vi "CPT32 Pulse Gen 3 (FPGA).vi"() -> ()   [LabVIEW 2021]
uses:
  <vilib>/rvi/Emulation/niFpgaGetClockAttributes.vi
  <vilib>/rvi/Emulation/niFpgaSctlEmulationGetInTimedLoop.vi
  <vilib>/rvi/Emulation/niFpgaEmulationReportErrorSimple.vi
  <vilib>/rvi/Emulation/niFpgaProcessEmulError.vi
  <vilib>/rvi/eio/common/nirviEmuTemplateMethod_errors.vi
  <vilib>/rvi/Emulation/niFpgaCriticalErrorInLSC.vi
  <vilib>/eio/EIOMethodNode/EIOMethodNode.xnode
  <vilib>/eio/EIONode/EIONode.xnode
panel:
  out "Array 7":fxp<+/-,37,27>[](array[numeric])
  out "Array 6":fxp<+/-,37,27>[](array[numeric])
  out "Array 5":fxp<+/-,37,27>[](array[numeric])
  out "Array 4":fxp<+/-,37,27>[](array[numeric])=[20.0, -50.0, 10.0, 20.0, 0.0, 0.0, 0.0, 0.0, 0.0, 0.0, 0.0, 0.0, 0.0, 0.0, 0.0, 0.0, 0.0, 0.0, 0.0, 0.0, 0.0, 0.0, 0.0, 0.0, 0.0, 0.0, 0.0, 0.0, 0.0, 0.0, 0.0, 0.0]
  out "Array 2":fxp<+/-,37,27>[](array[numeric])
  out "Array 1":fxp<+/-,37,27>[](array[numeric])
  out "Array 0":fxp<+/-,37,27>[](array[numeric])
  out "Array 3":fxp<+/-,37,27>[](array[numeric])=[20.0, -10.0, 50.0, -10.0, 0.0, 0.0, 0.0, 0.0, 0.0, 0.0, 0.0, 0.0, 0.0, 0.0, 0.0, 0.0]
  in  "Period (ms)":fxp<+,21,11>=160.0
  in  "DO 4":fxp<+/-,21,11>[](array[numeric])=[10.0, -10.0, 10.0, -10.0, 10.0, -10.0, 10.0, -10.0, 10.0, -10.0, 10.0, -10.0, 10.0, -10.0, 10.0, -10.0, 0.0, 0.0, 0.0, 0.0, 0.0, 0.0, 0.0, 0.0, 0.0, 0.0, 0.0, 0.0, 0.0, 0.0, 0.0, 0.0] format="%#.4g"
  in  "DO 2":fxp<+/-,21,11>[](array[numeric])=[10.0, -10.0, 10.0, -10.0, 10.0, -10.0, 10.0, -10.0, 10.0, -10.0, 10.0, -10.0, 10.0, -10.0, 10.0, -10.0] format="%#.4g"
  in  "DO 1":fxp<+/-,21,11>[](array[numeric])=[10.0, -10.0, 10.0, -10.0, 10.0, -10.0, 10.0, -10.0, 10.0, -10.0, 10.0, -10.0, 10.0, -10.0, 10.0, -10.0, 0.0, 0.0, 0.0, 0.0, 0.0, 0.0, 0.0, 0.0, 0.0, 0.0, 0.0, 0.0, 0.0, 0.0, 0.0, 0.0] format="%#.4g"
  in  "DO 3":fxp<+/-,21,11>[](array[numeric])=[0.0009765625, -10.0, -10.0, -10.0, -10.0, -10.0, -10.0, -10.0, -10.0, -10.0, -10.0, -10.0, -10.0, -10.0, -10.0, -10.0] format="%#.4g"
  in  "DO 5":fxp<+/-,21,11>[](array[numeric])=[10.0, -10.0, 10.0, -10.0, 10.0, -10.0, 10.0, -10.0, 10.0, -10.0, 10.0, -10.0, 10.0, -10.0, 10.0, -10.0, 0.0, 0.0, 0.0, 0.0, 0.0, 0.0, 0.0, 0.0, 0.0, 0.0, 0.0, 0.0, 0.0, 0.0, 0.0, 0.0] format="%#.4g"
  in  "DO 6":fxp<+/-,21,11>[](array[numeric])=[10.0, -10.0, 10.0, -10.0, 10.0, -10.0, 10.0, -10.0, 10.0, -10.0, 10.0, -10.0, 10.0, -10.0, 10.0, -10.0, 0.0, 0.0, 0.0, 0.0, 0.0, 0.0, 0.0, 0.0, 0.0, 0.0, 0.0, 0.0, 0.0, 0.0, 0.0, 0.0] format="%#.4g"
  in  "DO 7":fxp<+/-,21,11>[](array[numeric])=[10.0, -10.0, -10.0, -10.0, -10.0, -10.0, -10.0, -10.0, -10.0, -10.0, -10.0, -10.0, -10.0, -10.0, -10.0, -10.0, 0.0, 0.0, 0.0, 0.0, 0.0, 0.0, 0.0, 0.0, 0.0, 0.0, 0.0, 0.0, 0.0, 0.0, 0.0, 0.0] format="%#.4g"
  in  "DO 0":fxp<+/-,21,11>[](array[numeric])=[0.0, 0.0, 0.0, 0.0, 0.0, 0.0, 0.0, 0.0, 0.0, 0.0, 0.0, 0.0, 0.0, 0.0, 0.0, 0.0] format="%#.4g"
  out "Period (us)":fxp<+/-,37,27>
  in  "Stop":bool
  out "AO 0 t":fxp<+/-,37,27>[](array[numeric])
  in  "Start":bool
  out "AO 1 t":fxp<+/-,37,27>[](array[numeric])
  out "AO 2 t":fxp<+/-,37,27>[](array[numeric])
  out "AO 3 t":fxp<+/-,37,27>[](array[numeric])
  in  "AO 0 time":fxp<+/-,21,11>[](array[numeric])=[0.0, 0.0, 0.0, 0.0, 0.0, 0.0, 0.0, 0.0, 0.0, 0.0, 0.0, 0.0, 0.0, 0.0, 0.0, 0.0] format="%#.4g"
  in  "AO 0 voltage":fxp<+/-,32,6>[](array[numeric])=[0.0, 0.0, 0.0, 0.0, 0.0, 0.0, 0.0, 0.0, 0.0, 0.0, 0.0, 0.0, 0.0, 0.0, 0.0, 0.0]
  in  "AO 1 time":fxp<+/-,21,11>[](array[numeric])=[0.0, 0.0, 0.0, 0.0, 0.0, 0.0, 0.0, 0.0, 0.0, 0.0, 0.0, 0.0, 0.0, 0.0, 0.0, 0.0] format="%#.4g"
  in  "AO 1 voltage":fxp<+/-,32,6>[](array[numeric])=[0.0, 0.0, 0.0, 0.0, 0.0, 0.0, 0.0, 0.0, 0.0, 0.0, 0.0, 0.0, 0.0, 0.0, 0.0, 0.0]
  in  "AO 2 time":fxp<+/-,21,11>[](array[numeric])=[0.0, 0.0, 0.0, 0.0] format="%#.4g"
  in  "AO 2 voltage":fxp<+/-,32,6>[](array[numeric])=[0.0, 0.0, 0.0, 0.0]
  in  "AO 3 time":fxp<+/-,21,11>[](array[numeric])=[0.0, 0.0, 0.0, 0.0] format="%#.4g"
  in  "AO 3 voltage":fxp<+/-,32,6>[](array[numeric])=[0.0, 0.0, 0.0, 0.0]
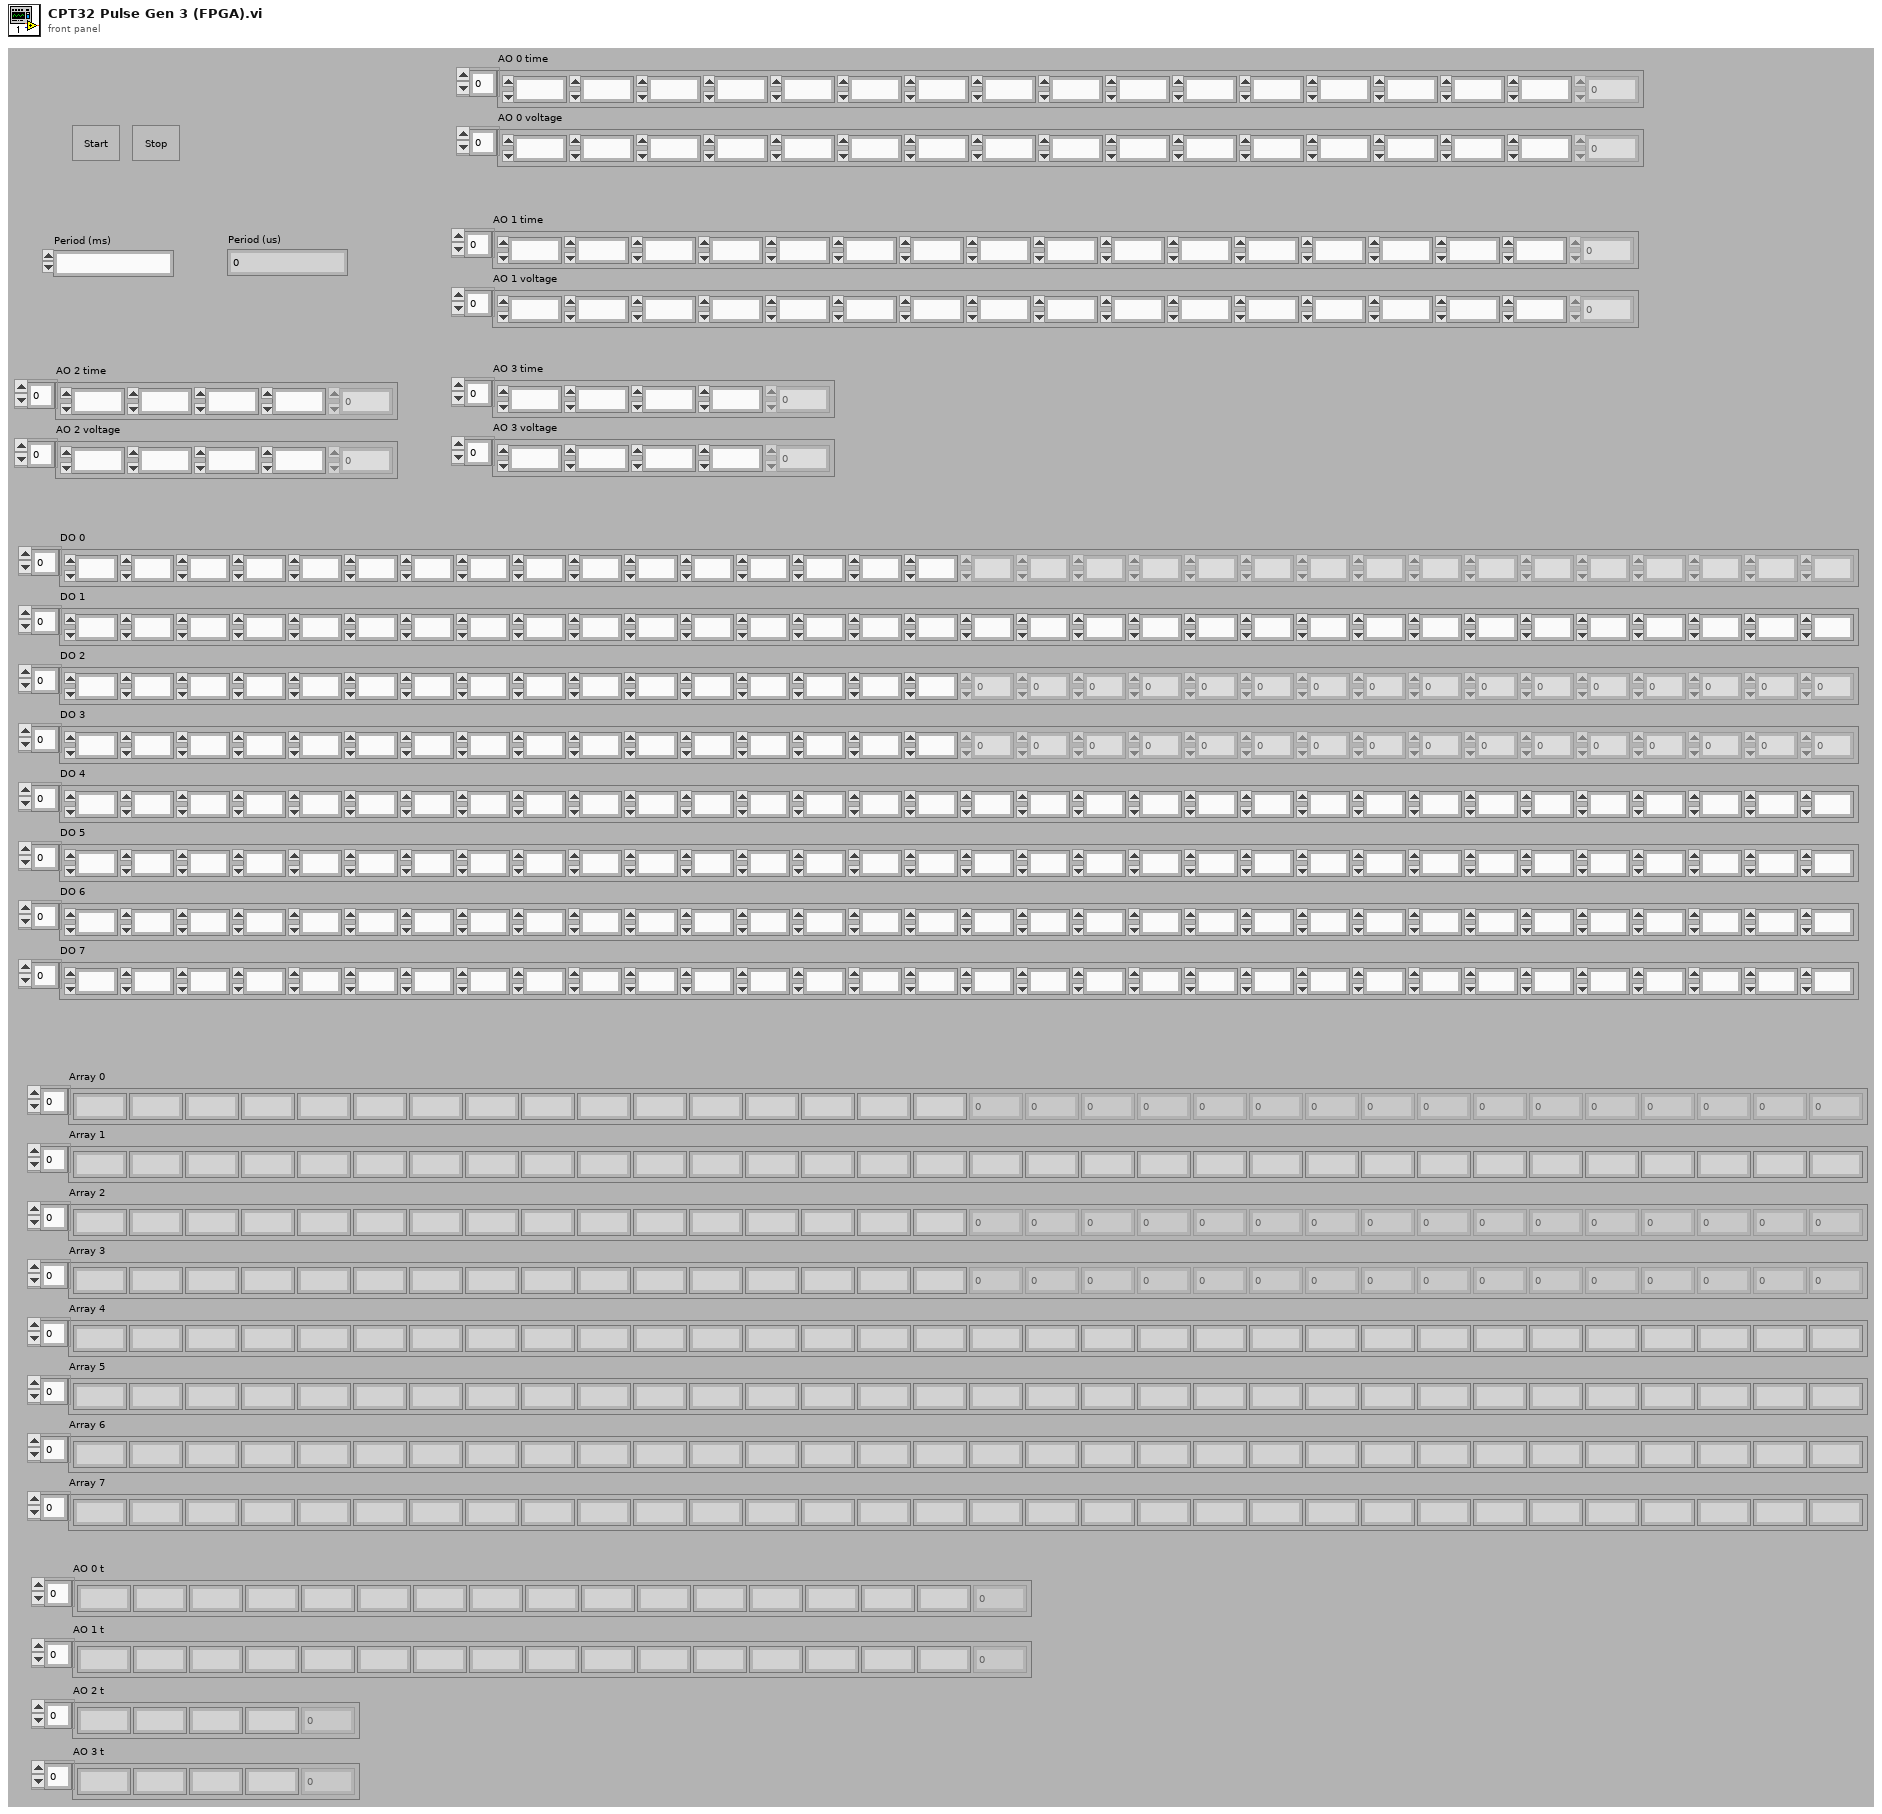
[diagram p1: front panel]
diagram:
  n1 = while {
    stop <- FALSE stop-if-true
    n2 = case shown="True" "Start" {
      frame False {
      }
      frame True {
        w4 = FALSE
        w3 = i16 0
        n3 = xnode "FPGA I/O Node"("Connector0/DIO0"=w4, "Connector0/DIO1"=w4, "Connector0/DIO2"=w4, "Connector0/DIO3"=w4, "Connector0/DIO4"=w4, "Connector0/DIO5"=w4, "Connector0/DIO6"=w4, "Connector0/DIO7"=w4, "Connector0/AO0"=w3, "Connector0/AO1"=w3, "Connector0/AO2"=w3, "Connector0/AO3"=w3) -> ()  [unwired: 12 in, 12 out]
        n4 = while {
          stop <- "Stop" stop-if-true
          n5 = Multiply(x="DO 3", y=i16 1000) -> (x*y=→"Array 3":fxp<+/-,37,27>[])
          n6 = Multiply(x="DO 4", y=i16 1000) -> (x*y=→"Array 4":fxp<+/-,37,27>[])
          n7 = Multiply(x="DO 5", y=i16 1000) -> (x*y=→"Array 5":fxp<+/-,37,27>[])
          n8 = Multiply(x="DO 6", y=i16 1000) -> (x*y=→"Array 6":fxp<+/-,37,27>[])
          n9 = Multiply(x="DO 7", y=i16 1000) -> (x*y=→"Array 7":fxp<+/-,37,27>[])
          n10 = Multiply(x="DO 0", y=i16 1000) -> (x*y=→"Array 0":fxp<+/-,37,27>[])
          n11 = Multiply(x="DO 1", y=i16 1000) -> (x*y=→"Array 1":fxp<+/-,37,27>[])
          n12 = Multiply(x="DO 2", y=i16 1000) -> (x*y=→"Array 2":fxp<+/-,37,27>[])
          n13 = Multiply(x="AO 0 time", y=i16 1000) -> (x*y=→"AO 0 t":fxp<+/-,37,27>[])
          n14 = Multiply(x="AO 3 time", y=i16 1000) -> (x*y=→"AO 3 t":fxp<+/-,37,27>[])
          n15 = Multiply(x="AO 1 time", y=i16 1000) -> (x*y=→"AO 1 t":fxp<+/-,37,27>[])
          n16 = Multiply(x="AO 2 time", y=i16 1000) -> (x*y=→"AO 2 t":fxp<+/-,37,27>[])
          n17 = Multiply(x="Period (ms)", y=i16 1000) -> (x*y=→"Period (us)":fxp<+/-,37,27>)
          n18 = flat-sequence {
            frame #0 {
              n19 = xnode "FPGA I/O Method Node"("Timeout"=-1) -> ()  [unwired: 1 in, 2 out]
            }
            frame #1 {
              n20 = local read "Period (us)"() -> (w126:fxp<+/-,37,27>)
              n21 = flat-sequence "Channel 0" {
                frame #0 {
                  # "第一段电压大小"
                  n22 = local read "AO 2 voltage"() -> (w281:fxp<+/-,32,6>[])
                  n23 = Index Array(array=w281, index=0) -> (element=w279:fxp<+/-,32,6>)
                  n24 = xnode "FPGA I/O Node"("Connector0/AO2"=w279) -> ()  [unwired: 1 in, 1 out]
                }
                frame #1 {
                  # "第一段持续时间"
                  n25 = local read "AO 2 t"() -> (w284:fxp<+/-,37,27>[])
                  n26 = Index Array(array=w284, index=0) -> (element=w282:fxp<+/-,37,27>)
                  n27 = call "Wait9"("Count(uSec)"=w282) -> ()  [unwired: 1 out]
                }
                frame #2 {
                  # "第二段电压大小"
                  n28 = local read "AO 2 voltage"() -> (w286:fxp<+/-,32,6>[])
                  n29 = Index Array(array=w286, index=1) -> (element=w285:fxp<+/-,32,6>)
                  n30 = xnode "FPGA I/O Node"("Connector0/AO2"=w285) -> ()  [unwired: 1 in, 1 out]
                }
                frame #3 {
                  # "第二段持续时间"
                  n31 = local read "AO 2 t"() -> (w289:fxp<+/-,37,27>[])
                  n32 = Index Array(array=w289, index=1) -> (element=w288:fxp<+/-,37,27>)
                  n33 = call "Wait10"("Count(uSec)"=w288) -> ()  [unwired: 1 out]
                }
                frame #4 {
                  # "第三段电压大小"
                  n34 = local read "AO 2 voltage"() -> (w292:fxp<+/-,32,6>[])
                  n35 = Index Array(array=w292, index=2) -> (element=w291:fxp<+/-,32,6>)
                  n36 = xnode "FPGA I/O Node"("Connector0/AO2"=w291) -> ()  [unwired: 1 in, 1 out]
                }
                frame #5 {
                  # "第三段持续时间"
                  n37 = local read "AO 2 t"() -> (w296:fxp<+/-,37,27>[])
                  n38 = Index Array(array=w296, index=2) -> (element=w294:fxp<+/-,37,27>)
                  n39 = call "Wait11"("Count(uSec)"=w294) -> ()  [unwired: 1 out]
                }
                frame #6 {
                  # "第四段电压大小"
                  n40 = local read "AO 2 voltage"() -> (w299:fxp<+/-,32,6>[])
                  n41 = Index Array(array=w299, index=3) -> (element=w297:fxp<+/-,32,6>)
                  n42 = xnode ("FPGA I/O Node")("Connector0/AO2"=w297) -> ()  [unwired: 1 in, 1 out]
                }
                frame #7 {
                  # "第四段持续时间"
                  n43 = local read "AO 2 t"() -> (w301:fxp<+/-,37,27>[])
                  n44 = Index Array(array=w301, index=3) -> (element=w300:fxp<+/-,37,27>)
                  n45 = call "Wait12"("Count(uSec)"=w300) -> ()  [unwired: 1 out]
                }
              }
              n46 = flat-sequence "Channel 0" {
                frame #0 {
                  # "第一段电压大小"
                  n47 = local read "AO 3 voltage"() -> (w257:fxp<+/-,32,6>[])
                  n48 = Index Array(array=w257, index=0) -> (element=w255:fxp<+/-,32,6>)
                  n49 = xnode "FPGA I/O Node"("Connector0/AO3"=w255) -> ()  [unwired: 1 in, 1 out]
                }
                frame #1 {
                  # "第一段持续时间"
                  n50 = local read "AO 3 t"() -> (w260:fxp<+/-,37,27>[])
                  n51 = Index Array(array=w260, index=0) -> (element=w258:fxp<+/-,37,27>)
                  n52 = call "Wait13"("Count(uSec)"=w258) -> ()  [unwired: 1 out]
                }
                frame #2 {
                  # "第二段电压大小"
                  n53 = local read "AO 3 voltage"() -> (w262:fxp<+/-,32,6>[])
                  n54 = Index Array(array=w262, index=1) -> (element=w261:fxp<+/-,32,6>)
                  n55 = xnode "FPGA I/O Node"("Connector0/AO3"=w261) -> ()  [unwired: 1 in, 1 out]
                }
                frame #3 {
                  # "第二段持续时间"
                  n56 = local read "AO 3 t"() -> (w265:fxp<+/-,37,27>[])
                  n57 = Index Array(array=w265, index=1) -> (element=w264:fxp<+/-,37,27>)
                  n58 = call "Wait14"("Count(uSec)"=w264) -> ()  [unwired: 1 out]
                }
                frame #4 {
                  # "第三段电压大小"
                  n59 = local read "AO 3 voltage"() -> (w268:fxp<+/-,32,6>[])
                  n60 = Index Array(array=w268, index=2) -> (element=w267:fxp<+/-,32,6>)
                  n61 = xnode "FPGA I/O Node"("Connector0/AO3"=w267) -> ()  [unwired: 1 in, 1 out]
                }
                frame #5 {
                  # "第三段持续时间"
                  n62 = local read "AO 3 t"() -> (w272:fxp<+/-,37,27>[])
                  n63 = Index Array(array=w272, index=2) -> (element=w270:fxp<+/-,37,27>)
                  n64 = call "Wait15"("Count(uSec)"=w270) -> ()  [unwired: 1 out]
                }
                frame #6 {
                  # "第四段电压大小"
                  n65 = local read "AO 3 voltage"() -> (w275:fxp<+/-,32,6>[])
                  n66 = Index Array(array=w275, index=3) -> (element=w273:fxp<+/-,32,6>)
                  n67 = xnode ("FPGA I/O Node")("Connector0/AO3"=w273) -> ()  [unwired: 1 in, 1 out]
                }
                frame #7 {
                  # "第四段持续时间"
                  n68 = local read "AO 3 t"() -> (w277:fxp<+/-,37,27>[])
                  n69 = Index Array(array=w277, index=3) -> (element=w276:fxp<+/-,37,27>)
                  n70 = call "Wait16"("Count(uSec)"=w276) -> ()  [unwired: 1 out]
                }
              }
              n71 = flat-sequence "Channel 3" {
                tunnel: [w1648] -> w254
                tunnel: w254 -> [w1652]
                tunnel: [w1653] -> w253
                tunnel: w253 -> [w1658]
                tunnel: [w1660] -> w252
                tunnel: w252 -> [w1664]
                tunnel: [w1666] -> w251
                tunnel: w251 -> [w1670]
                tunnel: [w1672] -> w250
                tunnel: w250 -> [w1676]
                tunnel: [w1678] -> w249
                tunnel: w249 -> [w1682]
                tunnel: [w1684] -> w248
                tunnel: w248 -> [w1688]
                tunnel: [w1690] -> w247
                tunnel: w247 -> [w1694]
                tunnel: [w1695] -> w246
                tunnel: w246 -> [w1700]
                tunnel: [w1701] -> w245
                tunnel: w245 -> [w1706]
                tunnel: [w1708] -> w244
                tunnel: w244 -> [w1712]
                tunnel: [w1714] -> w243
                tunnel: w243 -> [w1718]
                tunnel: [w1720] -> w242
                tunnel: w242 -> [w1724]
                tunnel: [w1726] -> w241
                tunnel: w241 -> [w1730]
                tunnel: [w1732] -> w240
                tunnel: w240 -> [w1736]
                tunnel: [w1738] -> w239
                tunnel: w239 -> [w1742]
                frame #0 {
                  # "起始电平"
                  n72 = local read "Array 0"() -> (w1650:fxp<+/-,37,27>[])
                  n73 = Index Array(array=w1650, index=0) -> (element=w1648:fxp<+/-,37,27>)
                  n74 = Greater Than 0?(x=w1648) -> (x > 0?=w1647:bool)
                  n75 = xnode "FPGA I/O Node"("Connector0/DIO0"=w1647) -> ()  [unwired: 1 in, 1 out]
                }
                frame #1 {
                  # "第一段持续时间"
                  n76 = Absolute Value(x=w1652) -> (abs(x)=w1651:fxp<+,36,26>)
                  n77 = call "Wait17"("Count(uSec)"=w1651) -> ()  [unwired: 1 out]
                }
                frame #2 {
                  n78 = local read "Array 0"() -> (w1656:fxp<+/-,37,27>[])
                  n79 = Index Array(array=w1656, index=1) -> (element=w1653:fxp<+/-,37,27>)
                  n80 = Greater Than 0?(x=w1653) -> (x > 0?=w1654:bool)
                  n81 = xnode "FPGA I/O Node"("Connector0/DIO0"=w1654) -> ()  [unwired: 1 in, 1 out]
                }
                frame #3 {
                  n82 = Absolute Value(x=w1658) -> (abs(x)=w1657:fxp<+,36,26>)
                  n83 = call "Wait18"("Count(uSec)"=w1657) -> ()  [unwired: 1 out]
                }
                frame #4 {
                  n84 = local read "Array 0"() -> (w1662:fxp<+/-,37,27>[])
                  n85 = Index Array(array=w1662, index=2) -> (element=w1660:fxp<+/-,37,27>)
                  n86 = Greater Than 0?(x=w1660) -> (x > 0?=w1659:bool)
                  n87 = xnode "FPGA I/O Node"("Connector0/DIO0"=w1659) -> ()  [unwired: 1 in, 1 out]
                }
                frame #5 {
                  n88 = Absolute Value(x=w1664) -> (abs(x)=w1663:fxp<+,36,26>)
                  n89 = call "Wait19"("Count(uSec)"=w1663) -> ()  [unwired: 1 out]
                }
                frame #6 {
                  n90 = local read "Array 0"() -> (w1668:fxp<+/-,37,27>[])
                  n91 = Index Array(array=w1668, index=3) -> (element=w1666:fxp<+/-,37,27>)
                  n92 = Greater Than 0?(x=w1666) -> (x > 0?=w1665:bool)
                  n93 = xnode ("FPGA I/O Node")("Connector0/DIO0"=w1665) -> ()  [unwired: 1 in, 1 out]
                }
                frame #7 {
                  n94 = Absolute Value(x=w1670) -> (abs(x)=w1669:fxp<+,36,26>)
                  n95 = call "Wait20"("Count(uSec)"=w1669) -> ()  [unwired: 1 out]
                }
                frame #8 {
                  # "低"
                  n96 = local read "Array 0"() -> (w1674:fxp<+/-,37,27>[])
                  n97 = Index Array(array=w1674, index=4) -> (element=w1672:fxp<+/-,37,27>)
                  n98 = Greater Than 0?(x=w1672) -> (x > 0?=w1671:bool)
                  n99 = xnode "FPGA I/O Node"("Connector0/DIO0"=w1671) -> ()  [unwired: 1 in, 1 out]
                }
                frame #9 {
                  n100 = Absolute Value(x=w1676) -> (abs(x)=w1675:fxp<+,36,26>)
                  n101 = call "Wait21"("Count(uSec)"=w1675) -> ()  [unwired: 1 out]
                }
                frame #10 {
                  # "高"
                  n102 = local read "Array 0"() -> (w1680:fxp<+/-,37,27>[])
                  n103 = Index Array(array=w1680, index=5) -> (element=w1678:fxp<+/-,37,27>)
                  n104 = Greater Than 0?(x=w1678) -> (x > 0?=w1677:bool)
                  n105 = xnode "FPGA I/O Node"("Connector0/DIO0"=w1677) -> ()  [unwired: 1 in, 1 out]
                }
                frame #11 {
                  n106 = Absolute Value(x=w1682) -> (abs(x)=w1681:fxp<+,36,26>)
                  n107 = call "Wait22"("Count(uSec)"=w1681) -> ()  [unwired: 1 out]
                }
                frame #12 {
                  # "低"
                  n108 = local read "Array 0"() -> (w1686:fxp<+/-,37,27>[])
                  n109 = Index Array(array=w1686, index=6) -> (element=w1684:fxp<+/-,37,27>)
                  n110 = Greater Than 0?(x=w1684) -> (x > 0?=w1683:bool)
                  n111 = xnode "FPGA I/O Node"("Connector0/DIO0"=w1683) -> ()  [unwired: 1 in, 1 out]
                }
                frame #13 {
                  n112 = Absolute Value(x=w1688) -> (abs(x)=w1687:fxp<+,36,26>)
                  n113 = call "Wait23"("Count(uSec)"=w1687) -> ()  [unwired: 1 out]
                }
                frame #14 {
                  n114 = local read "Array 0"() -> (w1692:fxp<+/-,37,27>[])
                  n115 = Index Array(array=w1692, index=7) -> (element=w1690:fxp<+/-,37,27>)
                  n116 = Greater Than 0?(x=w1690) -> (x > 0?=w1689:bool)
                  n117 = xnode "FPGA I/O Node"("Connector0/DIO0"=w1689) -> ()  [unwired: 1 in, 1 out]
                }
                frame #15 {
                  n118 = Absolute Value(x=w1694) -> (abs(x)=w1693:fxp<+,36,26>)
                  n119 = call "Wait24"("Count(uSec)"=w1693) -> ()  [unwired: 1 out]
                }
                frame #16 {
                  n120 = local read "Array 0"() -> (w1698:fxp<+/-,37,27>[])
                  n121 = Index Array(array=w1698, index=8) -> (element=w1695:fxp<+/-,37,27>)
                  n122 = Greater Than 0?(x=w1695) -> (x > 0?=w1696:bool)
                  n123 = xnode "FPGA I/O Node"("Connector0/DIO0"=w1696) -> ()  [unwired: 1 in, 1 out]
                }
                frame #17 {
                  n124 = Absolute Value(x=w1700) -> (abs(x)=w1699:fxp<+,36,26>)
                  n125 = call "Wait25"("Count(uSec)"=w1699) -> ()  [unwired: 1 out]
                }
                frame #18 {
                  n126 = local read "Array 0"() -> (w1704:fxp<+/-,37,27>[])
                  n127 = Index Array(array=w1704, index=9) -> (element=w1701:fxp<+/-,37,27>)
                  n128 = Greater Than 0?(x=w1701) -> (x > 0?=w1702:bool)
                  n129 = xnode "FPGA I/O Node"("Connector0/DIO0"=w1702) -> ()  [unwired: 1 in, 1 out]
                }
                frame #19 {
                  n130 = Absolute Value(x=w1706) -> (abs(x)=w1705:fxp<+,36,26>)
                  n131 = call "Wait26"("Count(uSec)"=w1705) -> ()  [unwired: 1 out]
                }
                frame #20 {
                  # "低"
                  n132 = local read "Array 0"() -> (w1710:fxp<+/-,37,27>[])
                  n133 = Index Array(array=w1710, index=10) -> (element=w1708:fxp<+/-,37,27>)
                  n134 = Greater Than 0?(x=w1708) -> (x > 0?=w1707:bool)
                  n135 = xnode "FPGA I/O Node"("Connector0/DIO0"=w1707) -> ()  [unwired: 1 in, 1 out]
                }
                frame #21 {
                  n136 = Absolute Value(x=w1712) -> (abs(x)=w1711:fxp<+,36,26>)
                  n137 = call "Wait27"("Count(uSec)"=w1711) -> ()  [unwired: 1 out]
                }
                frame #22 {
                  # "高"
                  n138 = local read "Array 0"() -> (w1716:fxp<+/-,37,27>[])
                  n139 = Index Array(array=w1716, index=11) -> (element=w1714:fxp<+/-,37,27>)
                  n140 = Greater Than 0?(x=w1714) -> (x > 0?=w1713:bool)
                  n141 = xnode "FPGA I/O Node"("Connector0/DIO0"=w1713) -> ()  [unwired: 1 in, 1 out]
                }
                frame #23 {
                  n142 = Absolute Value(x=w1718) -> (abs(x)=w1717:fxp<+,36,26>)
                  n143 = call "Wait28"("Count(uSec)"=w1717) -> ()  [unwired: 1 out]
                }
                frame #24 {
                  # "低"
                  n144 = local read "Array 0"() -> (w1722:fxp<+/-,37,27>[])
                  n145 = Index Array(array=w1722, index=12) -> (element=w1720:fxp<+/-,37,27>)
                  n146 = Greater Than 0?(x=w1720) -> (x > 0?=w1719:bool)
                  n147 = xnode "FPGA I/O Node"("Connector0/DIO0"=w1719) -> ()  [unwired: 1 in, 1 out]
                }
                frame #25 {
                  n148 = Absolute Value(x=w1724) -> (abs(x)=w1723:fxp<+,36,26>)
                  n149 = call "Wait29"("Count(uSec)"=w1723) -> ()  [unwired: 1 out]
                }
                frame #26 {
                  # "高"
                  n150 = local read "Array 0"() -> (w1728:fxp<+/-,37,27>[])
                  n151 = Index Array(array=w1728, index=13) -> (element=w1726:fxp<+/-,37,27>)
                  n152 = Greater Than 0?(x=w1726) -> (x > 0?=w1725:bool)
                  n153 = xnode "FPGA I/O Node"("Connector0/DIO0"=w1725) -> ()  [unwired: 1 in, 1 out]
                }
                frame #27 {
                  n154 = Absolute Value(x=w1730) -> (abs(x)=w1729:fxp<+,36,26>)
                  n155 = call "Wait30"("Count(uSec)"=w1729) -> ()  [unwired: 1 out]
                }
                frame #28 {
                  # "低"
                  n156 = local read "Array 0"() -> (w1734:fxp<+/-,37,27>[])
                  n157 = Index Array(array=w1734, index=14) -> (element=w1732:fxp<+/-,37,27>)
                  n158 = Greater Than 0?(x=w1732) -> (x > 0?=w1731:bool)
                  n159 = xnode "FPGA I/O Node"("Connector0/DIO0"=w1731) -> ()  [unwired: 1 in, 1 out]
                }
                frame #29 {
                  n160 = Absolute Value(x=w1736) -> (abs(x)=w1735:fxp<+,36,26>)
                  n161 = call "Wait31"("Count(uSec)"=w1735) -> ()  [unwired: 1 out]
                }
                frame #30 {
                  n162 = local read "Array 0"() -> (w1740:fxp<+/-,37,27>[])
                  n163 = Index Array(array=w1740, index=15) -> (element=w1738:fxp<+/-,37,27>)
                  n164 = Greater Than 0?(x=w1738) -> (x > 0?=w1737:bool)
                  n165 = xnode "FPGA I/O Node"("Connector0/DIO0"=w1737) -> ()  [unwired: 1 in, 1 out]
                }
                frame #31 {
                  n166 = Absolute Value(x=w1742) -> (abs(x)=w1741:fxp<+,36,26>)
                  n167 = call "Wait32"("Count(uSec)"=w1741) -> ()  [unwired: 1 out]
                }
              }
              n168 = flat-sequence "Channel 3" {
                tunnel: [w1360] -> w222
                tunnel: w222 -> [w1364]
                tunnel: [w1365] -> w221
                tunnel: w221 -> [w1370]
                tunnel: [w1372] -> w220
                tunnel: w220 -> [w1376]
                tunnel: [w1378] -> w219
                tunnel: w219 -> [w1382]
                tunnel: [w1384] -> w218
                tunnel: w218 -> [w1388]
                tunnel: [w1390] -> w217
                tunnel: w217 -> [w1394]
                tunnel: [w1396] -> w216
                tunnel: w216 -> [w1400]
                tunnel: [w1402] -> w215
                tunnel: w215 -> [w1406]
                tunnel: [w1407] -> w214
                tunnel: w214 -> [w1412]
                tunnel: [w1413] -> w213
                tunnel: w213 -> [w1418]
                tunnel: [w1420] -> w212
                tunnel: w212 -> [w1424]
                tunnel: [w1426] -> w211
                tunnel: w211 -> [w1430]
                tunnel: [w1432] -> w210
                tunnel: w210 -> [w1436]
                tunnel: [w1438] -> w209
                tunnel: w209 -> [w1442]
                tunnel: [w1444] -> w208
                tunnel: w208 -> [w1448]
                tunnel: [w1450] -> w207
                tunnel: w207 -> [w1454]
                frame #0 {
                  # "起始电平"
                  n169 = local read "Array 2"() -> (w1362:fxp<+/-,37,27>[])
                  n170 = Index Array(array=w1362, index=0) -> (element=w1360:fxp<+/-,37,27>)
                  n171 = Greater Than 0?(x=w1360) -> (x > 0?=w1359:bool)
                  n172 = xnode "FPGA I/O Node"("Connector0/DIO2"=w1359) -> ()  [unwired: 1 in, 1 out]
                }
                frame #1 {
                  # "第一段持续时间"
                  n173 = Absolute Value(x=w1364) -> (abs(x)=w1363:fxp<+,36,26>)
                  n174 = call "Wait49"("Count(uSec)"=w1363) -> ()  [unwired: 1 out]
                }
                frame #2 {
                  n175 = local read "Array 2"() -> (w1368:fxp<+/-,37,27>[])
                  n176 = Index Array(array=w1368, index=1) -> (element=w1365:fxp<+/-,37,27>)
                  n177 = Greater Than 0?(x=w1365) -> (x > 0?=w1366:bool)
                  n178 = xnode "FPGA I/O Node"("Connector0/DIO2"=w1366) -> ()  [unwired: 1 in, 1 out]
                }
                frame #3 {
                  n179 = Absolute Value(x=w1370) -> (abs(x)=w1369:fxp<+,36,26>)
                  n180 = call "Wait50"("Count(uSec)"=w1369) -> ()  [unwired: 1 out]
                }
                frame #4 {
                  n181 = local read "Array 2"() -> (w1374:fxp<+/-,37,27>[])
                  n182 = Index Array(array=w1374, index=2) -> (element=w1372:fxp<+/-,37,27>)
                  n183 = Greater Than 0?(x=w1372) -> (x > 0?=w1371:bool)
                  n184 = xnode "FPGA I/O Node"("Connector0/DIO2"=w1371) -> ()  [unwired: 1 in, 1 out]
                }
                frame #5 {
                  n185 = Absolute Value(x=w1376) -> (abs(x)=w1375:fxp<+,36,26>)
                  n186 = call "Wait51"("Count(uSec)"=w1375) -> ()  [unwired: 1 out]
                }
                frame #6 {
                  n187 = local read "Array 2"() -> (w1380:fxp<+/-,37,27>[])
                  n188 = Index Array(array=w1380, index=3) -> (element=w1378:fxp<+/-,37,27>)
                  n189 = Greater Than 0?(x=w1378) -> (x > 0?=w1377:bool)
                  n190 = xnode ("FPGA I/O Node")("Connector0/DIO2"=w1377) -> ()  [unwired: 1 in, 1 out]
                }
                frame #7 {
                  n191 = Absolute Value(x=w1382) -> (abs(x)=w1381:fxp<+,36,26>)
                  n192 = call "Wait52"("Count(uSec)"=w1381) -> ()  [unwired: 1 out]
                }
                frame #8 {
                  # "低"
                  n193 = local read "Array 2"() -> (w1386:fxp<+/-,37,27>[])
                  n194 = Index Array(array=w1386, index=4) -> (element=w1384:fxp<+/-,37,27>)
                  n195 = Greater Than 0?(x=w1384) -> (x > 0?=w1383:bool)
                  n196 = xnode "FPGA I/O Node"("Connector0/DIO2"=w1383) -> ()  [unwired: 1 in, 1 out]
                }
                frame #9 {
                  n197 = Absolute Value(x=w1388) -> (abs(x)=w1387:fxp<+,36,26>)
                  n198 = call "Wait53"("Count(uSec)"=w1387) -> ()  [unwired: 1 out]
                }
                frame #10 {
                  # "高"
                  n199 = local read "Array 2"() -> (w1392:fxp<+/-,37,27>[])
                  n200 = Index Array(array=w1392, index=5) -> (element=w1390:fxp<+/-,37,27>)
                  n201 = Greater Than 0?(x=w1390) -> (x > 0?=w1389:bool)
                  n202 = xnode "FPGA I/O Node"("Connector0/DIO2"=w1389) -> ()  [unwired: 1 in, 1 out]
                }
                frame #11 {
                  n203 = Absolute Value(x=w1394) -> (abs(x)=w1393:fxp<+,36,26>)
                  n204 = call "Wait54"("Count(uSec)"=w1393) -> ()  [unwired: 1 out]
                }
                frame #12 {
                  # "低"
                  n205 = local read "Array 2"() -> (w1398:fxp<+/-,37,27>[])
                  n206 = Index Array(array=w1398, index=6) -> (element=w1396:fxp<+/-,37,27>)
                  n207 = Greater Than 0?(x=w1396) -> (x > 0?=w1395:bool)
                  n208 = xnode "FPGA I/O Node"("Connector0/DIO2"=w1395) -> ()  [unwired: 1 in, 1 out]
                }
                frame #13 {
                  n209 = Absolute Value(x=w1400) -> (abs(x)=w1399:fxp<+,36,26>)
                  n210 = call "Wait55"("Count(uSec)"=w1399) -> ()  [unwired: 1 out]
                }
                frame #14 {
                  n211 = local read "Array 2"() -> (w1404:fxp<+/-,37,27>[])
                  n212 = Index Array(array=w1404, index=7) -> (element=w1402:fxp<+/-,37,27>)
                  n213 = Greater Than 0?(x=w1402) -> (x > 0?=w1401:bool)
                  n214 = xnode "FPGA I/O Node"("Connector0/DIO2"=w1401) -> ()  [unwired: 1 in, 1 out]
                }
                frame #15 {
                  n215 = Absolute Value(x=w1406) -> (abs(x)=w1405:fxp<+,36,26>)
                  n216 = call "Wait56"("Count(uSec)"=w1405) -> ()  [unwired: 1 out]
                }
                frame #16 {
                  n217 = local read "Array 2"() -> (w1410:fxp<+/-,37,27>[])
                  n218 = Index Array(array=w1410, index=8) -> (element=w1407:fxp<+/-,37,27>)
                  n219 = Greater Than 0?(x=w1407) -> (x > 0?=w1408:bool)
                  n220 = xnode "FPGA I/O Node"("Connector0/DIO2"=w1408) -> ()  [unwired: 1 in, 1 out]
                }
                frame #17 {
                  n221 = Absolute Value(x=w1412) -> (abs(x)=w1411:fxp<+,36,26>)
                  n222 = call "Wait57"("Count(uSec)"=w1411) -> ()  [unwired: 1 out]
                }
                frame #18 {
                  n223 = local read "Array 2"() -> (w1416:fxp<+/-,37,27>[])
                  n224 = Index Array(array=w1416, index=9) -> (element=w1413:fxp<+/-,37,27>)
                  n225 = Greater Than 0?(x=w1413) -> (x > 0?=w1414:bool)
                  n226 = xnode "FPGA I/O Node"("Connector0/DIO2"=w1414) -> ()  [unwired: 1 in, 1 out]
                }
                frame #19 {
                  n227 = Absolute Value(x=w1418) -> (abs(x)=w1417:fxp<+,36,26>)
                  n228 = call "Wait58"("Count(uSec)"=w1417) -> ()  [unwired: 1 out]
                }
                frame #20 {
                  # "低"
                  n229 = local read "Array 2"() -> (w1422:fxp<+/-,37,27>[])
                  n230 = Index Array(array=w1422, index=10) -> (element=w1420:fxp<+/-,37,27>)
                  n231 = Greater Than 0?(x=w1420) -> (x > 0?=w1419:bool)
                  n232 = xnode "FPGA I/O Node"("Connector0/DIO2"=w1419) -> ()  [unwired: 1 in, 1 out]
                }
                frame #21 {
                  n233 = Absolute Value(x=w1424) -> (abs(x)=w1423:fxp<+,36,26>)
                  n234 = call "Wait59"("Count(uSec)"=w1423) -> ()  [unwired: 1 out]
                }
                frame #22 {
                  # "高"
                  n235 = local read "Array 2"() -> (w1428:fxp<+/-,37,27>[])
                  n236 = Index Array(array=w1428, index=11) -> (element=w1426:fxp<+/-,37,27>)
                  n237 = Greater Than 0?(x=w1426) -> (x > 0?=w1425:bool)
                  n238 = xnode "FPGA I/O Node"("Connector0/DIO2"=w1425) -> ()  [unwired: 1 in, 1 out]
                }
                frame #23 {
                  n239 = Absolute Value(x=w1430) -> (abs(x)=w1429:fxp<+,36,26>)
                  n240 = call "Wait60"("Count(uSec)"=w1429) -> ()  [unwired: 1 out]
                }
                frame #24 {
                  # "低"
                  n241 = local read "Array 2"() -> (w1434:fxp<+/-,37,27>[])
                  n242 = Index Array(array=w1434, index=12) -> (element=w1432:fxp<+/-,37,27>)
                  n243 = Greater Than 0?(x=w1432) -> (x > 0?=w1431:bool)
                  n244 = xnode "FPGA I/O Node"("Connector0/DIO2"=w1431) -> ()  [unwired: 1 in, 1 out]
                }
                frame #25 {
                  n245 = Absolute Value(x=w1436) -> (abs(x)=w1435:fxp<+,36,26>)
                  n246 = call "Wait61"("Count(uSec)"=w1435) -> ()  [unwired: 1 out]
                }
                frame #26 {
                  # "高"
                  n247 = local read "Array 2"() -> (w1440:fxp<+/-,37,27>[])
                  n248 = Index Array(array=w1440, index=13) -> (element=w1438:fxp<+/-,37,27>)
                  n249 = Greater Than 0?(x=w1438) -> (x > 0?=w1437:bool)
                  n250 = xnode "FPGA I/O Node"("Connector0/DIO2"=w1437) -> ()  [unwired: 1 in, 1 out]
                }
                frame #27 {
                  n251 = Absolute Value(x=w1442) -> (abs(x)=w1441:fxp<+,36,26>)
                  n252 = call "Wait62"("Count(uSec)"=w1441) -> ()  [unwired: 1 out]
                }
                frame #28 {
                  # "低"
                  n253 = local read "Array 2"() -> (w1446:fxp<+/-,37,27>[])
                  n254 = Index Array(array=w1446, index=14) -> (element=w1444:fxp<+/-,37,27>)
                  n255 = Greater Than 0?(x=w1444) -> (x > 0?=w1443:bool)
                  n256 = xnode "FPGA I/O Node"("Connector0/DIO2"=w1443) -> ()  [unwired: 1 in, 1 out]
                }
                frame #29 {
                  n257 = Absolute Value(x=w1448) -> (abs(x)=w1447:fxp<+,36,26>)
                  n258 = call "Wait63"("Count(uSec)"=w1447) -> ()  [unwired: 1 out]
                }
                frame #30 {
                  n259 = local read "Array 2"() -> (w1452:fxp<+/-,37,27>[])
                  n260 = Index Array(array=w1452, index=15) -> (element=w1450:fxp<+/-,37,27>)
                  n261 = Greater Than 0?(x=w1450) -> (x > 0?=w1449:bool)
                  n262 = xnode "FPGA I/O Node"("Connector0/DIO2"=w1449) -> ()  [unwired: 1 in, 1 out]
                }
                frame #31 {
                  n263 = Absolute Value(x=w1454) -> (abs(x)=w1453:fxp<+,36,26>)
                  n264 = call "Wait64"("Count(uSec)"=w1453) -> ()  [unwired: 1 out]
                }
              }
              n265 = flat-sequence "Channel 3" {
                tunnel: [w1264] -> w206
                tunnel: w206 -> [w1268]
                tunnel: [w1269] -> w205
                tunnel: w205 -> [w1274]
                tunnel: [w1276] -> w204
                tunnel: w204 -> [w1280]
                tunnel: [w1282] -> w203
                tunnel: w203 -> [w1286]
                tunnel: [w1288] -> w202
                tunnel: w202 -> [w1292]
                tunnel: [w1294] -> w201
                tunnel: w201 -> [w1298]
                tunnel: [w1300] -> w200
                tunnel: w200 -> [w1304]
                tunnel: [w1306] -> w199
                tunnel: w199 -> [w1310]
                tunnel: [w1311] -> w198
                tunnel: w198 -> [w1316]
                tunnel: [w1317] -> w197
                tunnel: w197 -> [w1322]
                tunnel: [w1324] -> w196
                tunnel: w196 -> [w1328]
                tunnel: [w1330] -> w195
                tunnel: w195 -> [w1334]
                tunnel: [w1336] -> w194
                tunnel: w194 -> [w1340]
                tunnel: [w1342] -> w193
                tunnel: w193 -> [w1346]
                tunnel: [w1348] -> w192
                tunnel: w192 -> [w1352]
                tunnel: [w1354] -> w191
                tunnel: w191 -> [w1358]
                frame #0 {
                  # "起始电平"
                  n266 = local read "Array 3"() -> (w1266:fxp<+/-,37,27>[])
                  n267 = Index Array(array=w1266, index=0) -> (element=w1264:fxp<+/-,37,27>)
                  n268 = Greater Than 0?(x=w1264) -> (x > 0?=w1263:bool)
                  n269 = xnode "FPGA I/O Node"("Connector0/DIO3"=w1263) -> ()  [unwired: 1 in, 1 out]
                }
                frame #1 {
                  # "第一段持续时间"
                  n270 = Absolute Value(x=w1268) -> (abs(x)=w1267:fxp<+,36,26>)
                  n271 = call "Wait65"("Count(uSec)"=w1267) -> ()  [unwired: 1 out]
                }
                frame #2 {
                  n272 = local read "Array 3"() -> (w1272:fxp<+/-,37,27>[])
                  n273 = Index Array(array=w1272, index=1) -> (element=w1269:fxp<+/-,37,27>)
                  n274 = Greater Than 0?(x=w1269) -> (x > 0?=w1270:bool)
                  n275 = xnode "FPGA I/O Node"("Connector0/DIO3"=w1270) -> ()  [unwired: 1 in, 1 out]
                }
                frame #3 {
                  n276 = Absolute Value(x=w1274) -> (abs(x)=w1273:fxp<+,36,26>)
                  n277 = call "Wait66"("Count(uSec)"=w1273) -> ()  [unwired: 1 out]
                }
                frame #4 {
                  n278 = local read "Array 3"() -> (w1278:fxp<+/-,37,27>[])
                  n279 = Index Array(array=w1278, index=2) -> (element=w1276:fxp<+/-,37,27>)
                  n280 = Greater Than 0?(x=w1276) -> (x > 0?=w1275:bool)
                  n281 = xnode "FPGA I/O Node"("Connector0/DIO3"=w1275) -> ()  [unwired: 1 in, 1 out]
                }
                frame #5 {
                  n282 = Absolute Value(x=w1280) -> (abs(x)=w1279:fxp<+,36,26>)
                  n283 = call "Wait67"("Count(uSec)"=w1279) -> ()  [unwired: 1 out]
                }
                frame #6 {
                  n284 = local read "Array 3"() -> (w1284:fxp<+/-,37,27>[])
                  n285 = Index Array(array=w1284, index=3) -> (element=w1282:fxp<+/-,37,27>)
                  n286 = Greater Than 0?(x=w1282) -> (x > 0?=w1281:bool)
                  n287 = xnode ("FPGA I/O Node")("Connector0/DIO3"=w1281) -> ()  [unwired: 1 in, 1 out]
                }
                frame #7 {
                  n288 = Absolute Value(x=w1286) -> (abs(x)=w1285:fxp<+,36,26>)
                  n289 = call "Wait68"("Count(uSec)"=w1285) -> ()  [unwired: 1 out]
                }
                frame #8 {
                  # "低"
                  n290 = local read "Array 3"() -> (w1290:fxp<+/-,37,27>[])
                  n291 = Index Array(array=w1290, index=4) -> (element=w1288:fxp<+/-,37,27>)
                  n292 = Greater Than 0?(x=w1288) -> (x > 0?=w1287:bool)
                  n293 = xnode "FPGA I/O Node"("Connector0/DIO3"=w1287) -> ()  [unwired: 1 in, 1 out]
                }
                frame #9 {
                  n294 = Absolute Value(x=w1292) -> (abs(x)=w1291:fxp<+,36,26>)
                  n295 = call "Wait69"("Count(uSec)"=w1291) -> ()  [unwired: 1 out]
                }
                frame #10 {
                  # "高"
                  n296 = local read "Array 3"() -> (w1296:fxp<+/-,37,27>[])
                  n297 = Index Array(array=w1296, index=5) -> (element=w1294:fxp<+/-,37,27>)
                  n298 = Greater Than 0?(x=w1294) -> (x > 0?=w1293:bool)
                  n299 = xnode "FPGA I/O Node"("Connector0/DIO3"=w1293) -> ()  [unwired: 1 in, 1 out]
                }
                frame #11 {
                  n300 = Absolute Value(x=w1298) -> (abs(x)=w1297:fxp<+,36,26>)
                  n301 = call "Wait70"("Count(uSec)"=w1297) -> ()  [unwired: 1 out]
                }
                frame #12 {
                  # "低"
                  n302 = local read "Array 3"() -> (w1302:fxp<+/-,37,27>[])
                  n303 = Index Array(array=w1302, index=6) -> (element=w1300:fxp<+/-,37,27>)
                  n304 = Greater Than 0?(x=w1300) -> (x > 0?=w1299:bool)
                  n305 = xnode "FPGA I/O Node"("Connector0/DIO3"=w1299) -> ()  [unwired: 1 in, 1 out]
                }
                frame #13 {
                  n306 = Absolute Value(x=w1304) -> (abs(x)=w1303:fxp<+,36,26>)
                  n307 = call "Wait71"("Count(uSec)"=w1303) -> ()  [unwired: 1 out]
                }
                frame #14 {
                  n308 = local read "Array 3"() -> (w1308:fxp<+/-,37,27>[])
                  n309 = Index Array(array=w1308, index=7) -> (element=w1306:fxp<+/-,37,27>)
                  n310 = Greater Than 0?(x=w1306) -> (x > 0?=w1305:bool)
                  n311 = xnode "FPGA I/O Node"("Connector0/DIO3"=w1305) -> ()  [unwired: 1 in, 1 out]
                }
                frame #15 {
                  n312 = Absolute Value(x=w1310) -> (abs(x)=w1309:fxp<+,36,26>)
                  n313 = call "Wait72"("Count(uSec)"=w1309) -> ()  [unwired: 1 out]
                }
                frame #16 {
                  n314 = local read "Array 3"() -> (w1314:fxp<+/-,37,27>[])
                  n315 = Index Array(array=w1314, index=8) -> (element=w1311:fxp<+/-,37,27>)
                  n316 = Greater Than 0?(x=w1311) -> (x > 0?=w1312:bool)
                  n317 = xnode "FPGA I/O Node"("Connector0/DIO3"=w1312) -> ()  [unwired: 1 in, 1 out]
                }
                frame #17 {
                  n318 = Absolute Value(x=w1316) -> (abs(x)=w1315:fxp<+,36,26>)
                  n319 = call "Wait73"("Count(uSec)"=w1315) -> ()  [unwired: 1 out]
                }
                frame #18 {
                  n320 = local read "Array 3"() -> (w1320:fxp<+/-,37,27>[])
                  n321 = Index Array(array=w1320, index=9) -> (element=w1317:fxp<+/-,37,27>)
                  n322 = Greater Than 0?(x=w1317) -> (x > 0?=w1318:bool)
                  n323 = xnode "FPGA I/O Node"("Connector0/DIO3"=w1318) -> ()  [unwired: 1 in, 1 out]
                }
                frame #19 {
                  n324 = Absolute Value(x=w1322) -> (abs(x)=w1321:fxp<+,36,26>)
                  n325 = call "Wait74"("Count(uSec)"=w1321) -> ()  [unwired: 1 out]
                }
                frame #20 {
                  # "低"
                  n326 = local read "Array 3"() -> (w1326:fxp<+/-,37,27>[])
                  n327 = Index Array(array=w1326, index=10) -> (element=w1324:fxp<+/-,37,27>)
                  n328 = Greater Than 0?(x=w1324) -> (x > 0?=w1323:bool)
                  n329 = xnode "FPGA I/O Node"("Connector0/DIO3"=w1323) -> ()  [unwired: 1 in, 1 out]
                }
                frame #21 {
                  n330 = Absolute Value(x=w1328) -> (abs(x)=w1327:fxp<+,36,26>)
                  n331 = call "Wait75"("Count(uSec)"=w1327) -> ()  [unwired: 1 out]
                }
                frame #22 {
                  # "高"
                  n332 = local read "Array 3"() -> (w1332:fxp<+/-,37,27>[])
                  n333 = Index Array(array=w1332, index=11) -> (element=w1330:fxp<+/-,37,27>)
                  n334 = Greater Than 0?(x=w1330) -> (x > 0?=w1329:bool)
                  n335 = xnode "FPGA I/O Node"("Connector0/DIO3"=w1329) -> ()  [unwired: 1 in, 1 out]
                }
                frame #23 {
                  n336 = Absolute Value(x=w1334) -> (abs(x)=w1333:fxp<+,36,26>)
                  n337 = call "Wait76"("Count(uSec)"=w1333) -> ()  [unwired: 1 out]
                }
                frame #24 {
                  # "低"
                  n338 = local read "Array 3"() -> (w1338:fxp<+/-,37,27>[])
                  n339 = Index Array(array=w1338, index=12) -> (element=w1336:fxp<+/-,37,27>)
                  n340 = Greater Than 0?(x=w1336) -> (x > 0?=w1335:bool)
                  n341 = xnode "FPGA I/O Node"("Connector0/DIO3"=w1335) -> ()  [unwired: 1 in, 1 out]
                }
                frame #25 {
                  n342 = Absolute Value(x=w1340) -> (abs(x)=w1339:fxp<+,36,26>)
                  n343 = call "Wait77"("Count(uSec)"=w1339) -> ()  [unwired: 1 out]
                }
                frame #26 {
                  # "高"
                  n344 = local read "Array 3"() -> (w1344:fxp<+/-,37,27>[])
                  n345 = Index Array(array=w1344, index=13) -> (element=w1342:fxp<+/-,37,27>)
                  n346 = Greater Than 0?(x=w1342) -> (x > 0?=w1341:bool)
                  n347 = xnode "FPGA I/O Node"("Connector0/DIO3"=w1341) -> ()  [unwired: 1 in, 1 out]
                }
                frame #27 {
                  n348 = Absolute Value(x=w1346) -> (abs(x)=w1345:fxp<+,36,26>)
                  n349 = call "Wait78"("Count(uSec)"=w1345) -> ()  [unwired: 1 out]
                }
                frame #28 {
                  # "低"
                  n350 = local read "Array 3"() -> (w1350:fxp<+/-,37,27>[])
                  n351 = Index Array(array=w1350, index=14) -> (element=w1348:fxp<+/-,37,27>)
                  n352 = Greater Than 0?(x=w1348) -> (x > 0?=w1347:bool)
                  n353 = xnode "FPGA I/O Node"("Connector0/DIO3"=w1347) -> ()  [unwired: 1 in, 1 out]
                }
                frame #29 {
                  n354 = Absolute Value(x=w1352) -> (abs(x)=w1351:fxp<+,36,26>)
                  n355 = call "Wait79"("Count(uSec)"=w1351) -> ()  [unwired: 1 out]
                }
                frame #30 {
                  n356 = local read "Array 3"() -> (w1356:fxp<+/-,37,27>[])
                  n357 = Index Array(array=w1356, index=15) -> (element=w1354:fxp<+/-,37,27>)
                  n358 = Greater Than 0?(x=w1354) -> (x > 0?=w1353:bool)
                  n359 = xnode "FPGA I/O Node"("Connector0/DIO3"=w1353) -> ()  [unwired: 1 in, 1 out]
                }
                frame #31 {
                  n360 = Absolute Value(x=w1358) -> (abs(x)=w1357:fxp<+,36,26>)
                  n361 = call "Wait80"("Count(uSec)"=w1357) -> ()  [unwired: 1 out]
                }
              }
              n362 = flat-sequence "Channel 0" {
                frame #0 {
                  # "第一段电压大小"
                  n363 = local read "AO 0 voltage"() -> (w401:fxp<+/-,32,6>[])
                  n364 = Index Array(array=w401, index=0) -> (element=w399:fxp<+/-,32,6>)
                  n365 = xnode "FPGA I/O Node"("Connector0/AO0"=w399) -> ()  [unwired: 1 in, 1 out]
                }
                frame #1 {
                  # "第一段持续时间"
                  n366 = local read "AO 0 t"() -> (w404:fxp<+/-,37,27>[])
                  n367 = Index Array(array=w404, index=0) -> (element=w402:fxp<+/-,37,27>)
                  n368 = call "Wait2"("Count(uSec)"=w402) -> ()  [unwired: 1 out]
                }
                frame #2 {
                  # "第二段电压大小"
                  n369 = local read "AO 0 voltage"() -> (w406:fxp<+/-,32,6>[])
                  n370 = Index Array(array=w406, index=1) -> (element=w405:fxp<+/-,32,6>)
                  n371 = xnode "FPGA I/O Node"("Connector0/AO0"=w405) -> ()  [unwired: 1 in, 1 out]
                }
                frame #3 {
                  # "第二段持续时间"
                  n372 = local read "AO 0 t"() -> (w409:fxp<+/-,37,27>[])
                  n373 = Index Array(array=w409, index=1) -> (element=w408:fxp<+/-,37,27>)
                  n374 = call "Wait3"("Count(uSec)"=w408) -> ()  [unwired: 1 out]
                }
                frame #4 {
                  # "第三段电压大小"
                  n375 = local read "AO 0 voltage"() -> (w412:fxp<+/-,32,6>[])
                  n376 = Index Array(array=w412, index=2) -> (element=w411:fxp<+/-,32,6>)
                  n377 = xnode "FPGA I/O Node"("Connector0/AO0"=w411) -> ()  [unwired: 1 in, 1 out]
                }
                frame #5 {
                  # "第三段持续时间"
                  n378 = local read "AO 0 t"() -> (w416:fxp<+/-,37,27>[])
                  n379 = Index Array(array=w416, index=2) -> (element=w414:fxp<+/-,37,27>)
                  n380 = call "Wait"("Count(uSec)"=w414) -> ()  [unwired: 1 out]
                }
                frame #6 {
                  # "第四段电压大小"
                  n381 = local read "AO 0 voltage"() -> (w419:fxp<+/-,32,6>[])
                  n382 = Index Array(array=w419, index=3) -> (element=w417:fxp<+/-,32,6>)
                  n383 = xnode ("FPGA I/O Node")("Connector0/AO0"=w417) -> ()  [unwired: 1 in, 1 out]
                }
                frame #7 {
                  # "第四段持续时间"
                  n384 = local read "AO 0 t"() -> (w421:fxp<+/-,37,27>[])
                  n385 = Index Array(array=w421, index=3) -> (element=w420:fxp<+/-,37,27>)
                  n386 = call "Wait4"("Count(uSec)"=w420) -> ()  [unwired: 1 out]
                }
                frame #8 {
                  n387 = local read "AO 0 voltage"() -> (w423:fxp<+/-,32,6>[])
                  n388 = Index Array(array=w423, index=4) -> (element=w424:fxp<+/-,32,6>)
                  n389 = xnode ("FPGA I/O Node")("Connector0/AO0"=w424) -> ()  [unwired: 1 in, 1 out]
                }
                frame #9 {
                  # "5"
                  n390 = local read "AO 0 t"() -> (w426:fxp<+/-,37,27>[])
                  n391 = Index Array(array=w426, index=4) -> (element=w427:fxp<+/-,37,27>)
                  n392 = call "Wait226"("Count(uSec)"=w427) -> ()  [unwired: 1 out]
                }
                frame #10 {
                  n393 = local read "AO 0 voltage"() -> (w429:fxp<+/-,32,6>[])
                  n394 = Index Array(array=w429, index=5) -> (element=w430:fxp<+/-,32,6>)
                  n395 = xnode ("FPGA I/O Node")("Connector0/AO0"=w430) -> ()  [unwired: 1 in, 1 out]
                }
                frame #11 {
                  # "6"
                  n396 = local read "AO 0 t"() -> (w432:fxp<+/-,37,27>[])
                  n397 = Index Array(array=w432, index=5) -> (element=w433:fxp<+/-,37,27>)
                  n398 = call "Wait227"("Count(uSec)"=w433) -> ()  [unwired: 1 out]
                }
                frame #12 {
                  n399 = local read "AO 0 voltage"() -> (w435:fxp<+/-,32,6>[])
                  n400 = Index Array(array=w435, index=6) -> (element=w436:fxp<+/-,32,6>)
                  n401 = xnode ("FPGA I/O Node")("Connector0/AO0"=w436) -> ()  [unwired: 1 in, 1 out]
                }
                frame #13 {
                  # "7"
                  n402 = local read "AO 0 t"() -> (w438:fxp<+/-,37,27>[])
                  n403 = Index Array(array=w438, index=6) -> (element=w439:fxp<+/-,37,27>)
                  n404 = call "Wait228"("Count(uSec)"=w439) -> ()  [unwired: 1 out]
                }
                frame #14 {
                  n405 = local read "AO 0 voltage"() -> (w441:fxp<+/-,32,6>[])
                  n406 = Index Array(array=w441, index=7) -> (element=w442:fxp<+/-,32,6>)
                  n407 = xnode ("FPGA I/O Node")("Connector0/AO0"=w442) -> ()  [unwired: 1 in, 1 out]
                }
                frame #15 {
                  # "8"
                  n408 = local read "AO 0 t"() -> (w444:fxp<+/-,37,27>[])
                  n409 = Index Array(array=w444, index=7) -> (element=w445:fxp<+/-,37,27>)
                  n410 = call "Wait229"("Count(uSec)"=w445) -> ()  [unwired: 1 out]
                }
                frame #16 {
                  n411 = local read "AO 0 voltage"() -> (w447:fxp<+/-,32,6>[])
                  n412 = Index Array(array=w447, index=8) -> (element=w448:fxp<+/-,32,6>)
                  n413 = xnode ("FPGA I/O Node")("Connector0/AO0"=w448) -> ()  [unwired: 1 in, 1 out]
                }
                frame #17 {
                  # "9"
                  n414 = local read "AO 0 t"() -> (w450:fxp<+/-,37,27>[])
                  n415 = Index Array(array=w450, index=8) -> (element=w451:fxp<+/-,37,27>)
                  n416 = call "Wait230"("Count(uSec)"=w451) -> ()  [unwired: 1 out]
                }
                frame #18 {
                  n417 = local read "AO 0 voltage"() -> (w453:fxp<+/-,32,6>[])
                  n418 = Index Array(array=w453, index=9) -> (element=w454:fxp<+/-,32,6>)
                  n419 = xnode ("FPGA I/O Node")("Connector0/AO0"=w454) -> ()  [unwired: 1 in, 1 out]
                }
                frame #19 {
                  # "10"
                  n420 = local read "AO 0 t"() -> (w456:fxp<+/-,37,27>[])
                  n421 = Index Array(array=w456, index=9) -> (element=w457:fxp<+/-,37,27>)
                  n422 = call "Wait231"("Count(uSec)"=w457) -> ()  [unwired: 1 out]
                }
                frame #20 {
                  n423 = local read "AO 0 voltage"() -> (w459:fxp<+/-,32,6>[])
                  n424 = Index Array(array=w459, index=10) -> (element=w460:fxp<+/-,32,6>)
                  n425 = xnode ("FPGA I/O Node")("Connector0/AO0"=w460) -> ()  [unwired: 1 in, 1 out]
                }
                frame #21 {
                  # "11"
                  n426 = local read "AO 0 t"() -> (w462:fxp<+/-,37,27>[])
                  n427 = Index Array(array=w462, index=10) -> (element=w463:fxp<+/-,37,27>)
                  n428 = call "Wait238"("Count(uSec)"=w463) -> ()  [unwired: 1 out]
                }
                frame #22 {
                  n429 = local read "AO 0 voltage"() -> (w465:fxp<+/-,32,6>[])
                  n430 = Index Array(array=w465, index=11) -> (element=w466:fxp<+/-,32,6>)
                  n431 = xnode ("FPGA I/O Node")("Connector0/AO0"=w466) -> ()  [unwired: 1 in, 1 out]
                }
                frame #23 {
                  # "12"
                  n432 = local read "AO 0 t"() -> (w468:fxp<+/-,37,27>[])
                  n433 = Index Array(array=w468, index=11) -> (element=w469:fxp<+/-,37,27>)
                  n434 = call "Wait239"("Count(uSec)"=w469) -> ()  [unwired: 1 out]
                }
                frame #24 {
                  n435 = local read "AO 0 voltage"() -> (w471:fxp<+/-,32,6>[])
                  n436 = Index Array(array=w471, index=12) -> (element=w472:fxp<+/-,32,6>)
                  n437 = xnode ("FPGA I/O Node")("Connector0/AO0"=w472) -> ()  [unwired: 1 in, 1 out]
                }
                frame #25 {
                  # "13"
                  n438 = local read "AO 0 t"() -> (w474:fxp<+/-,37,27>[])
                  n439 = Index Array(array=w474, index=12) -> (element=w475:fxp<+/-,37,27>)
                  n440 = call "Wait240"("Count(uSec)"=w475) -> ()  [unwired: 1 out]
                }
                frame #26 {
                  n441 = local read "AO 0 voltage"() -> (w477:fxp<+/-,32,6>[])
                  n442 = Index Array(array=w477, index=13) -> (element=w478:fxp<+/-,32,6>)
                  n443 = xnode ("FPGA I/O Node")("Connector0/AO0"=w478) -> ()  [unwired: 1 in, 1 out]
                }
                frame #27 {
                  # "14"
                  n444 = local read "AO 0 t"() -> (w480:fxp<+/-,37,27>[])
                  n445 = Index Array(array=w480, index=13) -> (element=w481:fxp<+/-,37,27>)
                  n446 = call "Wait241"("Count(uSec)"=w481) -> ()  [unwired: 1 out]
                }
                frame #28 {
                  n447 = local read "AO 0 voltage"() -> (w483:fxp<+/-,32,6>[])
                  n448 = Index Array(array=w483, index=14) -> (element=w484:fxp<+/-,32,6>)
                  n449 = xnode ("FPGA I/O Node")("Connector0/AO0"=w484) -> ()  [unwired: 1 in, 1 out]
                }
                frame #29 {
                  # "15"
                  n450 = local read "AO 0 t"() -> (w486:fxp<+/-,37,27>[])
                  n451 = Index Array(array=w486, index=14) -> (element=w487:fxp<+/-,37,27>)
                  n452 = call "Wait242"("Count(uSec)"=w487) -> ()  [unwired: 1 out]
                }
                frame #30 {
                  n453 = local read "AO 0 voltage"() -> (w489:fxp<+/-,32,6>[])
                  n454 = Index Array(array=w489, index=15) -> (element=w490:fxp<+/-,32,6>)
                  n455 = xnode ("FPGA I/O Node")("Connector0/AO0"=w490) -> ()  [unwired: 1 in, 1 out]
                }
                frame #31 {
                  # "16"
                  n456 = local read "AO 0 t"() -> (w492:fxp<+/-,37,27>[])
                  n457 = Index Array(array=w492, index=15) -> (element=w493:fxp<+/-,37,27>)
                  n458 = call "Wait243"("Count(uSec)"=w493) -> ()  [unwired: 1 out]
                }
              }
              n459 = flat-sequence "Channel 0" {
                frame #0 {
                  # "第一段电压大小"
                  n460 = local read "AO 1 voltage"() -> (w305:fxp<+/-,32,6>[])
                  n461 = Index Array(array=w305, index=0) -> (element=w303:fxp<+/-,32,6>)
                  n462 = xnode "FPGA I/O Node"("Connector0/AO1"=w303) -> ()  [unwired: 1 in, 1 out]
                }
                frame #1 {
                  # "第一段持续时间"
                  n463 = local read "AO 1 t"() -> (w308:fxp<+/-,37,27>[])
                  n464 = Index Array(array=w308, index=0) -> (element=w306:fxp<+/-,37,27>)
                  n465 = call "Wait5"("Count(uSec)"=w306) -> ()  [unwired: 1 out]
                }
                frame #2 {
                  # "第二段电压大小"
                  n466 = local read "AO 1 voltage"() -> (w310:fxp<+/-,32,6>[])
                  n467 = Index Array(array=w310, index=1) -> (element=w309:fxp<+/-,32,6>)
                  n468 = xnode "FPGA I/O Node"("Connector0/AO1"=w309) -> ()  [unwired: 1 in, 1 out]
                }
                frame #3 {
                  # "第二段持续时间"
                  n469 = local read "AO 1 t"() -> (w313:fxp<+/-,37,27>[])
                  n470 = Index Array(array=w313, index=1) -> (element=w312:fxp<+/-,37,27>)
                  n471 = call "Wait6"("Count(uSec)"=w312) -> ()  [unwired: 1 out]
                }
                frame #4 {
                  # "第三段电压大小"
                  n472 = local read "AO 1 voltage"() -> (w316:fxp<+/-,32,6>[])
                  n473 = Index Array(array=w316, index=2) -> (element=w315:fxp<+/-,32,6>)
                  n474 = xnode "FPGA I/O Node"("Connector0/AO1"=w315) -> ()  [unwired: 1 in, 1 out]
                }
                frame #5 {
                  # "第三段持续时间"
                  n475 = local read "AO 1 t"() -> (w320:fxp<+/-,37,27>[])
                  n476 = Index Array(array=w320, index=2) -> (element=w318:fxp<+/-,37,27>)
                  n477 = call "Wait7"("Count(uSec)"=w318) -> ()  [unwired: 1 out]
                }
                frame #6 {
                  # "第四段电压大小"
                  n478 = local read "AO 1 voltage"() -> (w323:fxp<+/-,32,6>[])
                  n479 = Index Array(array=w323, index=3) -> (element=w321:fxp<+/-,32,6>)
                  n480 = xnode ("FPGA I/O Node")("Connector0/AO1"=w321) -> ()  [unwired: 1 in, 1 out]
                }
                frame #7 {
                  # "第四段持续时间"
                  n481 = local read "AO 1 t"() -> (w325:fxp<+/-,37,27>[])
                  n482 = Index Array(array=w325, index=3) -> (element=w324:fxp<+/-,37,27>)
                  n483 = call "Wait8"("Count(uSec)"=w324) -> ()  [unwired: 1 out]
                }
                frame #8 {
                  n484 = local read "AO 1 voltage"() -> (w327:fxp<+/-,32,6>[])
                  n485 = Index Array(array=w327, index=4) -> (element=w328:fxp<+/-,32,6>)
                  n486 = xnode ("FPGA I/O Node")("Connector0/AO1"=w328) -> ()  [unwired: 1 in, 1 out]
                }
                frame #9 {
                  n487 = local read "AO 1 t"() -> (w330:fxp<+/-,37,27>[])
                  n488 = Index Array(array=w330, index=4) -> (element=w331:fxp<+/-,37,27>)
                  n489 = call "Wait237"("Count(uSec)"=w331) -> ()  [unwired: 1 out]
                }
                frame #10 {
                  n490 = local read "AO 1 voltage"() -> (w333:fxp<+/-,32,6>[])
                  n491 = Index Array(array=w333, index=5) -> (element=w334:fxp<+/-,32,6>)
                  n492 = xnode ("FPGA I/O Node")("Connector0/AO1"=w334) -> ()  [unwired: 1 in, 1 out]
                }
                frame #11 {
                  n493 = local read "AO 1 t"() -> (w336:fxp<+/-,37,27>[])
                  n494 = Index Array(array=w336, index=5) -> (element=w337:fxp<+/-,37,27>)
                  n495 = call "Wait236"("Count(uSec)"=w337) -> ()  [unwired: 1 out]
                }
                frame #12 {
                  n496 = local read "AO 1 voltage"() -> (w339:fxp<+/-,32,6>[])
                  n497 = Index Array(array=w339, index=6) -> (element=w340:fxp<+/-,32,6>)
                  n498 = xnode ("FPGA I/O Node")("Connector0/AO1"=w340) -> ()  [unwired: 1 in, 1 out]
                }
                frame #13 {
                  n499 = local read "AO 1 t"() -> (w342:fxp<+/-,37,27>[])
                  n500 = Index Array(array=w342, index=6) -> (element=w343:fxp<+/-,37,27>)
                  n501 = call "Wait235"("Count(uSec)"=w343) -> ()  [unwired: 1 out]
                }
                frame #14 {
                  n502 = local read "AO 1 voltage"() -> (w345:fxp<+/-,32,6>[])
                  n503 = Index Array(array=w345, index=7) -> (element=w346:fxp<+/-,32,6>)
                  n504 = xnode ("FPGA I/O Node")("Connector0/AO1"=w346) -> ()  [unwired: 1 in, 1 out]
                }
                frame #15 {
                  n505 = local read "AO 1 t"() -> (w348:fxp<+/-,37,27>[])
                  n506 = Index Array(array=w348, index=7) -> (element=w349:fxp<+/-,37,27>)
                  n507 = call "Wait234"("Count(uSec)"=w349) -> ()  [unwired: 1 out]
                }
                frame #16 {
                  n508 = local read "AO 1 voltage"() -> (w351:fxp<+/-,32,6>[])
                  n509 = Index Array(array=w351, index=8) -> (element=w352:fxp<+/-,32,6>)
                  n510 = xnode ("FPGA I/O Node")("Connector0/AO1"=w352) -> ()  [unwired: 1 in, 1 out]
                }
                frame #17 {
                  n511 = local read "AO 1 t"() -> (w354:fxp<+/-,37,27>[])
                  n512 = Index Array(array=w354, index=8) -> (element=w355:fxp<+/-,37,27>)
                  n513 = call "Wait233"("Count(uSec)"=w355) -> ()  [unwired: 1 out]
                }
                frame #18 {
                  n514 = local read "AO 1 voltage"() -> (w357:fxp<+/-,32,6>[])
                  n515 = Index Array(array=w357, index=9) -> (element=w358:fxp<+/-,32,6>)
                  n516 = xnode ("FPGA I/O Node")("Connector0/AO1"=w358) -> ()  [unwired: 1 in, 1 out]
                }
                frame #19 {
                  n517 = local read "AO 1 t"() -> (w360:fxp<+/-,37,27>[])
                  n518 = Index Array(array=w360, index=9) -> (element=w361:fxp<+/-,37,27>)
                  n519 = call "Wait232"("Count(uSec)"=w361) -> ()  [unwired: 1 out]
                }
                frame #20 {
                  n520 = local read "AO 1 voltage"() -> (w363:fxp<+/-,32,6>[])
                  n521 = Index Array(array=w363, index=10) -> (element=w364:fxp<+/-,32,6>)
                  n522 = xnode ("FPGA I/O Node")("Connector0/AO1"=w364) -> ()  [unwired: 1 in, 1 out]
                }
                frame #21 {
                  n523 = local read "AO 1 t"() -> (w366:fxp<+/-,37,27>[])
                  n524 = Index Array(array=w366, index=10) -> (element=w367:fxp<+/-,37,27>)
                  n525 = call "Wait244"("Count(uSec)"=w367) -> ()  [unwired: 1 out]
                }
                frame #22 {
                  n526 = local read "AO 1 voltage"() -> (w369:fxp<+/-,32,6>[])
                  n527 = Index Array(array=w369, index=11) -> (element=w370:fxp<+/-,32,6>)
                  n528 = xnode ("FPGA I/O Node")("Connector0/AO1"=w370) -> ()  [unwired: 1 in, 1 out]
                }
                frame #23 {
                  n529 = local read "AO 1 t"() -> (w372:fxp<+/-,37,27>[])
                  n530 = Index Array(array=w372, index=11) -> (element=w373:fxp<+/-,37,27>)
                  n531 = call "Wait245"("Count(uSec)"=w373) -> ()  [unwired: 1 out]
                }
                frame #24 {
                  n532 = local read "AO 1 voltage"() -> (w375:fxp<+/-,32,6>[])
                  n533 = Index Array(array=w375, index=12) -> (element=w376:fxp<+/-,32,6>)
                  n534 = xnode ("FPGA I/O Node")("Connector0/AO1"=w376) -> ()  [unwired: 1 in, 1 out]
                }
                frame #25 {
                  n535 = local read "AO 1 t"() -> (w378:fxp<+/-,37,27>[])
                  n536 = Index Array(array=w378, index=12) -> (element=w379:fxp<+/-,37,27>)
                  n537 = call "Wait246"("Count(uSec)"=w379) -> ()  [unwired: 1 out]
                }
                frame #26 {
                  n538 = local read "AO 1 voltage"() -> (w381:fxp<+/-,32,6>[])
                  n539 = Index Array(array=w381, index=13) -> (element=w382:fxp<+/-,32,6>)
                  n540 = xnode ("FPGA I/O Node")("Connector0/AO1"=w382) -> ()  [unwired: 1 in, 1 out]
                }
                frame #27 {
                  n541 = local read "AO 1 t"() -> (w384:fxp<+/-,37,27>[])
                  n542 = Index Array(array=w384, index=13) -> (element=w385:fxp<+/-,37,27>)
                  n543 = call "Wait247"("Count(uSec)"=w385) -> ()  [unwired: 1 out]
                }
                frame #28 {
                  n544 = local read "AO 1 voltage"() -> (w387:fxp<+/-,32,6>[])
                  n545 = Index Array(array=w387, index=14) -> (element=w388:fxp<+/-,32,6>)
                  n546 = xnode ("FPGA I/O Node")("Connector0/AO1"=w388) -> ()  [unwired: 1 in, 1 out]
                }
                frame #29 {
                  n547 = local read "AO 1 t"() -> (w390:fxp<+/-,37,27>[])
                  n548 = Index Array(array=w390, index=14) -> (element=w391:fxp<+/-,37,27>)
                  n549 = call "Wait248"("Count(uSec)"=w391) -> ()  [unwired: 1 out]
                }
                frame #30 {
                  n550 = local read "AO 1 voltage"() -> (w393:fxp<+/-,32,6>[])
                  n551 = Index Array(array=w393, index=15) -> (element=w394:fxp<+/-,32,6>)
                  n552 = xnode ("FPGA I/O Node")("Connector0/AO1"=w394) -> ()  [unwired: 1 in, 1 out]
                }
                frame #31 {
                  n553 = local read "AO 1 t"() -> (w396:fxp<+/-,37,27>[])
                  n554 = Index Array(array=w396, index=15) -> (element=w397:fxp<+/-,37,27>)
                  n555 = call "Wait249"("Count(uSec)"=w397) -> ()  [unwired: 1 out]
                }
              }
              n556 = flat-sequence "Channel 3" {
                tunnel: [w1072] -> w190
                tunnel: w190 -> [w1076]
                tunnel: [w1077] -> w189
                tunnel: w189 -> [w1082]
                tunnel: [w1084] -> w188
                tunnel: w188 -> [w1088]
                tunnel: [w1090] -> w187
                tunnel: w187 -> [w1094]
                tunnel: [w1096] -> w186
                tunnel: w186 -> [w1100]
                tunnel: [w1102] -> w185
                tunnel: w185 -> [w1106]
                tunnel: [w1108] -> w184
                tunnel: w184 -> [w1112]
                tunnel: [w1114] -> w183
                tunnel: w183 -> [w1118]
                tunnel: [w1119] -> w182
                tunnel: w182 -> [w1124]
                tunnel: [w1125] -> w181
                tunnel: w181 -> [w1130]
                tunnel: [w1132] -> w180
                tunnel: w180 -> [w1136]
                tunnel: [w1138] -> w179
                tunnel: w179 -> [w1142]
                tunnel: [w1144] -> w178
                tunnel: w178 -> [w1148]
                tunnel: [w1150] -> w177
                tunnel: w177 -> [w1154]
                tunnel: [w1156] -> w176
                tunnel: w176 -> [w1160]
                tunnel: [w1162] -> w175
                tunnel: w175 -> [w1166]
                tunnel: [w1167] -> w93
                tunnel: w93 -> [w1171]
                tunnel: [w1173] -> w90
                tunnel: w90 -> [w1177]
                tunnel: [w1179] -> w74
                tunnel: w74 -> [w1183]
                tunnel: [w1185] -> w73
                tunnel: w73 -> [w1189]
                tunnel: [w1191] -> w72
                tunnel: w72 -> [w1195]
                tunnel: [w1197] -> w71
                tunnel: w71 -> [w1201]
                tunnel: [w1203] -> w70
                tunnel: w70 -> [w1207]
                tunnel: [w1209] -> w69
                tunnel: w69 -> [w1213]
                tunnel: [w1215] -> w61
                tunnel: w61 -> [w1219]
                tunnel: [w1221] -> w68
                tunnel: w68 -> [w1225]
                tunnel: [w1227] -> w67
                tunnel: w67 -> [w1231]
                tunnel: [w1233] -> w66
                tunnel: w66 -> [w1237]
                tunnel: [w1239] -> w65
                tunnel: w65 -> [w1243]
                tunnel: [w1245] -> w64
                tunnel: w64 -> [w1249]
                tunnel: [w1251] -> w63
                tunnel: w63 -> [w1255]
                tunnel: [w1257] -> w62
                tunnel: w62 -> [w1261]
                frame #0 {
                  # "起始电平"
                  n557 = local read "Array 4"() -> (w1074:fxp<+/-,37,27>[])
                  n558 = Index Array(array=w1074, index=0) -> (element=w1072:fxp<+/-,37,27>)
                  n559 = Greater Than 0?(x=w1072) -> (x > 0?=w1071:bool)
                  n560 = xnode "FPGA I/O Node"("Connector0/DIO4"=w1071) -> ()  [unwired: 1 in, 1 out]
                }
                frame #1 {
                  # "第一段持续时间"
                  n561 = Absolute Value(x=w1076) -> (abs(x)=w1075:fxp<+,36,26>)
                  n562 = call "Wait81"("Count(uSec)"=w1075) -> ()  [unwired: 1 out]
                }
                frame #2 {
                  n563 = local read "Array 4"() -> (w1080:fxp<+/-,37,27>[])
                  n564 = Index Array(array=w1080, index=1) -> (element=w1077:fxp<+/-,37,27>)
                  n565 = Greater Than 0?(x=w1077) -> (x > 0?=w1078:bool)
                  n566 = xnode "FPGA I/O Node"("Connector0/DIO4"=w1078) -> ()  [unwired: 1 in, 1 out]
                }
                frame #3 {
                  n567 = Absolute Value(x=w1082) -> (abs(x)=w1081:fxp<+,36,26>)
                  n568 = call "Wait82"("Count(uSec)"=w1081) -> ()  [unwired: 1 out]
                }
                frame #4 {
                  n569 = local read "Array 4"() -> (w1086:fxp<+/-,37,27>[])
                  n570 = Index Array(array=w1086, index=2) -> (element=w1084:fxp<+/-,37,27>)
                  n571 = Greater Than 0?(x=w1084) -> (x > 0?=w1083:bool)
                  n572 = xnode "FPGA I/O Node"("Connector0/DIO4"=w1083) -> ()  [unwired: 1 in, 1 out]
                }
                frame #5 {
                  n573 = Absolute Value(x=w1088) -> (abs(x)=w1087:fxp<+,36,26>)
                  n574 = call "Wait83"("Count(uSec)"=w1087) -> ()  [unwired: 1 out]
                }
                frame #6 {
                  n575 = local read "Array 4"() -> (w1092:fxp<+/-,37,27>[])
                  n576 = Index Array(array=w1092, index=3) -> (element=w1090:fxp<+/-,37,27>)
                  n577 = Greater Than 0?(x=w1090) -> (x > 0?=w1089:bool)
                  n578 = xnode ("FPGA I/O Node")("Connector0/DIO4"=w1089) -> ()  [unwired: 1 in, 1 out]
                }
                frame #7 {
                  n579 = Absolute Value(x=w1094) -> (abs(x)=w1093:fxp<+,36,26>)
                  n580 = call "Wait84"("Count(uSec)"=w1093) -> ()  [unwired: 1 out]
                }
                frame #8 {
                  # "低"
                  n581 = local read "Array 4"() -> (w1098:fxp<+/-,37,27>[])
                  n582 = Index Array(array=w1098, index=4) -> (element=w1096:fxp<+/-,37,27>)
                  n583 = Greater Than 0?(x=w1096) -> (x > 0?=w1095:bool)
                  n584 = xnode "FPGA I/O Node"("Connector0/DIO4"=w1095) -> ()  [unwired: 1 in, 1 out]
                }
                frame #9 {
                  n585 = Absolute Value(x=w1100) -> (abs(x)=w1099:fxp<+,36,26>)
                  n586 = call "Wait85"("Count(uSec)"=w1099) -> ()  [unwired: 1 out]
                }
                frame #10 {
                  # "高"
                  n587 = local read "Array 4"() -> (w1104:fxp<+/-,37,27>[])
                  n588 = Index Array(array=w1104, index=5) -> (element=w1102:fxp<+/-,37,27>)
                  n589 = Greater Than 0?(x=w1102) -> (x > 0?=w1101:bool)
                  n590 = xnode "FPGA I/O Node"("Connector0/DIO4"=w1101) -> ()  [unwired: 1 in, 1 out]
                }
                frame #11 {
                  n591 = Absolute Value(x=w1106) -> (abs(x)=w1105:fxp<+,36,26>)
                  n592 = call "Wait86"("Count(uSec)"=w1105) -> ()  [unwired: 1 out]
                }
                frame #12 {
                  # "低"
                  n593 = local read "Array 4"() -> (w1110:fxp<+/-,37,27>[])
                  n594 = Index Array(array=w1110, index=6) -> (element=w1108:fxp<+/-,37,27>)
                  n595 = Greater Than 0?(x=w1108) -> (x > 0?=w1107:bool)
                  n596 = xnode "FPGA I/O Node"("Connector0/DIO4"=w1107) -> ()  [unwired: 1 in, 1 out]
                }
                frame #13 {
                  n597 = Absolute Value(x=w1112) -> (abs(x)=w1111:fxp<+,36,26>)
                  n598 = call "Wait87"("Count(uSec)"=w1111) -> ()  [unwired: 1 out]
                }
                frame #14 {
                  n599 = local read "Array 4"() -> (w1116:fxp<+/-,37,27>[])
                  n600 = Index Array(array=w1116, index=7) -> (element=w1114:fxp<+/-,37,27>)
                  n601 = Greater Than 0?(x=w1114) -> (x > 0?=w1113:bool)
                  n602 = xnode "FPGA I/O Node"("Connector0/DIO4"=w1113) -> ()  [unwired: 1 in, 1 out]
                }
                frame #15 {
                  n603 = Absolute Value(x=w1118) -> (abs(x)=w1117:fxp<+,36,26>)
                  n604 = call "Wait88"("Count(uSec)"=w1117) -> ()  [unwired: 1 out]
                }
                frame #16 {
                  n605 = local read "Array 4"() -> (w1122:fxp<+/-,37,27>[])
                  n606 = Index Array(array=w1122, index=8) -> (element=w1119:fxp<+/-,37,27>)
                  n607 = Greater Than 0?(x=w1119) -> (x > 0?=w1120:bool)
                  n608 = xnode "FPGA I/O Node"("Connector0/DIO4"=w1120) -> ()  [unwired: 1 in, 1 out]
                }
                frame #17 {
                  n609 = Absolute Value(x=w1124) -> (abs(x)=w1123:fxp<+,36,26>)
                  n610 = call "Wait89"("Count(uSec)"=w1123) -> ()  [unwired: 1 out]
                }
                frame #18 {
                  n611 = local read "Array 4"() -> (w1128:fxp<+/-,37,27>[])
                  n612 = Index Array(array=w1128, index=9) -> (element=w1125:fxp<+/-,37,27>)
                  n613 = Greater Than 0?(x=w1125) -> (x > 0?=w1126:bool)
                  n614 = xnode "FPGA I/O Node"("Connector0/DIO4"=w1126) -> ()  [unwired: 1 in, 1 out]
                }
                frame #19 {
                  n615 = Absolute Value(x=w1130) -> (abs(x)=w1129:fxp<+,36,26>)
                  n616 = call "Wait90"("Count(uSec)"=w1129) -> ()  [unwired: 1 out]
                }
                frame #20 {
                  # "低"
                  n617 = local read "Array 4"() -> (w1134:fxp<+/-,37,27>[])
                  n618 = Index Array(array=w1134, index=10) -> (element=w1132:fxp<+/-,37,27>)
                  n619 = Greater Than 0?(x=w1132) -> (x > 0?=w1131:bool)
                  n620 = xnode "FPGA I/O Node"("Connector0/DIO4"=w1131) -> ()  [unwired: 1 in, 1 out]
                }
                frame #21 {
                  n621 = Absolute Value(x=w1136) -> (abs(x)=w1135:fxp<+,36,26>)
                  n622 = call "Wait91"("Count(uSec)"=w1135) -> ()  [unwired: 1 out]
                }
                frame #22 {
                  # "高"
                  n623 = local read "Array 4"() -> (w1140:fxp<+/-,37,27>[])
                  n624 = Index Array(array=w1140, index=11) -> (element=w1138:fxp<+/-,37,27>)
                  n625 = Greater Than 0?(x=w1138) -> (x > 0?=w1137:bool)
                  n626 = xnode "FPGA I/O Node"("Connector0/DIO4"=w1137) -> ()  [unwired: 1 in, 1 out]
                }
                frame #23 {
                  n627 = Absolute Value(x=w1142) -> (abs(x)=w1141:fxp<+,36,26>)
                  n628 = call "Wait92"("Count(uSec)"=w1141) -> ()  [unwired: 1 out]
                }
                frame #24 {
                  # "低"
                  n629 = local read "Array 4"() -> (w1146:fxp<+/-,37,27>[])
                  n630 = Index Array(array=w1146, index=12) -> (element=w1144:fxp<+/-,37,27>)
                  n631 = Greater Than 0?(x=w1144) -> (x > 0?=w1143:bool)
                  n632 = xnode "FPGA I/O Node"("Connector0/DIO4"=w1143) -> ()  [unwired: 1 in, 1 out]
                }
                frame #25 {
                  n633 = Absolute Value(x=w1148) -> (abs(x)=w1147:fxp<+,36,26>)
                  n634 = call "Wait93"("Count(uSec)"=w1147) -> ()  [unwired: 1 out]
                }
                frame #26 {
                  # "高"
                  n635 = local read "Array 4"() -> (w1152:fxp<+/-,37,27>[])
                  n636 = Index Array(array=w1152, index=13) -> (element=w1150:fxp<+/-,37,27>)
                  n637 = Greater Than 0?(x=w1150) -> (x > 0?=w1149:bool)
                  n638 = xnode "FPGA I/O Node"("Connector0/DIO4"=w1149) -> ()  [unwired: 1 in, 1 out]
                }
                frame #27 {
                  n639 = Absolute Value(x=w1154) -> (abs(x)=w1153:fxp<+,36,26>)
                  n640 = call "Wait94"("Count(uSec)"=w1153) -> ()  [unwired: 1 out]
                }
                frame #28 {
                  # "低"
                  n641 = local read "Array 4"() -> (w1158:fxp<+/-,37,27>[])
                  n642 = Index Array(array=w1158, index=14) -> (element=w1156:fxp<+/-,37,27>)
                  n643 = Greater Than 0?(x=w1156) -> (x > 0?=w1155:bool)
                  n644 = xnode "FPGA I/O Node"("Connector0/DIO4"=w1155) -> ()  [unwired: 1 in, 1 out]
                }
                frame #29 {
                  n645 = Absolute Value(x=w1160) -> (abs(x)=w1159:fxp<+,36,26>)
                  n646 = call "Wait95"("Count(uSec)"=w1159) -> ()  [unwired: 1 out]
                }
                frame #30 {
                  n647 = local read "Array 4"() -> (w1164:fxp<+/-,37,27>[])
                  n648 = Index Array(array=w1164, index=15) -> (element=w1162:fxp<+/-,37,27>)
                  n649 = Greater Than 0?(x=w1162) -> (x > 0?=w1161:bool)
                  n650 = xnode "FPGA I/O Node"("Connector0/DIO4"=w1161) -> ()  [unwired: 1 in, 1 out]
                }
                frame #31 {
                  n651 = Absolute Value(x=w1166) -> (abs(x)=w1165:fxp<+,36,26>)
                  n652 = call "Wait96"("Count(uSec)"=w1165) -> ()  [unwired: 1 out]
                }
                frame #32 {
                  n653 = local read "Array 4"() -> (w1168:fxp<+/-,37,27>[])
                  n654 = Index Array(array=w1168, index=16) -> (element=w1167:fxp<+/-,37,27>)
                  n655 = Greater Than 0?(x=w1167) -> (x > 0?=w1169:bool)
                  n656 = xnode "FPGA I/O Node"("Connector0/DIO4"=w1169) -> ()  [unwired: 1 in, 1 out]
                }
                frame #33 {
                  n657 = Absolute Value(x=w1171) -> (abs(x)=w1172:fxp<+,36,26>)
                  n658 = call "Wait146"("Count(uSec)"=w1172) -> ()  [unwired: 1 out]
                }
                frame #34 {
                  n659 = local read "Array 4"() -> (w1174:fxp<+/-,37,27>[])
                  n660 = Index Array(array=w1174, index=17) -> (element=w1173:fxp<+/-,37,27>)
                  n661 = Greater Than 0?(x=w1173) -> (x > 0?=w1175:bool)
                  n662 = xnode "FPGA I/O Node"("Connector0/DIO4"=w1175) -> ()  [unwired: 1 in, 1 out]
                }
                frame #35 {
                  n663 = Absolute Value(x=w1177) -> (abs(x)=w1178:fxp<+,36,26>)
                  n664 = call "Wait181"("Count(uSec)"=w1178) -> ()  [unwired: 1 out]
                }
                frame #36 {
                  n665 = local read "Array 4"() -> (w1180:fxp<+/-,37,27>[])
                  n666 = Index Array(array=w1180, index=18) -> (element=w1179:fxp<+/-,37,27>)
                  n667 = Greater Than 0?(x=w1179) -> (x > 0?=w1181:bool)
                  n668 = xnode "FPGA I/O Node"("Connector0/DIO4"=w1181) -> ()  [unwired: 1 in, 1 out]
                }
                frame #37 {
                  n669 = Absolute Value(x=w1183) -> (abs(x)=w1184:fxp<+,36,26>)
                  n670 = call "Wait184"("Count(uSec)"=w1184) -> ()  [unwired: 1 out]
                }
                frame #38 {
                  n671 = local read "Array 4"() -> (w1186:fxp<+/-,37,27>[])
                  n672 = Index Array(array=w1186, index=19) -> (element=w1185:fxp<+/-,37,27>)
                  n673 = Greater Than 0?(x=w1185) -> (x > 0?=w1187:bool)
                  n674 = xnode "FPGA I/O Node"("Connector0/DIO4"=w1187) -> ()  [unwired: 1 in, 1 out]
                }
                frame #39 {
                  n675 = Absolute Value(x=w1189) -> (abs(x)=w1190:fxp<+,36,26>)
                  n676 = call "Wait187"("Count(uSec)"=w1190) -> ()  [unwired: 1 out]
                }
                frame #40 {
                  n677 = local read "Array 4"() -> (w1192:fxp<+/-,37,27>[])
                  n678 = Index Array(array=w1192, index=20) -> (element=w1191:fxp<+/-,37,27>)
                  n679 = Greater Than 0?(x=w1191) -> (x > 0?=w1193:bool)
                  n680 = xnode "FPGA I/O Node"("Connector0/DIO4"=w1193) -> ()  [unwired: 1 in, 1 out]
                }
                frame #41 {
                  n681 = Absolute Value(x=w1195) -> (abs(x)=w1196:fxp<+,36,26>)
                  n682 = call "Wait190"("Count(uSec)"=w1196) -> ()  [unwired: 1 out]
                }
                frame #42 {
                  n683 = local read "Array 4"() -> (w1198:fxp<+/-,37,27>[])
                  n684 = Index Array(array=w1198, index=21) -> (element=w1197:fxp<+/-,37,27>)
                  n685 = Greater Than 0?(x=w1197) -> (x > 0?=w1199:bool)
                  n686 = xnode "FPGA I/O Node"("Connector0/DIO4"=w1199) -> ()  [unwired: 1 in, 1 out]
                }
                frame #43 {
                  n687 = Absolute Value(x=w1201) -> (abs(x)=w1202:fxp<+,36,26>)
                  n688 = call "Wait193"("Count(uSec)"=w1202) -> ()  [unwired: 1 out]
                }
                frame #44 {
                  n689 = local read "Array 4"() -> (w1204:fxp<+/-,37,27>[])
                  n690 = Index Array(array=w1204, index=22) -> (element=w1203:fxp<+/-,37,27>)
                  n691 = Greater Than 0?(x=w1203) -> (x > 0?=w1205:bool)
                  n692 = xnode "FPGA I/O Node"("Connector0/DIO4"=w1205) -> ()  [unwired: 1 in, 1 out]
                }
                frame #45 {
                  n693 = Absolute Value(x=w1207) -> (abs(x)=w1208:fxp<+,36,26>)
                  n694 = call "Wait196"("Count(uSec)"=w1208) -> ()  [unwired: 1 out]
                }
                frame #46 {
                  n695 = local read "Array 4"() -> (w1210:fxp<+/-,37,27>[])
                  n696 = Index Array(array=w1210, index=23) -> (element=w1209:fxp<+/-,37,27>)
                  n697 = Greater Than 0?(x=w1209) -> (x > 0?=w1211:bool)
                  n698 = xnode "FPGA I/O Node"("Connector0/DIO4"=w1211) -> ()  [unwired: 1 in, 1 out]
                }
                frame #47 {
                  n699 = Absolute Value(x=w1213) -> (abs(x)=w1214:fxp<+,36,26>)
                  n700 = call "Wait199"("Count(uSec)"=w1214) -> ()  [unwired: 1 out]
                }
                frame #48 {
                  n701 = local read "Array 4"() -> (w1216:fxp<+/-,37,27>[])
                  n702 = Index Array(array=w1216, index=24) -> (element=w1215:fxp<+/-,37,27>)
                  n703 = Greater Than 0?(x=w1215) -> (x > 0?=w1217:bool)
                  n704 = xnode "FPGA I/O Node"("Connector0/DIO4"=w1217) -> ()  [unwired: 1 in, 1 out]
                }
                frame #49 {
                  n705 = Absolute Value(x=w1219) -> (abs(x)=w1220:fxp<+,36,26>)
                  n706 = call "Wait202"("Count(uSec)"=w1220) -> ()  [unwired: 1 out]
                }
                frame #50 {
                  n707 = local read "Array 4"() -> (w1222:fxp<+/-,37,27>[])
                  n708 = Index Array(array=w1222, index=25) -> (element=w1221:fxp<+/-,37,27>)
                  n709 = Greater Than 0?(x=w1221) -> (x > 0?=w1223:bool)
                  n710 = xnode "FPGA I/O Node"("Connector0/DIO4"=w1223) -> ()  [unwired: 1 in, 1 out]
                }
                frame #51 {
                  n711 = Absolute Value(x=w1225) -> (abs(x)=w1226:fxp<+,36,26>)
                  n712 = call "Wait205"("Count(uSec)"=w1226) -> ()  [unwired: 1 out]
                }
                frame #52 {
                  n713 = local read "Array 4"() -> (w1228:fxp<+/-,37,27>[])
                  n714 = Index Array(array=w1228, index=26) -> (element=w1227:fxp<+/-,37,27>)
                  n715 = Greater Than 0?(x=w1227) -> (x > 0?=w1229:bool)
                  n716 = xnode "FPGA I/O Node"("Connector0/DIO4"=w1229) -> ()  [unwired: 1 in, 1 out]
                }
                frame #53 {
                  n717 = Absolute Value(x=w1231) -> (abs(x)=w1232:fxp<+,36,26>)
                  n718 = call "Wait208"("Count(uSec)"=w1232) -> ()  [unwired: 1 out]
                }
                frame #54 {
                  n719 = local read "Array 4"() -> (w1234:fxp<+/-,37,27>[])
                  n720 = Index Array(array=w1234, index=27) -> (element=w1233:fxp<+/-,37,27>)
                  n721 = Greater Than 0?(x=w1233) -> (x > 0?=w1235:bool)
                  n722 = xnode "FPGA I/O Node"("Connector0/DIO4"=w1235) -> ()  [unwired: 1 in, 1 out]
                }
                frame #55 {
                  n723 = Absolute Value(x=w1237) -> (abs(x)=w1238:fxp<+,36,26>)
                  n724 = call "Wait211"("Count(uSec)"=w1238) -> ()  [unwired: 1 out]
                }
                frame #56 {
                  n725 = local read "Array 4"() -> (w1240:fxp<+/-,37,27>[])
                  n726 = Index Array(array=w1240, index=28) -> (element=w1239:fxp<+/-,37,27>)
                  n727 = Greater Than 0?(x=w1239) -> (x > 0?=w1241:bool)
                  n728 = xnode "FPGA I/O Node"("Connector0/DIO4"=w1241) -> ()  [unwired: 1 in, 1 out]
                }
                frame #57 {
                  n729 = Absolute Value(x=w1243) -> (abs(x)=w1244:fxp<+,36,26>)
                  n730 = call "Wait214"("Count(uSec)"=w1244) -> ()  [unwired: 1 out]
                }
                frame #58 {
                  n731 = local read "Array 4"() -> (w1246:fxp<+/-,37,27>[])
                  n732 = Index Array(array=w1246, index=29) -> (element=w1245:fxp<+/-,37,27>)
                  n733 = Greater Than 0?(x=w1245) -> (x > 0?=w1247:bool)
                  n734 = xnode "FPGA I/O Node"("Connector0/DIO4"=w1247) -> ()  [unwired: 1 in, 1 out]
                }
                frame #59 {
                  n735 = Absolute Value(x=w1249) -> (abs(x)=w1250:fxp<+,36,26>)
                  n736 = call "Wait217"("Count(uSec)"=w1250) -> ()  [unwired: 1 out]
                }
                frame #60 {
                  n737 = local read "Array 4"() -> (w1252:fxp<+/-,37,27>[])
                  n738 = Index Array(array=w1252, index=30) -> (element=w1251:fxp<+/-,37,27>)
                  n739 = Greater Than 0?(x=w1251) -> (x > 0?=w1253:bool)
                  n740 = xnode "FPGA I/O Node"("Connector0/DIO4"=w1253) -> ()  [unwired: 1 in, 1 out]
                }
                frame #61 {
                  n741 = Absolute Value(x=w1255) -> (abs(x)=w1256:fxp<+,36,26>)
                  n742 = call "Wait220"("Count(uSec)"=w1256) -> ()  [unwired: 1 out]
                }
                frame #62 {
                  n743 = local read "Array 4"() -> (w1258:fxp<+/-,37,27>[])
                  n744 = Index Array(array=w1258, index=31) -> (element=w1257:fxp<+/-,37,27>)
                  n745 = Greater Than 0?(x=w1257) -> (x > 0?=w1259:bool)
                  n746 = xnode "FPGA I/O Node"("Connector0/DIO4"=w1259) -> ()  [unwired: 1 in, 1 out]
                }
                frame #63 {
                  n747 = Absolute Value(x=w1261) -> (abs(x)=w1262:fxp<+,36,26>)
                  n748 = call "Wait223"("Count(uSec)"=w1262) -> ()  [unwired: 1 out]
                }
              }
              n749 = flat-sequence "Channel 3" {
                tunnel: [w688] -> w158
                tunnel: w158 -> [w692]
                tunnel: [w693] -> w157
                tunnel: w157 -> [w698]
                tunnel: [w700] -> w156
                tunnel: w156 -> [w704]
                tunnel: [w706] -> w155
                tunnel: w155 -> [w710]
                tunnel: [w712] -> w154
                tunnel: w154 -> [w716]
                tunnel: [w718] -> w153
                tunnel: w153 -> [w722]
                tunnel: [w724] -> w152
                tunnel: w152 -> [w728]
                tunnel: [w730] -> w151
                tunnel: w151 -> [w734]
                tunnel: [w735] -> w150
                tunnel: w150 -> [w740]
                tunnel: [w741] -> w149
                tunnel: w149 -> [w746]
                tunnel: [w748] -> w148
                tunnel: w148 -> [w752]
                tunnel: [w754] -> w147
                tunnel: w147 -> [w758]
                tunnel: [w760] -> w146
                tunnel: w146 -> [w764]
                tunnel: [w766] -> w145
                tunnel: w145 -> [w770]
                tunnel: [w772] -> w144
                tunnel: w144 -> [w776]
                tunnel: [w778] -> w143
                tunnel: w143 -> [w782]
                tunnel: [w783] -> w92
                tunnel: w92 -> [w787]
                tunnel: [w789] -> w89
                tunnel: w89 -> [w793]
                tunnel: [w795] -> w88
                tunnel: w88 -> [w799]
                tunnel: [w801] -> w87
                tunnel: w87 -> [w805]
                tunnel: [w807] -> w86
                tunnel: w86 -> [w811]
                tunnel: [w813] -> w85
                tunnel: w85 -> [w817]
                tunnel: [w819] -> w84
                tunnel: w84 -> [w823]
                tunnel: [w825] -> w83
                tunnel: w83 -> [w829]
                tunnel: [w831] -> w82
                tunnel: w82 -> [w835]
                tunnel: [w837] -> w81
                tunnel: w81 -> [w841]
                tunnel: [w843] -> w80
                tunnel: w80 -> [w847]
                tunnel: [w849] -> w79
                tunnel: w79 -> [w853]
                tunnel: [w855] -> w78
                tunnel: w78 -> [w859]
                tunnel: [w861] -> w77
                tunnel: w77 -> [w865]
                tunnel: [w867] -> w76
                tunnel: w76 -> [w871]
                tunnel: [w873] -> w75
                tunnel: w75 -> [w877]
                frame #0 {
                  # "起始电平"
                  n750 = local read "Array 6"() -> (w690:fxp<+/-,37,27>[])
                  n751 = Index Array(array=w690, index=0) -> (element=w688:fxp<+/-,37,27>)
                  n752 = Greater Than 0?(x=w688) -> (x > 0?=w687:bool)
                  n753 = xnode "FPGA I/O Node"("Connector0/DIO6"=w687) -> ()  [unwired: 1 in, 1 out]
                }
                frame #1 {
                  # "第一段持续时间"
                  n754 = Absolute Value(x=w692) -> (abs(x)=w691:fxp<+,36,26>)
                  n755 = call "Wait113"("Count(uSec)"=w691) -> ()  [unwired: 1 out]
                }
                frame #2 {
                  n756 = local read "Array 6"() -> (w696:fxp<+/-,37,27>[])
                  n757 = Index Array(array=w696, index=1) -> (element=w693:fxp<+/-,37,27>)
                  n758 = Greater Than 0?(x=w693) -> (x > 0?=w694:bool)
                  n759 = xnode "FPGA I/O Node"("Connector0/DIO6"=w694) -> ()  [unwired: 1 in, 1 out]
                }
                frame #3 {
                  n760 = Absolute Value(x=w698) -> (abs(x)=w697:fxp<+,36,26>)
                  n761 = call "Wait114"("Count(uSec)"=w697) -> ()  [unwired: 1 out]
                }
                frame #4 {
                  n762 = local read "Array 6"() -> (w702:fxp<+/-,37,27>[])
                  n763 = Index Array(array=w702, index=2) -> (element=w700:fxp<+/-,37,27>)
                  n764 = Greater Than 0?(x=w700) -> (x > 0?=w699:bool)
                  n765 = xnode "FPGA I/O Node"("Connector0/DIO6"=w699) -> ()  [unwired: 1 in, 1 out]
                }
                frame #5 {
                  n766 = Absolute Value(x=w704) -> (abs(x)=w703:fxp<+,36,26>)
                  n767 = call "Wait115"("Count(uSec)"=w703) -> ()  [unwired: 1 out]
                }
                frame #6 {
                  n768 = local read "Array 6"() -> (w708:fxp<+/-,37,27>[])
                  n769 = Index Array(array=w708, index=3) -> (element=w706:fxp<+/-,37,27>)
                  n770 = Greater Than 0?(x=w706) -> (x > 0?=w705:bool)
                  n771 = xnode ("FPGA I/O Node")("Connector0/DIO6"=w705) -> ()  [unwired: 1 in, 1 out]
                }
                frame #7 {
                  n772 = Absolute Value(x=w710) -> (abs(x)=w709:fxp<+,36,26>)
                  n773 = call "Wait116"("Count(uSec)"=w709) -> ()  [unwired: 1 out]
                }
                frame #8 {
                  # "低"
                  n774 = local read "Array 6"() -> (w714:fxp<+/-,37,27>[])
                  n775 = Index Array(array=w714, index=4) -> (element=w712:fxp<+/-,37,27>)
                  n776 = Greater Than 0?(x=w712) -> (x > 0?=w711:bool)
                  n777 = xnode "FPGA I/O Node"("Connector0/DIO6"=w711) -> ()  [unwired: 1 in, 1 out]
                }
                frame #9 {
                  n778 = Absolute Value(x=w716) -> (abs(x)=w715:fxp<+,36,26>)
                  n779 = call "Wait117"("Count(uSec)"=w715) -> ()  [unwired: 1 out]
                }
                frame #10 {
                  # "高"
                  n780 = local read "Array 6"() -> (w720:fxp<+/-,37,27>[])
                  n781 = Index Array(array=w720, index=5) -> (element=w718:fxp<+/-,37,27>)
                  n782 = Greater Than 0?(x=w718) -> (x > 0?=w717:bool)
                  n783 = xnode "FPGA I/O Node"("Connector0/DIO6"=w717) -> ()  [unwired: 1 in, 1 out]
                }
                frame #11 {
                  n784 = Absolute Value(x=w722) -> (abs(x)=w721:fxp<+,36,26>)
                  n785 = call "Wait118"("Count(uSec)"=w721) -> ()  [unwired: 1 out]
                }
                frame #12 {
                  # "低"
                  n786 = local read "Array 6"() -> (w726:fxp<+/-,37,27>[])
                  n787 = Index Array(array=w726, index=6) -> (element=w724:fxp<+/-,37,27>)
                  n788 = Greater Than 0?(x=w724) -> (x > 0?=w723:bool)
                  n789 = xnode "FPGA I/O Node"("Connector0/DIO6"=w723) -> ()  [unwired: 1 in, 1 out]
                }
                frame #13 {
                  n790 = Absolute Value(x=w728) -> (abs(x)=w727:fxp<+,36,26>)
                  n791 = call "Wait119"("Count(uSec)"=w727) -> ()  [unwired: 1 out]
                }
                frame #14 {
                  n792 = local read "Array 6"() -> (w732:fxp<+/-,37,27>[])
                  n793 = Index Array(array=w732, index=7) -> (element=w730:fxp<+/-,37,27>)
                  n794 = Greater Than 0?(x=w730) -> (x > 0?=w729:bool)
                  n795 = xnode "FPGA I/O Node"("Connector0/DIO6"=w729) -> ()  [unwired: 1 in, 1 out]
                }
                frame #15 {
                  n796 = Absolute Value(x=w734) -> (abs(x)=w733:fxp<+,36,26>)
                  n797 = call "Wait120"("Count(uSec)"=w733) -> ()  [unwired: 1 out]
                }
                frame #16 {
                  n798 = local read "Array 6"() -> (w738:fxp<+/-,37,27>[])
                  n799 = Index Array(array=w738, index=8) -> (element=w735:fxp<+/-,37,27>)
                  n800 = Greater Than 0?(x=w735) -> (x > 0?=w736:bool)
                  n801 = xnode "FPGA I/O Node"("Connector0/DIO6"=w736) -> ()  [unwired: 1 in, 1 out]
                }
                frame #17 {
                  n802 = Absolute Value(x=w740) -> (abs(x)=w739:fxp<+,36,26>)
                  n803 = call "Wait121"("Count(uSec)"=w739) -> ()  [unwired: 1 out]
                }
                frame #18 {
                  n804 = local read "Array 6"() -> (w744:fxp<+/-,37,27>[])
                  n805 = Index Array(array=w744, index=9) -> (element=w741:fxp<+/-,37,27>)
                  n806 = Greater Than 0?(x=w741) -> (x > 0?=w742:bool)
                  n807 = xnode "FPGA I/O Node"("Connector0/DIO6"=w742) -> ()  [unwired: 1 in, 1 out]
                }
                frame #19 {
                  n808 = Absolute Value(x=w746) -> (abs(x)=w745:fxp<+,36,26>)
                  n809 = call "Wait122"("Count(uSec)"=w745) -> ()  [unwired: 1 out]
                }
                frame #20 {
                  # "低"
                  n810 = local read "Array 6"() -> (w750:fxp<+/-,37,27>[])
                  n811 = Index Array(array=w750, index=10) -> (element=w748:fxp<+/-,37,27>)
                  n812 = Greater Than 0?(x=w748) -> (x > 0?=w747:bool)
                  n813 = xnode "FPGA I/O Node"("Connector0/DIO6"=w747) -> ()  [unwired: 1 in, 1 out]
                }
                frame #21 {
                  n814 = Absolute Value(x=w752) -> (abs(x)=w751:fxp<+,36,26>)
                  n815 = call "Wait123"("Count(uSec)"=w751) -> ()  [unwired: 1 out]
                }
                frame #22 {
                  # "高"
                  n816 = local read "Array 6"() -> (w756:fxp<+/-,37,27>[])
                  n817 = Index Array(array=w756, index=11) -> (element=w754:fxp<+/-,37,27>)
                  n818 = Greater Than 0?(x=w754) -> (x > 0?=w753:bool)
                  n819 = xnode "FPGA I/O Node"("Connector0/DIO6"=w753) -> ()  [unwired: 1 in, 1 out]
                }
                frame #23 {
                  n820 = Absolute Value(x=w758) -> (abs(x)=w757:fxp<+,36,26>)
                  n821 = call "Wait124"("Count(uSec)"=w757) -> ()  [unwired: 1 out]
                }
                frame #24 {
                  # "低"
                  n822 = local read "Array 6"() -> (w762:fxp<+/-,37,27>[])
                  n823 = Index Array(array=w762, index=12) -> (element=w760:fxp<+/-,37,27>)
                  n824 = Greater Than 0?(x=w760) -> (x > 0?=w759:bool)
                  n825 = xnode "FPGA I/O Node"("Connector0/DIO6"=w759) -> ()  [unwired: 1 in, 1 out]
                }
                frame #25 {
                  n826 = Absolute Value(x=w764) -> (abs(x)=w763:fxp<+,36,26>)
                  n827 = call "Wait125"("Count(uSec)"=w763) -> ()  [unwired: 1 out]
                }
                frame #26 {
                  # "高"
                  n828 = local read "Array 6"() -> (w768:fxp<+/-,37,27>[])
                  n829 = Index Array(array=w768, index=13) -> (element=w766:fxp<+/-,37,27>)
                  n830 = Greater Than 0?(x=w766) -> (x > 0?=w765:bool)
                  n831 = xnode "FPGA I/O Node"("Connector0/DIO6"=w765) -> ()  [unwired: 1 in, 1 out]
                }
                frame #27 {
                  n832 = Absolute Value(x=w770) -> (abs(x)=w769:fxp<+,36,26>)
                  n833 = call "Wait126"("Count(uSec)"=w769) -> ()  [unwired: 1 out]
                }
                frame #28 {
                  # "低"
                  n834 = local read "Array 6"() -> (w774:fxp<+/-,37,27>[])
                  n835 = Index Array(array=w774, index=14) -> (element=w772:fxp<+/-,37,27>)
                  n836 = Greater Than 0?(x=w772) -> (x > 0?=w771:bool)
                  n837 = xnode "FPGA I/O Node"("Connector0/DIO6"=w771) -> ()  [unwired: 1 in, 1 out]
                }
                frame #29 {
                  n838 = Absolute Value(x=w776) -> (abs(x)=w775:fxp<+,36,26>)
                  n839 = call "Wait127"("Count(uSec)"=w775) -> ()  [unwired: 1 out]
                }
                frame #30 {
                  n840 = local read "Array 6"() -> (w780:fxp<+/-,37,27>[])
                  n841 = Index Array(array=w780, index=15) -> (element=w778:fxp<+/-,37,27>)
                  n842 = Greater Than 0?(x=w778) -> (x > 0?=w777:bool)
                  n843 = xnode "FPGA I/O Node"("Connector0/DIO6"=w777) -> ()  [unwired: 1 in, 1 out]
                }
                frame #31 {
                  n844 = Absolute Value(x=w782) -> (abs(x)=w781:fxp<+,36,26>)
                  n845 = call "Wait128"("Count(uSec)"=w781) -> ()  [unwired: 1 out]
                }
                frame #32 {
                  n846 = local read "Array 6"() -> (w784:fxp<+/-,37,27>[])
                  n847 = Index Array(array=w784, index=16) -> (element=w783:fxp<+/-,37,27>)
                  n848 = Greater Than 0?(x=w783) -> (x > 0?=w785:bool)
                  n849 = xnode "FPGA I/O Node"("Connector0/DIO6"=w785) -> ()  [unwired: 1 in, 1 out]
                }
                frame #33 {
                  n850 = Absolute Value(x=w787) -> (abs(x)=w788:fxp<+,36,26>)
                  n851 = call "Wait147"("Count(uSec)"=w788) -> ()  [unwired: 1 out]
                }
                frame #34 {
                  n852 = local read "Array 6"() -> (w790:fxp<+/-,37,27>[])
                  n853 = Index Array(array=w790, index=17) -> (element=w789:fxp<+/-,37,27>)
                  n854 = Greater Than 0?(x=w789) -> (x > 0?=w791:bool)
                  n855 = xnode "FPGA I/O Node"("Connector0/DIO6"=w791) -> ()  [unwired: 1 in, 1 out]
                }
                frame #35 {
                  n856 = Absolute Value(x=w793) -> (abs(x)=w794:fxp<+,36,26>)
                  n857 = call "Wait182"("Count(uSec)"=w794) -> ()  [unwired: 1 out]
                }
                frame #36 {
                  n858 = local read "Array 6"() -> (w796:fxp<+/-,37,27>[])
                  n859 = Index Array(array=w796, index=18) -> (element=w795:fxp<+/-,37,27>)
                  n860 = Greater Than 0?(x=w795) -> (x > 0?=w797:bool)
                  n861 = xnode "FPGA I/O Node"("Connector0/DIO6"=w797) -> ()  [unwired: 1 in, 1 out]
                }
                frame #37 {
                  n862 = Absolute Value(x=w799) -> (abs(x)=w800:fxp<+,36,26>)
                  n863 = call "Wait185"("Count(uSec)"=w800) -> ()  [unwired: 1 out]
                }
                frame #38 {
                  n864 = local read "Array 6"() -> (w802:fxp<+/-,37,27>[])
                  n865 = Index Array(array=w802, index=19) -> (element=w801:fxp<+/-,37,27>)
                  n866 = Greater Than 0?(x=w801) -> (x > 0?=w803:bool)
                  n867 = xnode "FPGA I/O Node"("Connector0/DIO6"=w803) -> ()  [unwired: 1 in, 1 out]
                }
                frame #39 {
                  n868 = Absolute Value(x=w805) -> (abs(x)=w806:fxp<+,36,26>)
                  n869 = call "Wait188"("Count(uSec)"=w806) -> ()  [unwired: 1 out]
                }
                frame #40 {
                  n870 = local read "Array 6"() -> (w808:fxp<+/-,37,27>[])
                  n871 = Index Array(array=w808, index=20) -> (element=w807:fxp<+/-,37,27>)
                  n872 = Greater Than 0?(x=w807) -> (x > 0?=w809:bool)
                  n873 = xnode "FPGA I/O Node"("Connector0/DIO6"=w809) -> ()  [unwired: 1 in, 1 out]
                }
                frame #41 {
                  n874 = Absolute Value(x=w811) -> (abs(x)=w812:fxp<+,36,26>)
                  n875 = call "Wait191"("Count(uSec)"=w812) -> ()  [unwired: 1 out]
                }
                frame #42 {
                  n876 = local read "Array 6"() -> (w814:fxp<+/-,37,27>[])
                  n877 = Index Array(array=w814, index=21) -> (element=w813:fxp<+/-,37,27>)
                  n878 = Greater Than 0?(x=w813) -> (x > 0?=w815:bool)
                  n879 = xnode "FPGA I/O Node"("Connector0/DIO6"=w815) -> ()  [unwired: 1 in, 1 out]
                }
                frame #43 {
                  n880 = Absolute Value(x=w817) -> (abs(x)=w818:fxp<+,36,26>)
                  n881 = call "Wait194"("Count(uSec)"=w818) -> ()  [unwired: 1 out]
                }
                frame #44 {
                  n882 = local read "Array 6"() -> (w820:fxp<+/-,37,27>[])
                  n883 = Index Array(array=w820, index=22) -> (element=w819:fxp<+/-,37,27>)
                  n884 = Greater Than 0?(x=w819) -> (x > 0?=w821:bool)
                  n885 = xnode "FPGA I/O Node"("Connector0/DIO6"=w821) -> ()  [unwired: 1 in, 1 out]
                }
                frame #45 {
                  n886 = Absolute Value(x=w823) -> (abs(x)=w824:fxp<+,36,26>)
                  n887 = call "Wait197"("Count(uSec)"=w824) -> ()  [unwired: 1 out]
                }
                frame #46 {
                  n888 = local read "Array 6"() -> (w826:fxp<+/-,37,27>[])
                  n889 = Index Array(array=w826, index=23) -> (element=w825:fxp<+/-,37,27>)
                  n890 = Greater Than 0?(x=w825) -> (x > 0?=w827:bool)
                  n891 = xnode "FPGA I/O Node"("Connector0/DIO6"=w827) -> ()  [unwired: 1 in, 1 out]
                }
                frame #47 {
                  n892 = Absolute Value(x=w829) -> (abs(x)=w830:fxp<+,36,26>)
                  n893 = call "Wait200"("Count(uSec)"=w830) -> ()  [unwired: 1 out]
                }
                frame #48 {
                  n894 = local read "Array 6"() -> (w832:fxp<+/-,37,27>[])
                  n895 = Index Array(array=w832, index=24) -> (element=w831:fxp<+/-,37,27>)
                  n896 = Greater Than 0?(x=w831) -> (x > 0?=w833:bool)
                  n897 = xnode "FPGA I/O Node"("Connector0/DIO6"=w833) -> ()  [unwired: 1 in, 1 out]
                }
                frame #49 {
                  n898 = Absolute Value(x=w835) -> (abs(x)=w836:fxp<+,36,26>)
                  n899 = call "Wait203"("Count(uSec)"=w836) -> ()  [unwired: 1 out]
                }
                frame #50 {
                  n900 = local read "Array 6"() -> (w838:fxp<+/-,37,27>[])
                  n901 = Index Array(array=w838, index=25) -> (element=w837:fxp<+/-,37,27>)
                  n902 = Greater Than 0?(x=w837) -> (x > 0?=w839:bool)
                  n903 = xnode "FPGA I/O Node"("Connector0/DIO6"=w839) -> ()  [unwired: 1 in, 1 out]
                }
                frame #51 {
                  n904 = Absolute Value(x=w841) -> (abs(x)=w842:fxp<+,36,26>)
                  n905 = call "Wait206"("Count(uSec)"=w842) -> ()  [unwired: 1 out]
                }
                frame #52 {
                  n906 = local read "Array 6"() -> (w844:fxp<+/-,37,27>[])
                  n907 = Index Array(array=w844, index=26) -> (element=w843:fxp<+/-,37,27>)
                  n908 = Greater Than 0?(x=w843) -> (x > 0?=w845:bool)
                  n909 = xnode "FPGA I/O Node"("Connector0/DIO6"=w845) -> ()  [unwired: 1 in, 1 out]
                }
                frame #53 {
                  n910 = Absolute Value(x=w847) -> (abs(x)=w848:fxp<+,36,26>)
                  n911 = call "Wait209"("Count(uSec)"=w848) -> ()  [unwired: 1 out]
                }
                frame #54 {
                  n912 = local read "Array 6"() -> (w850:fxp<+/-,37,27>[])
                  n913 = Index Array(array=w850, index=27) -> (element=w849:fxp<+/-,37,27>)
                  n914 = Greater Than 0?(x=w849) -> (x > 0?=w851:bool)
                  n915 = xnode "FPGA I/O Node"("Connector0/DIO6"=w851) -> ()  [unwired: 1 in, 1 out]
                }
                frame #55 {
                  n916 = Absolute Value(x=w853) -> (abs(x)=w854:fxp<+,36,26>)
                  n917 = call "Wait212"("Count(uSec)"=w854) -> ()  [unwired: 1 out]
                }
                frame #56 {
                  n918 = local read "Array 6"() -> (w856:fxp<+/-,37,27>[])
                  n919 = Index Array(array=w856, index=28) -> (element=w855:fxp<+/-,37,27>)
                  n920 = Greater Than 0?(x=w855) -> (x > 0?=w857:bool)
                  n921 = xnode "FPGA I/O Node"("Connector0/DIO6"=w857) -> ()  [unwired: 1 in, 1 out]
                }
                frame #57 {
                  n922 = Absolute Value(x=w859) -> (abs(x)=w860:fxp<+,36,26>)
                  n923 = call "Wait215"("Count(uSec)"=w860) -> ()  [unwired: 1 out]
                }
                frame #58 {
                  n924 = local read "Array 6"() -> (w862:fxp<+/-,37,27>[])
                  n925 = Index Array(array=w862, index=29) -> (element=w861:fxp<+/-,37,27>)
                  n926 = Greater Than 0?(x=w861) -> (x > 0?=w863:bool)
                  n927 = xnode "FPGA I/O Node"("Connector0/DIO6"=w863) -> ()  [unwired: 1 in, 1 out]
                }
                frame #59 {
                  n928 = Absolute Value(x=w865) -> (abs(x)=w866:fxp<+,36,26>)
                  n929 = call "Wait218"("Count(uSec)"=w866) -> ()  [unwired: 1 out]
                }
                frame #60 {
                  n930 = local read "Array 6"() -> (w868:fxp<+/-,37,27>[])
                  n931 = Index Array(array=w868, index=30) -> (element=w867:fxp<+/-,37,27>)
                  n932 = Greater Than 0?(x=w867) -> (x > 0?=w869:bool)
                  n933 = xnode "FPGA I/O Node"("Connector0/DIO6"=w869) -> ()  [unwired: 1 in, 1 out]
                }
                frame #61 {
                  n934 = Absolute Value(x=w871) -> (abs(x)=w872:fxp<+,36,26>)
                  n935 = call "Wait221"("Count(uSec)"=w872) -> ()  [unwired: 1 out]
                }
                frame #62 {
                  n936 = local read "Array 6"() -> (w874:fxp<+/-,37,27>[])
                  n937 = Index Array(array=w874, index=31) -> (element=w873:fxp<+/-,37,27>)
                  n938 = Greater Than 0?(x=w873) -> (x > 0?=w875:bool)
                  n939 = xnode "FPGA I/O Node"("Connector0/DIO6"=w875) -> ()  [unwired: 1 in, 1 out]
                }
                frame #63 {
                  n940 = Absolute Value(x=w877) -> (abs(x)=w878:fxp<+,36,26>)
                  n941 = call "Wait224"("Count(uSec)"=w878) -> ()  [unwired: 1 out]
                }
              }
              n942 = flat-sequence "Channel 3" {
                tunnel: [w496] -> w142
                tunnel: w142 -> [w500]
                tunnel: [w501] -> w141
                tunnel: w141 -> [w506]
                tunnel: [w508] -> w140
                tunnel: w140 -> [w512]
                tunnel: [w514] -> w139
                tunnel: w139 -> [w518]
                tunnel: [w520] -> w138
                tunnel: w138 -> [w524]
                tunnel: [w526] -> w137
                tunnel: w137 -> [w530]
                tunnel: [w532] -> w136
                tunnel: w136 -> [w536]
                tunnel: [w538] -> w135
                tunnel: w135 -> [w542]
                tunnel: [w543] -> w134
                tunnel: w134 -> [w548]
                tunnel: [w549] -> w133
                tunnel: w133 -> [w554]
                tunnel: [w556] -> w132
                tunnel: w132 -> [w560]
                tunnel: [w562] -> w131
                tunnel: w131 -> [w566]
                tunnel: [w568] -> w130
                tunnel: w130 -> [w572]
                tunnel: [w574] -> w129
                tunnel: w129 -> [w578]
                tunnel: [w580] -> w128
                tunnel: w128 -> [w584]
                tunnel: [w586] -> w127
                tunnel: w127 -> [w590]
                tunnel: [w591] -> w91
                tunnel: w91 -> [w595]
                tunnel: [w597] -> w60
                tunnel: w60 -> [w601]
                tunnel: [w603] -> w59
                tunnel: w59 -> [w607]
                tunnel: [w609] -> w58
                tunnel: w58 -> [w613]
                tunnel: [w615] -> w57
                tunnel: w57 -> [w619]
                tunnel: [w621] -> w56
                tunnel: w56 -> [w625]
                tunnel: [w627] -> w55
                tunnel: w55 -> [w631]
                tunnel: [w633] -> w54
                tunnel: w54 -> [w637]
                tunnel: [w639] -> w53
                tunnel: w53 -> [w643]
                tunnel: [w645] -> w52
                tunnel: w52 -> [w649]
                tunnel: [w651] -> w51
                tunnel: w51 -> [w655]
                tunnel: [w657] -> w50
                tunnel: w50 -> [w661]
                tunnel: [w663] -> w49
                tunnel: w49 -> [w667]
                tunnel: [w669] -> w48
                tunnel: w48 -> [w673]
                tunnel: [w675] -> w47
                tunnel: w47 -> [w679]
                tunnel: [w681] -> w46
                tunnel: w46 -> [w685]
                frame #0 {
                  # "起始电平"
                  n943 = local read "Array 7"() -> (w498:fxp<+/-,37,27>[])
                  n944 = Index Array(array=w498, index=0) -> (element=w496:fxp<+/-,37,27>)
                  n945 = Greater Than 0?(x=w496) -> (x > 0?=w495:bool)
                  n946 = xnode "FPGA I/O Node"("Connector0/DIO7"=w495) -> ()  [unwired: 1 in, 1 out]
                }
                frame #1 {
                  # "第一段持续时间"
                  n947 = Absolute Value(x=w500) -> (abs(x)=w499:fxp<+,36,26>)
                  n948 = call "Wait129"("Count(uSec)"=w499) -> ()  [unwired: 1 out]
                }
                frame #2 {
                  n949 = local read "Array 7"() -> (w504:fxp<+/-,37,27>[])
                  n950 = Index Array(array=w504, index=1) -> (element=w501:fxp<+/-,37,27>)
                  n951 = Greater Than 0?(x=w501) -> (x > 0?=w502:bool)
                  n952 = xnode "FPGA I/O Node"("Connector0/DIO7"=w502) -> ()  [unwired: 1 in, 1 out]
                }
                frame #3 {
                  n953 = Absolute Value(x=w506) -> (abs(x)=w505:fxp<+,36,26>)
                  n954 = call "Wait130"("Count(uSec)"=w505) -> ()  [unwired: 1 out]
                }
                frame #4 {
                  n955 = local read "Array 7"() -> (w510:fxp<+/-,37,27>[])
                  n956 = Index Array(array=w510, index=2) -> (element=w508:fxp<+/-,37,27>)
                  n957 = Greater Than 0?(x=w508) -> (x > 0?=w507:bool)
                  n958 = xnode "FPGA I/O Node"("Connector0/DIO7"=w507) -> ()  [unwired: 1 in, 1 out]
                }
                frame #5 {
                  n959 = Absolute Value(x=w512) -> (abs(x)=w511:fxp<+,36,26>)
                  n960 = call "Wait131"("Count(uSec)"=w511) -> ()  [unwired: 1 out]
                }
                frame #6 {
                  n961 = local read "Array 7"() -> (w516:fxp<+/-,37,27>[])
                  n962 = Index Array(array=w516, index=3) -> (element=w514:fxp<+/-,37,27>)
                  n963 = Greater Than 0?(x=w514) -> (x > 0?=w513:bool)
                  n964 = xnode ("FPGA I/O Node")("Connector0/DIO7"=w513) -> ()  [unwired: 1 in, 1 out]
                }
                frame #7 {
                  n965 = Absolute Value(x=w518) -> (abs(x)=w517:fxp<+,36,26>)
                  n966 = call "Wait132"("Count(uSec)"=w517) -> ()  [unwired: 1 out]
                }
                frame #8 {
                  # "低"
                  n967 = local read "Array 7"() -> (w522:fxp<+/-,37,27>[])
                  n968 = Index Array(array=w522, index=4) -> (element=w520:fxp<+/-,37,27>)
                  n969 = Greater Than 0?(x=w520) -> (x > 0?=w519:bool)
                  n970 = xnode "FPGA I/O Node"("Connector0/DIO7"=w519) -> ()  [unwired: 1 in, 1 out]
                }
                frame #9 {
                  n971 = Absolute Value(x=w524) -> (abs(x)=w523:fxp<+,36,26>)
                  n972 = call "Wait133"("Count(uSec)"=w523) -> ()  [unwired: 1 out]
                }
                frame #10 {
                  # "高"
                  n973 = local read "Array 7"() -> (w528:fxp<+/-,37,27>[])
                  n974 = Index Array(array=w528, index=5) -> (element=w526:fxp<+/-,37,27>)
                  n975 = Greater Than 0?(x=w526) -> (x > 0?=w525:bool)
                  n976 = xnode "FPGA I/O Node"("Connector0/DIO7"=w525) -> ()  [unwired: 1 in, 1 out]
                }
                frame #11 {
                  n977 = Absolute Value(x=w530) -> (abs(x)=w529:fxp<+,36,26>)
                  n978 = call "Wait134"("Count(uSec)"=w529) -> ()  [unwired: 1 out]
                }
                frame #12 {
                  # "低"
                  n979 = local read "Array 7"() -> (w534:fxp<+/-,37,27>[])
                  n980 = Index Array(array=w534, index=6) -> (element=w532:fxp<+/-,37,27>)
                  n981 = Greater Than 0?(x=w532) -> (x > 0?=w531:bool)
                  n982 = xnode "FPGA I/O Node"("Connector0/DIO7"=w531) -> ()  [unwired: 1 in, 1 out]
                }
                frame #13 {
                  n983 = Absolute Value(x=w536) -> (abs(x)=w535:fxp<+,36,26>)
                  n984 = call "Wait135"("Count(uSec)"=w535) -> ()  [unwired: 1 out]
                }
                frame #14 {
                  n985 = local read "Array 7"() -> (w540:fxp<+/-,37,27>[])
                  n986 = Index Array(array=w540, index=7) -> (element=w538:fxp<+/-,37,27>)
                  n987 = Greater Than 0?(x=w538) -> (x > 0?=w537:bool)
                  n988 = xnode "FPGA I/O Node"("Connector0/DIO7"=w537) -> ()  [unwired: 1 in, 1 out]
                }
                frame #15 {
                  n989 = Absolute Value(x=w542) -> (abs(x)=w541:fxp<+,36,26>)
                  n990 = call "Wait136"("Count(uSec)"=w541) -> ()  [unwired: 1 out]
                }
                frame #16 {
                  n991 = local read "Array 7"() -> (w546:fxp<+/-,37,27>[])
                  n992 = Index Array(array=w546, index=8) -> (element=w543:fxp<+/-,37,27>)
                  n993 = Greater Than 0?(x=w543) -> (x > 0?=w544:bool)
                  n994 = xnode "FPGA I/O Node"("Connector0/DIO7"=w544) -> ()  [unwired: 1 in, 1 out]
                }
                frame #17 {
                  n995 = Absolute Value(x=w548) -> (abs(x)=w547:fxp<+,36,26>)
                  n996 = call "Wait137"("Count(uSec)"=w547) -> ()  [unwired: 1 out]
                }
                frame #18 {
                  n997 = local read "Array 7"() -> (w552:fxp<+/-,37,27>[])
                  n998 = Index Array(array=w552, index=9) -> (element=w549:fxp<+/-,37,27>)
                  n999 = Greater Than 0?(x=w549) -> (x > 0?=w550:bool)
                  n1000 = xnode "FPGA I/O Node"("Connector0/DIO7"=w550) -> ()  [unwired: 1 in, 1 out]
                }
                frame #19 {
                  n1001 = Absolute Value(x=w554) -> (abs(x)=w553:fxp<+,36,26>)
                  n1002 = call "Wait138"("Count(uSec)"=w553) -> ()  [unwired: 1 out]
                }
                frame #20 {
                  # "低"
                  n1003 = local read "Array 7"() -> (w558:fxp<+/-,37,27>[])
                  n1004 = Index Array(array=w558, index=10) -> (element=w556:fxp<+/-,37,27>)
                  n1005 = Greater Than 0?(x=w556) -> (x > 0?=w555:bool)
                  n1006 = xnode "FPGA I/O Node"("Connector0/DIO7"=w555) -> ()  [unwired: 1 in, 1 out]
                }
                frame #21 {
                  n1007 = Absolute Value(x=w560) -> (abs(x)=w559:fxp<+,36,26>)
                  n1008 = call "Wait139"("Count(uSec)"=w559) -> ()  [unwired: 1 out]
                }
                frame #22 {
                  # "高"
                  n1009 = local read "Array 7"() -> (w564:fxp<+/-,37,27>[])
                  n1010 = Index Array(array=w564, index=11) -> (element=w562:fxp<+/-,37,27>)
                  n1011 = Greater Than 0?(x=w562) -> (x > 0?=w561:bool)
                  n1012 = xnode "FPGA I/O Node"("Connector0/DIO7"=w561) -> ()  [unwired: 1 in, 1 out]
                }
                frame #23 {
                  n1013 = Absolute Value(x=w566) -> (abs(x)=w565:fxp<+,36,26>)
                  n1014 = call "Wait140"("Count(uSec)"=w565) -> ()  [unwired: 1 out]
                }
                frame #24 {
                  # "低"
                  n1015 = local read "Array 7"() -> (w570:fxp<+/-,37,27>[])
                  n1016 = Index Array(array=w570, index=12) -> (element=w568:fxp<+/-,37,27>)
                  n1017 = Greater Than 0?(x=w568) -> (x > 0?=w567:bool)
                  n1018 = xnode "FPGA I/O Node"("Connector0/DIO7"=w567) -> ()  [unwired: 1 in, 1 out]
                }
                frame #25 {
                  n1019 = Absolute Value(x=w572) -> (abs(x)=w571:fxp<+,36,26>)
                  n1020 = call "Wait141"("Count(uSec)"=w571) -> ()  [unwired: 1 out]
                }
                frame #26 {
                  # "高"
                  n1021 = local read "Array 7"() -> (w576:fxp<+/-,37,27>[])
                  n1022 = Index Array(array=w576, index=13) -> (element=w574:fxp<+/-,37,27>)
                  n1023 = Greater Than 0?(x=w574) -> (x > 0?=w573:bool)
                  n1024 = xnode "FPGA I/O Node"("Connector0/DIO7"=w573) -> ()  [unwired: 1 in, 1 out]
                }
                frame #27 {
                  n1025 = Absolute Value(x=w578) -> (abs(x)=w577:fxp<+,36,26>)
                  n1026 = call "Wait142"("Count(uSec)"=w577) -> ()  [unwired: 1 out]
                }
                frame #28 {
                  # "低"
                  n1027 = local read "Array 7"() -> (w582:fxp<+/-,37,27>[])
                  n1028 = Index Array(array=w582, index=14) -> (element=w580:fxp<+/-,37,27>)
                  n1029 = Greater Than 0?(x=w580) -> (x > 0?=w579:bool)
                  n1030 = xnode "FPGA I/O Node"("Connector0/DIO7"=w579) -> ()  [unwired: 1 in, 1 out]
                }
                frame #29 {
                  n1031 = Absolute Value(x=w584) -> (abs(x)=w583:fxp<+,36,26>)
                  n1032 = call "Wait143"("Count(uSec)"=w583) -> ()  [unwired: 1 out]
                }
                frame #30 {
                  n1033 = local read "Array 7"() -> (w588:fxp<+/-,37,27>[])
                  n1034 = Index Array(array=w588, index=15) -> (element=w586:fxp<+/-,37,27>)
                  n1035 = Greater Than 0?(x=w586) -> (x > 0?=w585:bool)
                  n1036 = xnode "FPGA I/O Node"("Connector0/DIO7"=w585) -> ()  [unwired: 1 in, 1 out]
                }
                frame #31 {
                  n1037 = Absolute Value(x=w590) -> (abs(x)=w589:fxp<+,36,26>)
                  n1038 = call "Wait144"("Count(uSec)"=w589) -> ()  [unwired: 1 out]
                }
                frame #32 {
                  n1039 = local read "Array 7"() -> (w592:fxp<+/-,37,27>[])
                  n1040 = Index Array(array=w592, index=16) -> (element=w591:fxp<+/-,37,27>)
                  n1041 = Greater Than 0?(x=w591) -> (x > 0?=w593:bool)
                  n1042 = xnode "FPGA I/O Node"("Connector0/DIO7"=w593) -> ()  [unwired: 1 in, 1 out]
                }
                frame #33 {
                  n1043 = Absolute Value(x=w595) -> (abs(x)=w596:fxp<+,36,26>)
                  n1044 = call "Wait148"("Count(uSec)"=w596) -> ()  [unwired: 1 out]
                }
                frame #34 {
                  n1045 = local read "Array 7"() -> (w598:fxp<+/-,37,27>[])
                  n1046 = Index Array(array=w598, index=17) -> (element=w597:fxp<+/-,37,27>)
                  n1047 = Greater Than 0?(x=w597) -> (x > 0?=w599:bool)
                  n1048 = xnode "FPGA I/O Node"("Connector0/DIO7"=w599) -> ()  [unwired: 1 in, 1 out]
                }
                frame #35 {
                  n1049 = Absolute Value(x=w601) -> (abs(x)=w602:fxp<+,36,26>)
                  n1050 = call "Wait183"("Count(uSec)"=w602) -> ()  [unwired: 1 out]
                }
                frame #36 {
                  n1051 = local read "Array 7"() -> (w604:fxp<+/-,37,27>[])
                  n1052 = Index Array(array=w604, index=18) -> (element=w603:fxp<+/-,37,27>)
                  n1053 = Greater Than 0?(x=w603) -> (x > 0?=w605:bool)
                  n1054 = xnode "FPGA I/O Node"("Connector0/DIO7"=w605) -> ()  [unwired: 1 in, 1 out]
                }
                frame #37 {
                  n1055 = Absolute Value(x=w607) -> (abs(x)=w608:fxp<+,36,26>)
                  n1056 = call "Wait186"("Count(uSec)"=w608) -> ()  [unwired: 1 out]
                }
                frame #38 {
                  n1057 = local read "Array 7"() -> (w610:fxp<+/-,37,27>[])
                  n1058 = Index Array(array=w610, index=19) -> (element=w609:fxp<+/-,37,27>)
                  n1059 = Greater Than 0?(x=w609) -> (x > 0?=w611:bool)
                  n1060 = xnode "FPGA I/O Node"("Connector0/DIO7"=w611) -> ()  [unwired: 1 in, 1 out]
                }
                frame #39 {
                  n1061 = Absolute Value(x=w613) -> (abs(x)=w614:fxp<+,36,26>)
                  n1062 = call "Wait189"("Count(uSec)"=w614) -> ()  [unwired: 1 out]
                }
                frame #40 {
                  n1063 = local read "Array 7"() -> (w616:fxp<+/-,37,27>[])
                  n1064 = Index Array(array=w616, index=20) -> (element=w615:fxp<+/-,37,27>)
                  n1065 = Greater Than 0?(x=w615) -> (x > 0?=w617:bool)
                  n1066 = xnode "FPGA I/O Node"("Connector0/DIO7"=w617) -> ()  [unwired: 1 in, 1 out]
                }
                frame #41 {
                  n1067 = Absolute Value(x=w619) -> (abs(x)=w620:fxp<+,36,26>)
                  n1068 = call "Wait192"("Count(uSec)"=w620) -> ()  [unwired: 1 out]
                }
                frame #42 {
                  n1069 = local read "Array 7"() -> (w622:fxp<+/-,37,27>[])
                  n1070 = Index Array(array=w622, index=21) -> (element=w621:fxp<+/-,37,27>)
                  n1071 = Greater Than 0?(x=w621) -> (x > 0?=w623:bool)
                  n1072 = xnode "FPGA I/O Node"("Connector0/DIO7"=w623) -> ()  [unwired: 1 in, 1 out]
                }
                frame #43 {
                  n1073 = Absolute Value(x=w625) -> (abs(x)=w626:fxp<+,36,26>)
                  n1074 = call "Wait195"("Count(uSec)"=w626) -> ()  [unwired: 1 out]
                }
                frame #44 {
                  n1075 = local read "Array 7"() -> (w628:fxp<+/-,37,27>[])
                  n1076 = Index Array(array=w628, index=22) -> (element=w627:fxp<+/-,37,27>)
                  n1077 = Greater Than 0?(x=w627) -> (x > 0?=w629:bool)
                  n1078 = xnode "FPGA I/O Node"("Connector0/DIO7"=w629) -> ()  [unwired: 1 in, 1 out]
                }
                frame #45 {
                  n1079 = Absolute Value(x=w631) -> (abs(x)=w632:fxp<+,36,26>)
                  n1080 = call "Wait198"("Count(uSec)"=w632) -> ()  [unwired: 1 out]
                }
                frame #46 {
                  n1081 = local read "Array 7"() -> (w634:fxp<+/-,37,27>[])
                  n1082 = Index Array(array=w634, index=23) -> (element=w633:fxp<+/-,37,27>)
                  n1083 = Greater Than 0?(x=w633) -> (x > 0?=w635:bool)
                  n1084 = xnode "FPGA I/O Node"("Connector0/DIO7"=w635) -> ()  [unwired: 1 in, 1 out]
                }
                frame #47 {
                  n1085 = Absolute Value(x=w637) -> (abs(x)=w638:fxp<+,36,26>)
                  n1086 = call "Wait201"("Count(uSec)"=w638) -> ()  [unwired: 1 out]
                }
                frame #48 {
                  n1087 = local read "Array 7"() -> (w640:fxp<+/-,37,27>[])
                  n1088 = Index Array(array=w640, index=24) -> (element=w639:fxp<+/-,37,27>)
                  n1089 = Greater Than 0?(x=w639) -> (x > 0?=w641:bool)
                  n1090 = xnode "FPGA I/O Node"("Connector0/DIO7"=w641) -> ()  [unwired: 1 in, 1 out]
                }
                frame #49 {
                  n1091 = Absolute Value(x=w643) -> (abs(x)=w644:fxp<+,36,26>)
                  n1092 = call "Wait204"("Count(uSec)"=w644) -> ()  [unwired: 1 out]
                }
                frame #50 {
                  n1093 = local read "Array 7"() -> (w646:fxp<+/-,37,27>[])
                  n1094 = Index Array(array=w646, index=25) -> (element=w645:fxp<+/-,37,27>)
                  n1095 = Greater Than 0?(x=w645) -> (x > 0?=w647:bool)
                  n1096 = xnode "FPGA I/O Node"("Connector0/DIO7"=w647) -> ()  [unwired: 1 in, 1 out]
                }
                frame #51 {
                  n1097 = Absolute Value(x=w649) -> (abs(x)=w650:fxp<+,36,26>)
                  n1098 = call "Wait207"("Count(uSec)"=w650) -> ()  [unwired: 1 out]
                }
                frame #52 {
                  n1099 = local read "Array 7"() -> (w652:fxp<+/-,37,27>[])
                  n1100 = Index Array(array=w652, index=26) -> (element=w651:fxp<+/-,37,27>)
                  n1101 = Greater Than 0?(x=w651) -> (x > 0?=w653:bool)
                  n1102 = xnode "FPGA I/O Node"("Connector0/DIO7"=w653) -> ()  [unwired: 1 in, 1 out]
                }
                frame #53 {
                  n1103 = Absolute Value(x=w655) -> (abs(x)=w656:fxp<+,36,26>)
                  n1104 = call "Wait210"("Count(uSec)"=w656) -> ()  [unwired: 1 out]
                }
                frame #54 {
                  n1105 = local read "Array 7"() -> (w658:fxp<+/-,37,27>[])
                  n1106 = Index Array(array=w658, index=27) -> (element=w657:fxp<+/-,37,27>)
                  n1107 = Greater Than 0?(x=w657) -> (x > 0?=w659:bool)
                  n1108 = xnode "FPGA I/O Node"("Connector0/DIO7"=w659) -> ()  [unwired: 1 in, 1 out]
                }
                frame #55 {
                  n1109 = Absolute Value(x=w661) -> (abs(x)=w662:fxp<+,36,26>)
                  n1110 = call "Wait213"("Count(uSec)"=w662) -> ()  [unwired: 1 out]
                }
                frame #56 {
                  n1111 = local read "Array 7"() -> (w664:fxp<+/-,37,27>[])
                  n1112 = Index Array(array=w664, index=28) -> (element=w663:fxp<+/-,37,27>)
                  n1113 = Greater Than 0?(x=w663) -> (x > 0?=w665:bool)
                  n1114 = xnode "FPGA I/O Node"("Connector0/DIO7"=w665) -> ()  [unwired: 1 in, 1 out]
                }
                frame #57 {
                  n1115 = Absolute Value(x=w667) -> (abs(x)=w668:fxp<+,36,26>)
                  n1116 = call "Wait216"("Count(uSec)"=w668) -> ()  [unwired: 1 out]
                }
                frame #58 {
                  n1117 = local read "Array 7"() -> (w670:fxp<+/-,37,27>[])
                  n1118 = Index Array(array=w670, index=29) -> (element=w669:fxp<+/-,37,27>)
                  n1119 = Greater Than 0?(x=w669) -> (x > 0?=w671:bool)
                  n1120 = xnode "FPGA I/O Node"("Connector0/DIO7"=w671) -> ()  [unwired: 1 in, 1 out]
                }
                frame #59 {
                  n1121 = Absolute Value(x=w673) -> (abs(x)=w674:fxp<+,36,26>)
                  n1122 = call "Wait219"("Count(uSec)"=w674) -> ()  [unwired: 1 out]
                }
                frame #60 {
                  n1123 = local read "Array 7"() -> (w676:fxp<+/-,37,27>[])
                  n1124 = Index Array(array=w676, index=30) -> (element=w675:fxp<+/-,37,27>)
                  n1125 = Greater Than 0?(x=w675) -> (x > 0?=w677:bool)
                  n1126 = xnode "FPGA I/O Node"("Connector0/DIO7"=w677) -> ()  [unwired: 1 in, 1 out]
                }
                frame #61 {
                  n1127 = Absolute Value(x=w679) -> (abs(x)=w680:fxp<+,36,26>)
                  n1128 = call "Wait222"("Count(uSec)"=w680) -> ()  [unwired: 1 out]
                }
                frame #62 {
                  n1129 = local read "Array 7"() -> (w682:fxp<+/-,37,27>[])
                  n1130 = Index Array(array=w682, index=31) -> (element=w681:fxp<+/-,37,27>)
                  n1131 = Greater Than 0?(x=w681) -> (x > 0?=w683:bool)
                  n1132 = xnode "FPGA I/O Node"("Connector0/DIO7"=w683) -> ()  [unwired: 1 in, 1 out]
                }
                frame #63 {
                  n1133 = Absolute Value(x=w685) -> (abs(x)=w686:fxp<+,36,26>)
                  n1134 = call "Wait225"("Count(uSec)"=w686) -> ()  [unwired: 1 out]
                }
              }
              n1135 = flat-sequence "Channel 3" {
                tunnel: [w1456] -> w238
                tunnel: w238 -> [w1460]
                tunnel: [w1461] -> w237
                tunnel: w237 -> [w1466]
                tunnel: [w1468] -> w236
                tunnel: w236 -> [w1472]
                tunnel: [w1474] -> w235
                tunnel: w235 -> [w1478]
                tunnel: [w1480] -> w234
                tunnel: w234 -> [w1484]
                tunnel: [w1486] -> w233
                tunnel: w233 -> [w1490]
                tunnel: [w1492] -> w232
                tunnel: w232 -> [w1496]
                tunnel: [w1498] -> w231
                tunnel: w231 -> [w1502]
                tunnel: [w1503] -> w230
                tunnel: w230 -> [w1508]
                tunnel: [w1509] -> w229
                tunnel: w229 -> [w1514]
                tunnel: [w1516] -> w228
                tunnel: w228 -> [w1520]
                tunnel: [w1522] -> w227
                tunnel: w227 -> [w1526]
                tunnel: [w1528] -> w226
                tunnel: w226 -> [w1532]
                tunnel: [w1534] -> w225
                tunnel: w225 -> [w1538]
                tunnel: [w1540] -> w224
                tunnel: w224 -> [w1544]
                tunnel: [w1546] -> w223
                tunnel: w223 -> [w1550]
                tunnel: [w1551] -> w125
                tunnel: w125 -> [w1555]
                tunnel: [w1557] -> w124
                tunnel: w124 -> [w1561]
                tunnel: [w1563] -> w123
                tunnel: w123 -> [w1567]
                tunnel: [w1569] -> w122
                tunnel: w122 -> [w1573]
                tunnel: [w1575] -> w121
                tunnel: w121 -> [w1579]
                tunnel: [w1581] -> w120
                tunnel: w120 -> [w1585]
                tunnel: [w1587] -> w119
                tunnel: w119 -> [w1591]
                tunnel: [w1593] -> w118
                tunnel: w118 -> [w1597]
                tunnel: [w1599] -> w117
                tunnel: w117 -> [w1603]
                tunnel: [w1605] -> w116
                tunnel: w116 -> [w1609]
                tunnel: [w1611] -> w115
                tunnel: w115 -> [w1615]
                tunnel: [w1617] -> w114
                tunnel: w114 -> [w1621]
                tunnel: [w1623] -> w113
                tunnel: w113 -> [w1627]
                tunnel: [w1629] -> w112
                tunnel: w112 -> [w1633]
                tunnel: [w1635] -> w111
                tunnel: w111 -> [w1639]
                tunnel: [w1641] -> w110
                tunnel: w110 -> [w1645]
                frame #0 {
                  # "起始电平"
                  n1136 = local read "Array 1"() -> (w1458:fxp<+/-,37,27>[])
                  n1137 = Index Array(array=w1458, index=0) -> (element=w1456:fxp<+/-,37,27>)
                  n1138 = Greater Than 0?(x=w1456) -> (x > 0?=w1455:bool)
                  n1139 = xnode "FPGA I/O Node"("Connector0/DIO1"=w1455) -> ()  [unwired: 1 in, 1 out]
                }
                frame #1 {
                  # "第一段持续时间"
                  n1140 = Absolute Value(x=w1460) -> (abs(x)=w1459:fxp<+,36,26>)
                  n1141 = call "Wait33"("Count(uSec)"=w1459) -> ()  [unwired: 1 out]
                }
                frame #2 {
                  n1142 = local read "Array 1"() -> (w1464:fxp<+/-,37,27>[])
                  n1143 = Index Array(array=w1464, index=1) -> (element=w1461:fxp<+/-,37,27>)
                  n1144 = Greater Than 0?(x=w1461) -> (x > 0?=w1462:bool)
                  n1145 = xnode "FPGA I/O Node"("Connector0/DIO1"=w1462) -> ()  [unwired: 1 in, 1 out]
                }
                frame #3 {
                  n1146 = Absolute Value(x=w1466) -> (abs(x)=w1465:fxp<+,36,26>)
                  n1147 = call "Wait34"("Count(uSec)"=w1465) -> ()  [unwired: 1 out]
                }
                frame #4 {
                  n1148 = local read "Array 1"() -> (w1470:fxp<+/-,37,27>[])
                  n1149 = Index Array(array=w1470, index=2) -> (element=w1468:fxp<+/-,37,27>)
                  n1150 = Greater Than 0?(x=w1468) -> (x > 0?=w1467:bool)
                  n1151 = xnode "FPGA I/O Node"("Connector0/DIO1"=w1467) -> ()  [unwired: 1 in, 1 out]
                }
                frame #5 {
                  n1152 = Absolute Value(x=w1472) -> (abs(x)=w1471:fxp<+,36,26>)
                  n1153 = call "Wait35"("Count(uSec)"=w1471) -> ()  [unwired: 1 out]
                }
                frame #6 {
                  n1154 = local read "Array 1"() -> (w1476:fxp<+/-,37,27>[])
                  n1155 = Index Array(array=w1476, index=3) -> (element=w1474:fxp<+/-,37,27>)
                  n1156 = Greater Than 0?(x=w1474) -> (x > 0?=w1473:bool)
                  n1157 = xnode ("FPGA I/O Node")("Connector0/DIO1"=w1473) -> ()  [unwired: 1 in, 1 out]
                }
                frame #7 {
                  n1158 = Absolute Value(x=w1478) -> (abs(x)=w1477:fxp<+,36,26>)
                  n1159 = call "Wait36"("Count(uSec)"=w1477) -> ()  [unwired: 1 out]
                }
                frame #8 {
                  # "低"
                  n1160 = local read "Array 1"() -> (w1482:fxp<+/-,37,27>[])
                  n1161 = Index Array(array=w1482, index=4) -> (element=w1480:fxp<+/-,37,27>)
                  n1162 = Greater Than 0?(x=w1480) -> (x > 0?=w1479:bool)
                  n1163 = xnode "FPGA I/O Node"("Connector0/DIO1"=w1479) -> ()  [unwired: 1 in, 1 out]
                }
                frame #9 {
                  n1164 = Absolute Value(x=w1484) -> (abs(x)=w1483:fxp<+,36,26>)
                  n1165 = call "Wait37"("Count(uSec)"=w1483) -> ()  [unwired: 1 out]
                }
                frame #10 {
                  # "高"
                  n1166 = local read "Array 1"() -> (w1488:fxp<+/-,37,27>[])
                  n1167 = Index Array(array=w1488, index=5) -> (element=w1486:fxp<+/-,37,27>)
                  n1168 = Greater Than 0?(x=w1486) -> (x > 0?=w1485:bool)
                  n1169 = xnode "FPGA I/O Node"("Connector0/DIO1"=w1485) -> ()  [unwired: 1 in, 1 out]
                }
                frame #11 {
                  n1170 = Absolute Value(x=w1490) -> (abs(x)=w1489:fxp<+,36,26>)
                  n1171 = call "Wait38"("Count(uSec)"=w1489) -> ()  [unwired: 1 out]
                }
                frame #12 {
                  # "低"
                  n1172 = local read "Array 1"() -> (w1494:fxp<+/-,37,27>[])
                  n1173 = Index Array(array=w1494, index=6) -> (element=w1492:fxp<+/-,37,27>)
                  n1174 = Greater Than 0?(x=w1492) -> (x > 0?=w1491:bool)
                  n1175 = xnode "FPGA I/O Node"("Connector0/DIO1"=w1491) -> ()  [unwired: 1 in, 1 out]
                }
                frame #13 {
                  n1176 = Absolute Value(x=w1496) -> (abs(x)=w1495:fxp<+,36,26>)
                  n1177 = call "Wait39"("Count(uSec)"=w1495) -> ()  [unwired: 1 out]
                }
                frame #14 {
                  n1178 = local read "Array 1"() -> (w1500:fxp<+/-,37,27>[])
                  n1179 = Index Array(array=w1500, index=7) -> (element=w1498:fxp<+/-,37,27>)
                  n1180 = Greater Than 0?(x=w1498) -> (x > 0?=w1497:bool)
                  n1181 = xnode "FPGA I/O Node"("Connector0/DIO1"=w1497) -> ()  [unwired: 1 in, 1 out]
                }
                frame #15 {
                  n1182 = Absolute Value(x=w1502) -> (abs(x)=w1501:fxp<+,36,26>)
                  n1183 = call "Wait40"("Count(uSec)"=w1501) -> ()  [unwired: 1 out]
                }
                frame #16 {
                  n1184 = local read "Array 1"() -> (w1506:fxp<+/-,37,27>[])
                  n1185 = Index Array(array=w1506, index=8) -> (element=w1503:fxp<+/-,37,27>)
                  n1186 = Greater Than 0?(x=w1503) -> (x > 0?=w1504:bool)
                  n1187 = xnode "FPGA I/O Node"("Connector0/DIO1"=w1504) -> ()  [unwired: 1 in, 1 out]
                }
                frame #17 {
                  n1188 = Absolute Value(x=w1508) -> (abs(x)=w1507:fxp<+,36,26>)
                  n1189 = call "Wait41"("Count(uSec)"=w1507) -> ()  [unwired: 1 out]
                }
                frame #18 {
                  n1190 = local read "Array 1"() -> (w1512:fxp<+/-,37,27>[])
                  n1191 = Index Array(array=w1512, index=9) -> (element=w1509:fxp<+/-,37,27>)
                  n1192 = Greater Than 0?(x=w1509) -> (x > 0?=w1510:bool)
                  n1193 = xnode "FPGA I/O Node"("Connector0/DIO1"=w1510) -> ()  [unwired: 1 in, 1 out]
                }
                frame #19 {
                  n1194 = Absolute Value(x=w1514) -> (abs(x)=w1513:fxp<+,36,26>)
                  n1195 = call "Wait42"("Count(uSec)"=w1513) -> ()  [unwired: 1 out]
                }
                frame #20 {
                  # "低"
                  n1196 = local read "Array 1"() -> (w1518:fxp<+/-,37,27>[])
                  n1197 = Index Array(array=w1518, index=10) -> (element=w1516:fxp<+/-,37,27>)
                  n1198 = Greater Than 0?(x=w1516) -> (x > 0?=w1515:bool)
                  n1199 = xnode "FPGA I/O Node"("Connector0/DIO1"=w1515) -> ()  [unwired: 1 in, 1 out]
                }
                frame #21 {
                  n1200 = Absolute Value(x=w1520) -> (abs(x)=w1519:fxp<+,36,26>)
                  n1201 = call "Wait43"("Count(uSec)"=w1519) -> ()  [unwired: 1 out]
                }
                frame #22 {
                  # "高"
                  n1202 = local read "Array 1"() -> (w1524:fxp<+/-,37,27>[])
                  n1203 = Index Array(array=w1524, index=11) -> (element=w1522:fxp<+/-,37,27>)
                  n1204 = Greater Than 0?(x=w1522) -> (x > 0?=w1521:bool)
                  n1205 = xnode "FPGA I/O Node"("Connector0/DIO1"=w1521) -> ()  [unwired: 1 in, 1 out]
                }
                frame #23 {
                  n1206 = Absolute Value(x=w1526) -> (abs(x)=w1525:fxp<+,36,26>)
                  n1207 = call "Wait44"("Count(uSec)"=w1525) -> ()  [unwired: 1 out]
                }
                frame #24 {
                  # "低"
                  n1208 = local read "Array 1"() -> (w1530:fxp<+/-,37,27>[])
                  n1209 = Index Array(array=w1530, index=12) -> (element=w1528:fxp<+/-,37,27>)
                  n1210 = Greater Than 0?(x=w1528) -> (x > 0?=w1527:bool)
                  n1211 = xnode "FPGA I/O Node"("Connector0/DIO1"=w1527) -> ()  [unwired: 1 in, 1 out]
                }
                frame #25 {
                  n1212 = Absolute Value(x=w1532) -> (abs(x)=w1531:fxp<+,36,26>)
                  n1213 = call "Wait45"("Count(uSec)"=w1531) -> ()  [unwired: 1 out]
                }
                frame #26 {
                  # "高"
                  n1214 = local read "Array 1"() -> (w1536:fxp<+/-,37,27>[])
                  n1215 = Index Array(array=w1536, index=13) -> (element=w1534:fxp<+/-,37,27>)
                  n1216 = Greater Than 0?(x=w1534) -> (x > 0?=w1533:bool)
                  n1217 = xnode "FPGA I/O Node"("Connector0/DIO1"=w1533) -> ()  [unwired: 1 in, 1 out]
                }
                frame #27 {
                  n1218 = Absolute Value(x=w1538) -> (abs(x)=w1537:fxp<+,36,26>)
                  n1219 = call "Wait46"("Count(uSec)"=w1537) -> ()  [unwired: 1 out]
                }
                frame #28 {
                  # "低"
                  n1220 = local read "Array 1"() -> (w1542:fxp<+/-,37,27>[])
                  n1221 = Index Array(array=w1542, index=14) -> (element=w1540:fxp<+/-,37,27>)
                  n1222 = Greater Than 0?(x=w1540) -> (x > 0?=w1539:bool)
                  n1223 = xnode "FPGA I/O Node"("Connector0/DIO1"=w1539) -> ()  [unwired: 1 in, 1 out]
                }
                frame #29 {
                  n1224 = Absolute Value(x=w1544) -> (abs(x)=w1543:fxp<+,36,26>)
                  n1225 = call "Wait47"("Count(uSec)"=w1543) -> ()  [unwired: 1 out]
                }
                frame #30 {
                  n1226 = local read "Array 1"() -> (w1548:fxp<+/-,37,27>[])
                  n1227 = Index Array(array=w1548, index=15) -> (element=w1546:fxp<+/-,37,27>)
                  n1228 = Greater Than 0?(x=w1546) -> (x > 0?=w1545:bool)
                  n1229 = xnode "FPGA I/O Node"("Connector0/DIO1"=w1545) -> ()  [unwired: 1 in, 1 out]
                }
                frame #31 {
                  n1230 = Absolute Value(x=w1550) -> (abs(x)=w1549:fxp<+,36,26>)
                  n1231 = call "Wait48"("Count(uSec)"=w1549) -> ()  [unwired: 1 out]
                }
                frame #32 {
                  n1232 = local read "Array 1"() -> (w1552:fxp<+/-,37,27>[])
                  n1233 = Index Array(array=w1552, index=16) -> (element=w1551:fxp<+/-,37,27>)
                  n1234 = Greater Than 0?(x=w1551) -> (x > 0?=w1553:bool)
                  n1235 = xnode "FPGA I/O Node"("Connector0/DIO1"=w1553) -> ()  [unwired: 1 in, 1 out]
                }
                frame #33 {
                  n1236 = Absolute Value(x=w1555) -> (abs(x)=w1556:fxp<+,36,26>)
                  n1237 = call "Wait149"("Count(uSec)"=w1556) -> ()  [unwired: 1 out]
                }
                frame #34 {
                  n1238 = local read "Array 1"() -> (w1558:fxp<+/-,37,27>[])
                  n1239 = Index Array(array=w1558, index=17) -> (element=w1557:fxp<+/-,37,27>)
                  n1240 = Greater Than 0?(x=w1557) -> (x > 0?=w1559:bool)
                  n1241 = xnode "FPGA I/O Node"("Connector0/DIO1"=w1559) -> ()  [unwired: 1 in, 1 out]
                }
                frame #35 {
                  n1242 = Absolute Value(x=w1561) -> (abs(x)=w1562:fxp<+,36,26>)
                  n1243 = call "Wait150"("Count(uSec)"=w1562) -> ()  [unwired: 1 out]
                }
                frame #36 {
                  n1244 = local read "Array 1"() -> (w1564:fxp<+/-,37,27>[])
                  n1245 = Index Array(array=w1564, index=18) -> (element=w1563:fxp<+/-,37,27>)
                  n1246 = Greater Than 0?(x=w1563) -> (x > 0?=w1565:bool)
                  n1247 = xnode "FPGA I/O Node"("Connector0/DIO1"=w1565) -> ()  [unwired: 1 in, 1 out]
                }
                frame #37 {
                  n1248 = Absolute Value(x=w1567) -> (abs(x)=w1568:fxp<+,36,26>)
                  n1249 = call "Wait151"("Count(uSec)"=w1568) -> ()  [unwired: 1 out]
                }
                frame #38 {
                  n1250 = local read "Array 1"() -> (w1570:fxp<+/-,37,27>[])
                  n1251 = Index Array(array=w1570, index=19) -> (element=w1569:fxp<+/-,37,27>)
                  n1252 = Greater Than 0?(x=w1569) -> (x > 0?=w1571:bool)
                  n1253 = xnode "FPGA I/O Node"("Connector0/DIO1"=w1571) -> ()  [unwired: 1 in, 1 out]
                }
                frame #39 {
                  n1254 = Absolute Value(x=w1573) -> (abs(x)=w1574:fxp<+,36,26>)
                  n1255 = call "Wait152"("Count(uSec)"=w1574) -> ()  [unwired: 1 out]
                }
                frame #40 {
                  n1256 = local read "Array 1"() -> (w1576:fxp<+/-,37,27>[])
                  n1257 = Index Array(array=w1576, index=20) -> (element=w1575:fxp<+/-,37,27>)
                  n1258 = Greater Than 0?(x=w1575) -> (x > 0?=w1577:bool)
                  n1259 = xnode "FPGA I/O Node"("Connector0/DIO1"=w1577) -> ()  [unwired: 1 in, 1 out]
                }
                frame #41 {
                  n1260 = Absolute Value(x=w1579) -> (abs(x)=w1580:fxp<+,36,26>)
                  n1261 = call "Wait153"("Count(uSec)"=w1580) -> ()  [unwired: 1 out]
                }
                frame #42 {
                  n1262 = local read "Array 1"() -> (w1582:fxp<+/-,37,27>[])
                  n1263 = Index Array(array=w1582, index=21) -> (element=w1581:fxp<+/-,37,27>)
                  n1264 = Greater Than 0?(x=w1581) -> (x > 0?=w1583:bool)
                  n1265 = xnode "FPGA I/O Node"("Connector0/DIO1"=w1583) -> ()  [unwired: 1 in, 1 out]
                }
                frame #43 {
                  n1266 = Absolute Value(x=w1585) -> (abs(x)=w1586:fxp<+,36,26>)
                  n1267 = call "Wait154"("Count(uSec)"=w1586) -> ()  [unwired: 1 out]
                }
                frame #44 {
                  n1268 = local read "Array 1"() -> (w1588:fxp<+/-,37,27>[])
                  n1269 = Index Array(array=w1588, index=22) -> (element=w1587:fxp<+/-,37,27>)
                  n1270 = Greater Than 0?(x=w1587) -> (x > 0?=w1589:bool)
                  n1271 = xnode "FPGA I/O Node"("Connector0/DIO1"=w1589) -> ()  [unwired: 1 in, 1 out]
                }
                frame #45 {
                  n1272 = Absolute Value(x=w1591) -> (abs(x)=w1592:fxp<+,36,26>)
                  n1273 = call "Wait155"("Count(uSec)"=w1592) -> ()  [unwired: 1 out]
                }
                frame #46 {
                  n1274 = local read "Array 1"() -> (w1594:fxp<+/-,37,27>[])
                  n1275 = Index Array(array=w1594, index=23) -> (element=w1593:fxp<+/-,37,27>)
                  n1276 = Greater Than 0?(x=w1593) -> (x > 0?=w1595:bool)
                  n1277 = xnode "FPGA I/O Node"("Connector0/DIO1"=w1595) -> ()  [unwired: 1 in, 1 out]
                }
                frame #47 {
                  n1278 = Absolute Value(x=w1597) -> (abs(x)=w1598:fxp<+,36,26>)
                  n1279 = call "Wait156"("Count(uSec)"=w1598) -> ()  [unwired: 1 out]
                }
                frame #48 {
                  n1280 = local read "Array 1"() -> (w1600:fxp<+/-,37,27>[])
                  n1281 = Index Array(array=w1600, index=24) -> (element=w1599:fxp<+/-,37,27>)
                  n1282 = Greater Than 0?(x=w1599) -> (x > 0?=w1601:bool)
                  n1283 = xnode "FPGA I/O Node"("Connector0/DIO1"=w1601) -> ()  [unwired: 1 in, 1 out]
                }
                frame #49 {
                  n1284 = Absolute Value(x=w1603) -> (abs(x)=w1604:fxp<+,36,26>)
                  n1285 = call "Wait157"("Count(uSec)"=w1604) -> ()  [unwired: 1 out]
                }
                frame #50 {
                  n1286 = local read "Array 1"() -> (w1606:fxp<+/-,37,27>[])
                  n1287 = Index Array(array=w1606, index=25) -> (element=w1605:fxp<+/-,37,27>)
                  n1288 = Greater Than 0?(x=w1605) -> (x > 0?=w1607:bool)
                  n1289 = xnode "FPGA I/O Node"("Connector0/DIO1"=w1607) -> ()  [unwired: 1 in, 1 out]
                }
                frame #51 {
                  n1290 = Absolute Value(x=w1609) -> (abs(x)=w1610:fxp<+,36,26>)
                  n1291 = call "Wait158"("Count(uSec)"=w1610) -> ()  [unwired: 1 out]
                }
                frame #52 {
                  n1292 = local read "Array 1"() -> (w1612:fxp<+/-,37,27>[])
                  n1293 = Index Array(array=w1612, index=26) -> (element=w1611:fxp<+/-,37,27>)
                  n1294 = Greater Than 0?(x=w1611) -> (x > 0?=w1613:bool)
                  n1295 = xnode "FPGA I/O Node"("Connector0/DIO1"=w1613) -> ()  [unwired: 1 in, 1 out]
                }
                frame #53 {
                  n1296 = Absolute Value(x=w1615) -> (abs(x)=w1616:fxp<+,36,26>)
                  n1297 = call "Wait159"("Count(uSec)"=w1616) -> ()  [unwired: 1 out]
                }
                frame #54 {
                  n1298 = local read "Array 1"() -> (w1618:fxp<+/-,37,27>[])
                  n1299 = Index Array(array=w1618, index=27) -> (element=w1617:fxp<+/-,37,27>)
                  n1300 = Greater Than 0?(x=w1617) -> (x > 0?=w1619:bool)
                  n1301 = xnode "FPGA I/O Node"("Connector0/DIO1"=w1619) -> ()  [unwired: 1 in, 1 out]
                }
                frame #55 {
                  n1302 = Absolute Value(x=w1621) -> (abs(x)=w1622:fxp<+,36,26>)
                  n1303 = call "Wait160"("Count(uSec)"=w1622) -> ()  [unwired: 1 out]
                }
                frame #56 {
                  n1304 = local read "Array 1"() -> (w1624:fxp<+/-,37,27>[])
                  n1305 = Index Array(array=w1624, index=28) -> (element=w1623:fxp<+/-,37,27>)
                  n1306 = Greater Than 0?(x=w1623) -> (x > 0?=w1625:bool)
                  n1307 = xnode "FPGA I/O Node"("Connector0/DIO1"=w1625) -> ()  [unwired: 1 in, 1 out]
                }
                frame #57 {
                  n1308 = Absolute Value(x=w1627) -> (abs(x)=w1628:fxp<+,36,26>)
                  n1309 = call "Wait161"("Count(uSec)"=w1628) -> ()  [unwired: 1 out]
                }
                frame #58 {
                  n1310 = local read "Array 1"() -> (w1630:fxp<+/-,37,27>[])
                  n1311 = Index Array(array=w1630, index=29) -> (element=w1629:fxp<+/-,37,27>)
                  n1312 = Greater Than 0?(x=w1629) -> (x > 0?=w1631:bool)
                  n1313 = xnode "FPGA I/O Node"("Connector0/DIO1"=w1631) -> ()  [unwired: 1 in, 1 out]
                }
                frame #59 {
                  n1314 = Absolute Value(x=w1633) -> (abs(x)=w1634:fxp<+,36,26>)
                  n1315 = call "Wait162"("Count(uSec)"=w1634) -> ()  [unwired: 1 out]
                }
                frame #60 {
                  n1316 = local read "Array 1"() -> (w1636:fxp<+/-,37,27>[])
                  n1317 = Index Array(array=w1636, index=30) -> (element=w1635:fxp<+/-,37,27>)
                  n1318 = Greater Than 0?(x=w1635) -> (x > 0?=w1637:bool)
                  n1319 = xnode "FPGA I/O Node"("Connector0/DIO1"=w1637) -> ()  [unwired: 1 in, 1 out]
                }
                frame #61 {
                  n1320 = Absolute Value(x=w1639) -> (abs(x)=w1640:fxp<+,36,26>)
                  n1321 = call "Wait163"("Count(uSec)"=w1640) -> ()  [unwired: 1 out]
                }
                frame #62 {
                  n1322 = local read "Array 1"() -> (w1642:fxp<+/-,37,27>[])
                  n1323 = Index Array(array=w1642, index=31) -> (element=w1641:fxp<+/-,37,27>)
                  n1324 = Greater Than 0?(x=w1641) -> (x > 0?=w1643:bool)
                  n1325 = xnode "FPGA I/O Node"("Connector0/DIO1"=w1643) -> ()  [unwired: 1 in, 1 out]
                }
                frame #63 {
                  n1326 = Absolute Value(x=w1645) -> (abs(x)=w1646:fxp<+,36,26>)
                  n1327 = call "Wait164"("Count(uSec)"=w1646) -> ()  [unwired: 1 out]
                }
              }
              n1328 = flat-sequence "Channel 3" {
                tunnel: [w880] -> w174
                tunnel: w174 -> [w884]
                tunnel: [w885] -> w173
                tunnel: w173 -> [w890]
                tunnel: [w892] -> w172
                tunnel: w172 -> [w896]
                tunnel: [w898] -> w171
                tunnel: w171 -> [w902]
                tunnel: [w904] -> w170
                tunnel: w170 -> [w908]
                tunnel: [w910] -> w169
                tunnel: w169 -> [w914]
                tunnel: [w916] -> w168
                tunnel: w168 -> [w920]
                tunnel: [w922] -> w167
                tunnel: w167 -> [w926]
                tunnel: [w927] -> w166
                tunnel: w166 -> [w932]
                tunnel: [w933] -> w165
                tunnel: w165 -> [w938]
                tunnel: [w940] -> w164
                tunnel: w164 -> [w944]
                tunnel: [w946] -> w163
                tunnel: w163 -> [w950]
                tunnel: [w952] -> w162
                tunnel: w162 -> [w956]
                tunnel: [w958] -> w161
                tunnel: w161 -> [w962]
                tunnel: [w964] -> w160
                tunnel: w160 -> [w968]
                tunnel: [w970] -> w159
                tunnel: w159 -> [w974]
                tunnel: [w975] -> w94
                tunnel: w94 -> [w979]
                tunnel: [w981] -> w95
                tunnel: w95 -> [w985]
                tunnel: [w987] -> w96
                tunnel: w96 -> [w991]
                tunnel: [w993] -> w97
                tunnel: w97 -> [w997]
                tunnel: [w999] -> w98
                tunnel: w98 -> [w1003]
                tunnel: [w1005] -> w99
                tunnel: w99 -> [w1009]
                tunnel: [w1011] -> w100
                tunnel: w100 -> [w1015]
                tunnel: [w1017] -> w101
                tunnel: w101 -> [w1021]
                tunnel: [w1023] -> w102
                tunnel: w102 -> [w1027]
                tunnel: [w1029] -> w103
                tunnel: w103 -> [w1033]
                tunnel: [w1035] -> w104
                tunnel: w104 -> [w1039]
                tunnel: [w1041] -> w105
                tunnel: w105 -> [w1045]
                tunnel: [w1047] -> w106
                tunnel: w106 -> [w1051]
                tunnel: [w1053] -> w107
                tunnel: w107 -> [w1057]
                tunnel: [w1059] -> w108
                tunnel: w108 -> [w1063]
                tunnel: [w1065] -> w109
                tunnel: w109 -> [w1069]
                frame #0 {
                  # "起始电平"
                  n1329 = local read "Array 5"() -> (w882:fxp<+/-,37,27>[])
                  n1330 = Index Array(array=w882, index=0) -> (element=w880:fxp<+/-,37,27>)
                  n1331 = Greater Than 0?(x=w880) -> (x > 0?=w879:bool)
                  n1332 = xnode "FPGA I/O Node"("Connector0/DIO5"=w879) -> ()  [unwired: 1 in, 1 out]
                }
                frame #1 {
                  # "第一段持续时间"
                  n1333 = Absolute Value(x=w884) -> (abs(x)=w883:fxp<+,36,26>)
                  n1334 = call "Wait97"("Count(uSec)"=w883) -> ()  [unwired: 1 out]
                }
                frame #2 {
                  n1335 = local read "Array 5"() -> (w888:fxp<+/-,37,27>[])
                  n1336 = Index Array(array=w888, index=1) -> (element=w885:fxp<+/-,37,27>)
                  n1337 = Greater Than 0?(x=w885) -> (x > 0?=w886:bool)
                  n1338 = xnode "FPGA I/O Node"("Connector0/DIO5"=w886) -> ()  [unwired: 1 in, 1 out]
                }
                frame #3 {
                  n1339 = Absolute Value(x=w890) -> (abs(x)=w889:fxp<+,36,26>)
                  n1340 = call "Wait98"("Count(uSec)"=w889) -> ()  [unwired: 1 out]
                }
                frame #4 {
                  n1341 = local read "Array 5"() -> (w894:fxp<+/-,37,27>[])
                  n1342 = Index Array(array=w894, index=2) -> (element=w892:fxp<+/-,37,27>)
                  n1343 = Greater Than 0?(x=w892) -> (x > 0?=w891:bool)
                  n1344 = xnode "FPGA I/O Node"("Connector0/DIO5"=w891) -> ()  [unwired: 1 in, 1 out]
                }
                frame #5 {
                  n1345 = Absolute Value(x=w896) -> (abs(x)=w895:fxp<+,36,26>)
                  n1346 = call "Wait99"("Count(uSec)"=w895) -> ()  [unwired: 1 out]
                }
                frame #6 {
                  n1347 = local read "Array 5"() -> (w900:fxp<+/-,37,27>[])
                  n1348 = Index Array(array=w900, index=3) -> (element=w898:fxp<+/-,37,27>)
                  n1349 = Greater Than 0?(x=w898) -> (x > 0?=w897:bool)
                  n1350 = xnode ("FPGA I/O Node")("Connector0/DIO5"=w897) -> ()  [unwired: 1 in, 1 out]
                }
                frame #7 {
                  n1351 = Absolute Value(x=w902) -> (abs(x)=w901:fxp<+,36,26>)
                  n1352 = call "Wait100"("Count(uSec)"=w901) -> ()  [unwired: 1 out]
                }
                frame #8 {
                  # "低"
                  n1353 = local read "Array 5"() -> (w906:fxp<+/-,37,27>[])
                  n1354 = Index Array(array=w906, index=4) -> (element=w904:fxp<+/-,37,27>)
                  n1355 = Greater Than 0?(x=w904) -> (x > 0?=w903:bool)
                  n1356 = xnode "FPGA I/O Node"("Connector0/DIO5"=w903) -> ()  [unwired: 1 in, 1 out]
                }
                frame #9 {
                  n1357 = Absolute Value(x=w908) -> (abs(x)=w907:fxp<+,36,26>)
                  n1358 = call "Wait101"("Count(uSec)"=w907) -> ()  [unwired: 1 out]
                }
                frame #10 {
                  # "高"
                  n1359 = local read "Array 5"() -> (w912:fxp<+/-,37,27>[])
                  n1360 = Index Array(array=w912, index=5) -> (element=w910:fxp<+/-,37,27>)
                  n1361 = Greater Than 0?(x=w910) -> (x > 0?=w909:bool)
                  n1362 = xnode "FPGA I/O Node"("Connector0/DIO5"=w909) -> ()  [unwired: 1 in, 1 out]
                }
                frame #11 {
                  n1363 = Absolute Value(x=w914) -> (abs(x)=w913:fxp<+,36,26>)
                  n1364 = call "Wait102"("Count(uSec)"=w913) -> ()  [unwired: 1 out]
                }
                frame #12 {
                  # "低"
                  n1365 = local read "Array 5"() -> (w918:fxp<+/-,37,27>[])
                  n1366 = Index Array(array=w918, index=6) -> (element=w916:fxp<+/-,37,27>)
                  n1367 = Greater Than 0?(x=w916) -> (x > 0?=w915:bool)
                  n1368 = xnode "FPGA I/O Node"("Connector0/DIO5"=w915) -> ()  [unwired: 1 in, 1 out]
                }
                frame #13 {
                  n1369 = Absolute Value(x=w920) -> (abs(x)=w919:fxp<+,36,26>)
                  n1370 = call "Wait103"("Count(uSec)"=w919) -> ()  [unwired: 1 out]
                }
                frame #14 {
                  n1371 = local read "Array 5"() -> (w924:fxp<+/-,37,27>[])
                  n1372 = Index Array(array=w924, index=7) -> (element=w922:fxp<+/-,37,27>)
                  n1373 = Greater Than 0?(x=w922) -> (x > 0?=w921:bool)
                  n1374 = xnode "FPGA I/O Node"("Connector0/DIO5"=w921) -> ()  [unwired: 1 in, 1 out]
                }
                frame #15 {
                  n1375 = Absolute Value(x=w926) -> (abs(x)=w925:fxp<+,36,26>)
                  n1376 = call "Wait104"("Count(uSec)"=w925) -> ()  [unwired: 1 out]
                }
                frame #16 {
                  n1377 = local read "Array 5"() -> (w930:fxp<+/-,37,27>[])
                  n1378 = Index Array(array=w930, index=8) -> (element=w927:fxp<+/-,37,27>)
                  n1379 = Greater Than 0?(x=w927) -> (x > 0?=w928:bool)
                  n1380 = xnode "FPGA I/O Node"("Connector0/DIO5"=w928) -> ()  [unwired: 1 in, 1 out]
                }
                frame #17 {
                  n1381 = Absolute Value(x=w932) -> (abs(x)=w931:fxp<+,36,26>)
                  n1382 = call "Wait105"("Count(uSec)"=w931) -> ()  [unwired: 1 out]
                }
                frame #18 {
                  n1383 = local read "Array 5"() -> (w936:fxp<+/-,37,27>[])
                  n1384 = Index Array(array=w936, index=9) -> (element=w933:fxp<+/-,37,27>)
                  n1385 = Greater Than 0?(x=w933) -> (x > 0?=w934:bool)
                  n1386 = xnode "FPGA I/O Node"("Connector0/DIO5"=w934) -> ()  [unwired: 1 in, 1 out]
                }
                frame #19 {
                  n1387 = Absolute Value(x=w938) -> (abs(x)=w937:fxp<+,36,26>)
                  n1388 = call "Wait106"("Count(uSec)"=w937) -> ()  [unwired: 1 out]
                }
                frame #20 {
                  # "低"
                  n1389 = local read "Array 5"() -> (w942:fxp<+/-,37,27>[])
                  n1390 = Index Array(array=w942, index=10) -> (element=w940:fxp<+/-,37,27>)
                  n1391 = Greater Than 0?(x=w940) -> (x > 0?=w939:bool)
                  n1392 = xnode "FPGA I/O Node"("Connector0/DIO5"=w939) -> ()  [unwired: 1 in, 1 out]
                }
                frame #21 {
                  n1393 = Absolute Value(x=w944) -> (abs(x)=w943:fxp<+,36,26>)
                  n1394 = call "Wait107"("Count(uSec)"=w943) -> ()  [unwired: 1 out]
                }
                frame #22 {
                  # "高"
                  n1395 = local read "Array 5"() -> (w948:fxp<+/-,37,27>[])
                  n1396 = Index Array(array=w948, index=11) -> (element=w946:fxp<+/-,37,27>)
                  n1397 = Greater Than 0?(x=w946) -> (x > 0?=w945:bool)
                  n1398 = xnode "FPGA I/O Node"("Connector0/DIO5"=w945) -> ()  [unwired: 1 in, 1 out]
                }
                frame #23 {
                  n1399 = Absolute Value(x=w950) -> (abs(x)=w949:fxp<+,36,26>)
                  n1400 = call "Wait108"("Count(uSec)"=w949) -> ()  [unwired: 1 out]
                }
                frame #24 {
                  # "低"
                  n1401 = local read "Array 5"() -> (w954:fxp<+/-,37,27>[])
                  n1402 = Index Array(array=w954, index=12) -> (element=w952:fxp<+/-,37,27>)
                  n1403 = Greater Than 0?(x=w952) -> (x > 0?=w951:bool)
                  n1404 = xnode "FPGA I/O Node"("Connector0/DIO5"=w951) -> ()  [unwired: 1 in, 1 out]
                }
                frame #25 {
                  n1405 = Absolute Value(x=w956) -> (abs(x)=w955:fxp<+,36,26>)
                  n1406 = call "Wait109"("Count(uSec)"=w955) -> ()  [unwired: 1 out]
                }
                frame #26 {
                  # "高"
                  n1407 = local read "Array 5"() -> (w960:fxp<+/-,37,27>[])
                  n1408 = Index Array(array=w960, index=13) -> (element=w958:fxp<+/-,37,27>)
                  n1409 = Greater Than 0?(x=w958) -> (x > 0?=w957:bool)
                  n1410 = xnode "FPGA I/O Node"("Connector0/DIO5"=w957) -> ()  [unwired: 1 in, 1 out]
                }
                frame #27 {
                  n1411 = Absolute Value(x=w962) -> (abs(x)=w961:fxp<+,36,26>)
                  n1412 = call "Wait110"("Count(uSec)"=w961) -> ()  [unwired: 1 out]
                }
                frame #28 {
                  # "低"
                  n1413 = local read "Array 5"() -> (w966:fxp<+/-,37,27>[])
                  n1414 = Index Array(array=w966, index=14) -> (element=w964:fxp<+/-,37,27>)
                  n1415 = Greater Than 0?(x=w964) -> (x > 0?=w963:bool)
                  n1416 = xnode "FPGA I/O Node"("Connector0/DIO5"=w963) -> ()  [unwired: 1 in, 1 out]
                }
                frame #29 {
                  n1417 = Absolute Value(x=w968) -> (abs(x)=w967:fxp<+,36,26>)
                  n1418 = call "Wait111"("Count(uSec)"=w967) -> ()  [unwired: 1 out]
                }
                frame #30 {
                  n1419 = local read "Array 5"() -> (w972:fxp<+/-,37,27>[])
                  n1420 = Index Array(array=w972, index=15) -> (element=w970:fxp<+/-,37,27>)
                  n1421 = Greater Than 0?(x=w970) -> (x > 0?=w969:bool)
                  n1422 = xnode "FPGA I/O Node"("Connector0/DIO5"=w969) -> ()  [unwired: 1 in, 1 out]
                }
                frame #31 {
                  n1423 = Absolute Value(x=w974) -> (abs(x)=w973:fxp<+,36,26>)
                  n1424 = call "Wait112"("Count(uSec)"=w973) -> ()  [unwired: 1 out]
                }
                frame #32 {
                  n1425 = local read "Array 5"() -> (w976:fxp<+/-,37,27>[])
                  n1426 = Index Array(array=w976, index=16) -> (element=w975:fxp<+/-,37,27>)
                  n1427 = Greater Than 0?(x=w975) -> (x > 0?=w977:bool)
                  n1428 = xnode "FPGA I/O Node"("Connector0/DIO5"=w977) -> ()  [unwired: 1 in, 1 out]
                }
                frame #33 {
                  n1429 = Absolute Value(x=w979) -> (abs(x)=w980:fxp<+,36,26>)
                  n1430 = call "Wait165"("Count(uSec)"=w980) -> ()  [unwired: 1 out]
                }
                frame #34 {
                  n1431 = local read "Array 5"() -> (w982:fxp<+/-,37,27>[])
                  n1432 = Index Array(array=w982, index=17) -> (element=w981:fxp<+/-,37,27>)
                  n1433 = Greater Than 0?(x=w981) -> (x > 0?=w983:bool)
                  n1434 = xnode "FPGA I/O Node"("Connector0/DIO5"=w983) -> ()  [unwired: 1 in, 1 out]
                }
                frame #35 {
                  n1435 = Absolute Value(x=w985) -> (abs(x)=w986:fxp<+,36,26>)
                  n1436 = call "Wait166"("Count(uSec)"=w986) -> ()  [unwired: 1 out]
                }
                frame #36 {
                  n1437 = local read "Array 5"() -> (w988:fxp<+/-,37,27>[])
                  n1438 = Index Array(array=w988, index=18) -> (element=w987:fxp<+/-,37,27>)
                  n1439 = Greater Than 0?(x=w987) -> (x > 0?=w989:bool)
                  n1440 = xnode "FPGA I/O Node"("Connector0/DIO5"=w989) -> ()  [unwired: 1 in, 1 out]
                }
                frame #37 {
                  n1441 = Absolute Value(x=w991) -> (abs(x)=w992:fxp<+,36,26>)
                  n1442 = call "Wait167"("Count(uSec)"=w992) -> ()  [unwired: 1 out]
                }
                frame #38 {
                  n1443 = local read "Array 5"() -> (w994:fxp<+/-,37,27>[])
                  n1444 = Index Array(array=w994, index=19) -> (element=w993:fxp<+/-,37,27>)
                  n1445 = Greater Than 0?(x=w993) -> (x > 0?=w995:bool)
                  n1446 = xnode "FPGA I/O Node"("Connector0/DIO5"=w995) -> ()  [unwired: 1 in, 1 out]
                }
                frame #39 {
                  n1447 = Absolute Value(x=w997) -> (abs(x)=w998:fxp<+,36,26>)
                  n1448 = call "Wait168"("Count(uSec)"=w998) -> ()  [unwired: 1 out]
                }
                frame #40 {
                  n1449 = local read "Array 5"() -> (w1000:fxp<+/-,37,27>[])
                  n1450 = Index Array(array=w1000, index=20) -> (element=w999:fxp<+/-,37,27>)
                  n1451 = Greater Than 0?(x=w999) -> (x > 0?=w1001:bool)
                  n1452 = xnode "FPGA I/O Node"("Connector0/DIO5"=w1001) -> ()  [unwired: 1 in, 1 out]
                }
                frame #41 {
                  n1453 = Absolute Value(x=w1003) -> (abs(x)=w1004:fxp<+,36,26>)
                  n1454 = call "Wait169"("Count(uSec)"=w1004) -> ()  [unwired: 1 out]
                }
                frame #42 {
                  n1455 = local read "Array 5"() -> (w1006:fxp<+/-,37,27>[])
                  n1456 = Index Array(array=w1006, index=21) -> (element=w1005:fxp<+/-,37,27>)
                  n1457 = Greater Than 0?(x=w1005) -> (x > 0?=w1007:bool)
                  n1458 = xnode "FPGA I/O Node"("Connector0/DIO5"=w1007) -> ()  [unwired: 1 in, 1 out]
                }
                frame #43 {
                  n1459 = Absolute Value(x=w1009) -> (abs(x)=w1010:fxp<+,36,26>)
                  n1460 = call "Wait170"("Count(uSec)"=w1010) -> ()  [unwired: 1 out]
                }
                frame #44 {
                  n1461 = local read "Array 5"() -> (w1012:fxp<+/-,37,27>[])
                  n1462 = Index Array(array=w1012, index=22) -> (element=w1011:fxp<+/-,37,27>)
                  n1463 = Greater Than 0?(x=w1011) -> (x > 0?=w1013:bool)
                  n1464 = xnode "FPGA I/O Node"("Connector0/DIO5"=w1013) -> ()  [unwired: 1 in, 1 out]
                }
                frame #45 {
                  n1465 = Absolute Value(x=w1015) -> (abs(x)=w1016:fxp<+,36,26>)
                  n1466 = call "Wait171"("Count(uSec)"=w1016) -> ()  [unwired: 1 out]
                }
                frame #46 {
                  n1467 = local read "Array 5"() -> (w1018:fxp<+/-,37,27>[])
                  n1468 = Index Array(array=w1018, index=23) -> (element=w1017:fxp<+/-,37,27>)
                  n1469 = Greater Than 0?(x=w1017) -> (x > 0?=w1019:bool)
                  n1470 = xnode "FPGA I/O Node"("Connector0/DIO5"=w1019) -> ()  [unwired: 1 in, 1 out]
                }
                frame #47 {
                  n1471 = Absolute Value(x=w1021) -> (abs(x)=w1022:fxp<+,36,26>)
                  n1472 = call "Wait172"("Count(uSec)"=w1022) -> ()  [unwired: 1 out]
                }
                frame #48 {
                  n1473 = local read "Array 5"() -> (w1024:fxp<+/-,37,27>[])
                  n1474 = Index Array(array=w1024, index=24) -> (element=w1023:fxp<+/-,37,27>)
                  n1475 = Greater Than 0?(x=w1023) -> (x > 0?=w1025:bool)
                  n1476 = xnode "FPGA I/O Node"("Connector0/DIO5"=w1025) -> ()  [unwired: 1 in, 1 out]
                }
                frame #49 {
                  n1477 = Absolute Value(x=w1027) -> (abs(x)=w1028:fxp<+,36,26>)
                  n1478 = call "Wait173"("Count(uSec)"=w1028) -> ()  [unwired: 1 out]
                }
                frame #50 {
                  n1479 = local read "Array 5"() -> (w1030:fxp<+/-,37,27>[])
                  n1480 = Index Array(array=w1030, index=25) -> (element=w1029:fxp<+/-,37,27>)
                  n1481 = Greater Than 0?(x=w1029) -> (x > 0?=w1031:bool)
                  n1482 = xnode "FPGA I/O Node"("Connector0/DIO5"=w1031) -> ()  [unwired: 1 in, 1 out]
                }
                frame #51 {
                  n1483 = Absolute Value(x=w1033) -> (abs(x)=w1034:fxp<+,36,26>)
                  n1484 = call "Wait174"("Count(uSec)"=w1034) -> ()  [unwired: 1 out]
                }
                frame #52 {
                  n1485 = local read "Array 5"() -> (w1036:fxp<+/-,37,27>[])
                  n1486 = Index Array(array=w1036, index=26) -> (element=w1035:fxp<+/-,37,27>)
                  n1487 = Greater Than 0?(x=w1035) -> (x > 0?=w1037:bool)
                  n1488 = xnode "FPGA I/O Node"("Connector0/DIO5"=w1037) -> ()  [unwired: 1 in, 1 out]
                }
                frame #53 {
                  n1489 = Absolute Value(x=w1039) -> (abs(x)=w1040:fxp<+,36,26>)
                  n1490 = call "Wait175"("Count(uSec)"=w1040) -> ()  [unwired: 1 out]
                }
                frame #54 {
                  n1491 = local read "Array 5"() -> (w1042:fxp<+/-,37,27>[])
                  n1492 = Index Array(array=w1042, index=27) -> (element=w1041:fxp<+/-,37,27>)
                  n1493 = Greater Than 0?(x=w1041) -> (x > 0?=w1043:bool)
                  n1494 = xnode "FPGA I/O Node"("Connector0/DIO5"=w1043) -> ()  [unwired: 1 in, 1 out]
                }
                frame #55 {
                  n1495 = Absolute Value(x=w1045) -> (abs(x)=w1046:fxp<+,36,26>)
                  n1496 = call "Wait176"("Count(uSec)"=w1046) -> ()  [unwired: 1 out]
                }
                frame #56 {
                  n1497 = local read "Array 5"() -> (w1048:fxp<+/-,37,27>[])
                  n1498 = Index Array(array=w1048, index=28) -> (element=w1047:fxp<+/-,37,27>)
                  n1499 = Greater Than 0?(x=w1047) -> (x > 0?=w1049:bool)
                  n1500 = xnode "FPGA I/O Node"("Connector0/DIO5"=w1049) -> ()  [unwired: 1 in, 1 out]
                }
                frame #57 {
                  n1501 = Absolute Value(x=w1051) -> (abs(x)=w1052:fxp<+,36,26>)
                  n1502 = call "Wait177"("Count(uSec)"=w1052) -> ()  [unwired: 1 out]
                }
                frame #58 {
                  n1503 = local read "Array 5"() -> (w1054:fxp<+/-,37,27>[])
                  n1504 = Index Array(array=w1054, index=29) -> (element=w1053:fxp<+/-,37,27>)
                  n1505 = Greater Than 0?(x=w1053) -> (x > 0?=w1055:bool)
                  n1506 = xnode "FPGA I/O Node"("Connector0/DIO5"=w1055) -> ()  [unwired: 1 in, 1 out]
                }
                frame #59 {
                  n1507 = Absolute Value(x=w1057) -> (abs(x)=w1058:fxp<+,36,26>)
                  n1508 = call "Wait178"("Count(uSec)"=w1058) -> ()  [unwired: 1 out]
                }
                frame #60 {
                  n1509 = local read "Array 5"() -> (w1060:fxp<+/-,37,27>[])
                  n1510 = Index Array(array=w1060, index=30) -> (element=w1059:fxp<+/-,37,27>)
                  n1511 = Greater Than 0?(x=w1059) -> (x > 0?=w1061:bool)
                  n1512 = xnode "FPGA I/O Node"("Connector0/DIO5"=w1061) -> ()  [unwired: 1 in, 1 out]
                }
                frame #61 {
                  n1513 = Absolute Value(x=w1063) -> (abs(x)=w1064:fxp<+,36,26>)
                  n1514 = call "Wait179"("Count(uSec)"=w1064) -> ()  [unwired: 1 out]
                }
                frame #62 {
                  n1515 = local read "Array 5"() -> (w1066:fxp<+/-,37,27>[])
                  n1516 = Index Array(array=w1066, index=31) -> (element=w1065:fxp<+/-,37,27>)
                  n1517 = Greater Than 0?(x=w1065) -> (x > 0?=w1067:bool)
                  n1518 = xnode "FPGA I/O Node"("Connector0/DIO5"=w1067) -> ()  [unwired: 1 in, 1 out]
                }
                frame #63 {
                  n1519 = Absolute Value(x=w1069) -> (abs(x)=w1070:fxp<+,36,26>)
                  n1520 = call "Wait180"("Count(uSec)"=w1070) -> ()  [unwired: 1 out]
                }
              }
              n1521 = call "Wait145"("Count(uSec)"=w126) -> ()  [unwired: 1 out]
            }
          }
        }
      }
    }
  }
